vi "TLB Native Dynamic Events ver 0.23.vi"() -> ()   [LabVIEW 2018]
uses:
  Labview Training Phase 2/Enum Controls/States for Action Engine.ctl
  TLB Type Definitions/State Type Definitions, for 0.26g versions and later 2.ctl
  TLB Type Definitions/Intruction Type Definitions.ctl
  TLB Type Definitions/Encoder cluster.ctl
  TLB Type Definitions/PING CLUSTER.ctl
  <vilib>/Studica/Studica Toolkit/NavX/NavX.lvlib
  <vilib>/Studica/Studica Toolkit/Background/DIO Channel.ctl
  Underlying VI's/NavX VI/navX type def.ctl
  <vilib>/Studica/Studica Toolkit/Background/I2C Channel.ctl
  TLB Type Definitions/Vision cluster.ctl
  <vilib>/NI_Real-Time Target Support.lvlib
  TLB Type Definitions/Stepper cluster.ctl
  Experimental VI's/Archived VI's/MOTOR CONTROL NO PID Type Def.ctl
  Underlying VI's/I2C Master VI/I2C MASTER Type Def.ctl
  Underlying VI's/I2C Master VI/I2C_MASTER_WRITE_NEW Type Def.ctl
  <vilib>/userdefined/High Color/IMAQdx.ctl
  Underlying VI's/I2C Master VI/Arduino_Interfacing.ctl
  TLB Type Definitions/Yaw Cluster.ctl
  TLB Type Definitions/Time cluster.ctl
  TLB Type Definitions/Y Stepper cluster.ctl
  Underlying VI's/Modified webcam FGV/Webcam AE.ctl
  Underlying VI's/Elasped Timer/Elapsed timer control.ctl
  Underlying VI's/Motor Control VI with PID/MOTOR CONTROL WITH PID AE DATA MODE TYPE DEF.ctl
  Underlying VI's/Motor Control VI with PID/MOTOR CONTROL WITH PID AE DIRECTION TYPE DEF.ctl
  TLB Type Definitions/IR Sensor Type Def.ctl
  <vilib>/myRIO/Common/Instrument Driver Framework/myRIO v1.0/AI/typedefs/AI Channels Enum.ctl
  <vilib>/myRIO/Common/Instrument Driver Framework/myRIO v1.0/AI/typedefs/AI Channels List.ctl
  TLB Type Definitions/Motor Speed Cluster.ctl
  Underlying VI's/IMAQ Create Reference AE/IMAQ Reference AE.ctl
  TLB Type Definitions/Line Sensor Cluster.ctl
  Underlying VI's/Line Sensor AE/Line Sensor AE Type Def.ctl
  <vilib>/Studica/Studica Toolkit/NavX/TypeDefs/Flags/Z900_navX_Flags_CalibrationStatusTypeDef.ctl
  <vilib>/Studica/Studica Toolkit/NavX/TypeDefs/Flags/Z900_navX_Flags_OpStatusTypeDef.ctl
panel:
  out "Front Wall detected":bool
  out "CPU 1 Usage":dbl
  out "CPU 0 Usage":dbl
  out "Line sensors":T1
  out "IR Sensors":T2
  out "Time up":T3
  out "NAVX Values":T4
  out "Stepper position values":T5
  out "Encoder values":T6
  out "Ultrasonic sensors":T7
  out "Stop?":bool
  out "Selected Task":T8=enum."Start Task 9"
  out "Object recognition mode":enum16{"Ball", "Soap", "Gel", "Pipe", "None"}(ring)
  out "Correcte stepper":u8
  out "Image Processing Error":errorcluster
  out "Object Detection":T9
  out "Status":T12 {"OP Status" items=["INITIALIZING", "SELFTEST_IN_PROGRESS", "ERROR", "IMU_AUTOCAL_IN_PROGRESS", "NORMAL"]; "Calibration Status" items=["IMU_CAL_STATE_MASK"=3, "IMU_CAL_STATE_INPROGRESS"=0, "IMU_CAL_STATE_ACCUMULATE"=1, "IMU_CAL_STATE_COMPLETE"=2]}
  out "General Errors":errorcluster
  in  "Red LED":bool
  out "Table obstruct":bool
  out "x-y":dbl
  out "Obstacle detected":bool
  out "Speed & distance":T13
  out "Task selection":u8
  out "NavX Readings":T14
  out "Arduino Data":T15
  out "TASK ENABLE":bool
  out "Rising Edge":bool
  in  "Green LED":bool
  out "State Logic":T16=enum."Startup"
  out "elements":T8[](array[typedef])
  in  "STOP TASK":bool
  in  "OK Button":bool
  in  "STOP":bool
  out "Queue Errors":errorcluster
  out "Action Queue Items":i32
  out "State Logic Queue Items":i32
  out "Action Queues items":string[](array[string])=["Hardware reset", "Software reset", ""]
  out "Action State":string
  # "VISION"
  # "TLB FRAMEWORK STATUS"
  # "System Health Status Update"
  # "Test Programme written by Calvin Loke    Dated: 28 Aug 2019\nTest Programme revised by Dr Alex See   Dated 30 Aug 2019\n\nRevision date: 20/03/2020\nProgramme version:   TLB Native Dynamic Events ver 0.19a"
  # "0: Task 1\n1: Task 2\n2: Task 3\n3: Task 4\n4: Task 5\n5: Task 6\n6: Task 7\n7: Task 8 Ball\n8: Task 8 Soap\n9: Task 8 Gel\n10: Task 8 Pipe\n11: Task 9 Blue\n12: Task 9 Black\n13: Task 9 Green\n14: Task 9 Red\n15: Task 9 Yellow"
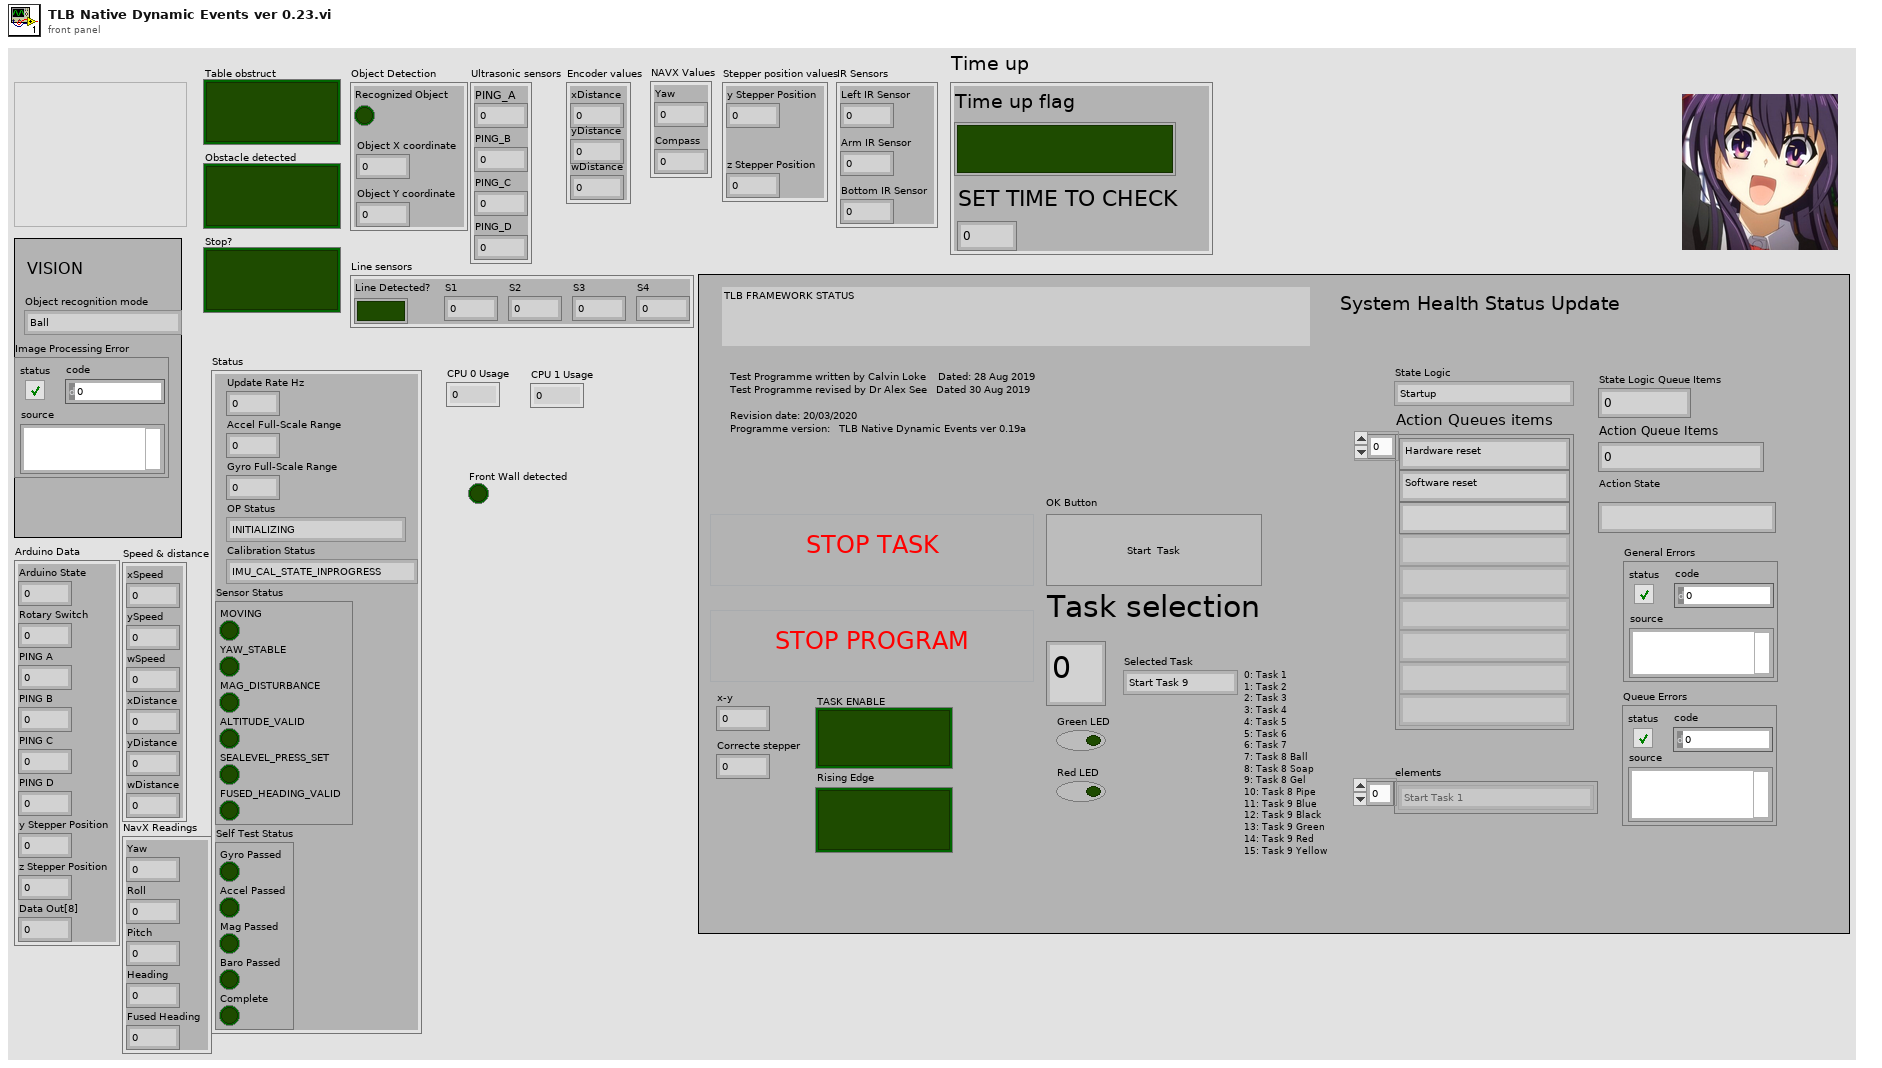
[diagram p1: front panel]
types:
  T1 = typedef "Line Sensor Cluster.ctl" = cluster{"Line Detected?":bool, "S1":dbl, "S2":dbl, "S3":dbl, "S4":dbl}
  T2 = typedef "IR Sensor Type Def.ctl" = cluster{"Left IR Sensor":dbl, "Arm IR Sensor":dbl, "Bottom IR Sensor":dbl}
  T3 = typedef "Time cluster.ctl" = cluster{"Time up flag":bool, "SET TIME TO CHECK":dbl}
  T4 = typedef "Yaw Cluster.ctl" = cluster{"Yaw":dbl, "Compass":dbl}
  T5 = typedef "Stepper cluster.ctl" = cluster{"y Stepper Position":u8, "z Stepper Position":u8}
  T6 = typedef "Encoder cluster.ctl" = cluster{"xDistance":dbl, "yDistance":dbl, "wDistance":dbl}
  T7 = typedef "PING CLUSTER.ctl" = cluster{"PING_A":u8, "PING_B":u8, "PING_C":u8, "PING_D":u8}
  T8 = typedef "Intruction Type Definitions.ctl" = enum16{"None", "Start Task 1", "Start Task 2", "Start Task 3", "Start Task 4", "Start Task 5", "Start Task 6", "Start Task 7", "Start Task 8 - BALL", "Start Task 8 - Gel", "Start Task 8 - Pipe", "Start Task 8 - Soap", "Start Task 9", "Start Task A", "Start Task B", "Exit"}
  T9 = typedef "Vision cluster.ctl" = cluster{"Recognized Object":bool, "Object X coordinate":dbl, "Object Y coordinate":dbl}
  T10 = typedef "NavX.lvlib/Z900_navX_Flags_OpStatusTypeDef.ctl" = u8
  T11 = typedef "NavX.lvlib/Z900_navX_Flags_CalibrationStatusTypeDef.ctl" = u8
  T12 = cluster{"Update Rate Hz":u8, "Accel Full-Scale Range":u8, "Gyro Full-Scale Range":u16, "OP Status":T10, "Calibration Status":T11, "Sensor Status":cluster{"MOVING":bool, "YAW_STABLE":bool, "MAG_DISTURBANCE":bool, "ALTITUDE_VALID":bool, "SEALEVEL_PRESS_SET":bool, "FUSED_HEADING_VALID":bool}, "Self Test Status":cluster{"Gyro Passed":bool, "Accel Passed":bool, "Mag Passed":bool, "Baro Passed":bool, "Complete":bool}}
  T13 = cluster{"xSpeed":dbl, "ySpeed":dbl, "wSpeed":dbl, "xDistance":dbl, "yDistance":dbl, "wDistance":dbl}
  T14 = cluster{"Yaw":dbl, "Roll":dbl, "Pitch":dbl, "Heading":dbl, "Fused Heading":dbl}
  T15 = cluster{"Arduino State":u8, "Rotary Switch":u8, "PING A":u8, "PING B":u8, "PING C":u8, "PING D":u8, "y Stepper Position":u8, "z Stepper Position":u8, "Data Out[8]":u8}
  T16 = typedef "State Type Definitions, for 0.26g versions and later 2.ctl" = enum16{"None", "Startup", "Move to Angle", "True Stop", "Idle", "Shutdown", "Task 1A", "Task 1B", "Task 2:Raise Arm", "Task 2:Sensor Mode", "Task 2:Reverse Mode", "Task 3", "Task 4_A", "Task 4_B", "Task 4_C", "Task 4_D", "Task 5A", "Task 5B", "Task 5C", "Task 5D", "Task 5E: POSITION ARM", "Task 5F: ARM GRAB HEIGHT", "Task 5G: CLOSE CLAW", "Task 5H: RAISE ARM", "Task 6_A", "Task 6_B", "Task 7", "Task 8A: RAISE ARM", "Task 8B: MOVE TO BOX", "Task 8C: CAM BURST", "Task 8D: PROCESS IMAGE", "Task 8E: ROBOT ADJUST", "Task 8F: CAM BURST 2", "Task 8G: PROCESS IMAGE 2", "Task 8H: ARM ADJUST", "Task 8I: ARM GRAB HEIGHT", "Task 8J: CLOSE CLAW", "Task 8K: RAISE MY SWORD", "Task 9A: Raise Arm", "Task 9B: Rotate to Angle", "Task 9C: Detect Box", "Task 9D: MOVE FORWARD", "Task 9E: MOVE LEFT", "Task 9F: SCAN BOX", "Task 9G: MOVE RIGHT", "Task 9H: SCAN BOX 2", "Task 9I: ROTATE 90 CW", "Task 9J: FORWARD", "Task 9K: MOVE RIGHT", "Task 9L: SCAN BOX 3", "Task 9M: MOVE RIGHT", "Task 9N: SCAN BOX 4", "PENIS", "PENIS 2", "PENIS 3", "Task 9R: PROCESS COLOUR", "Task A1: Task 9 Open cam", "Task A2: Task 9 Move Arm", "Task A3: Task 9 Set Timer", "Task A4: Tasl 9 Capture images", "Task A5: Task 9 Close camera", "Task A6: Process Colour", "Task A7: Dispose Camera Buffer"}
  T17 = typedef "Motor Speed Cluster.ctl" = cluster{"ySpeed":dbl, "xSpeed":dbl, "wSpeed":dbl}
  T18 = typedef "Y Stepper cluster.ctl" = cluster{"yStepper desired":u8}
  T19 = typedef "DIO Channel.ctl" = enum16{"Not Connected", "A/DIO1", "A/DIO2", "A/DIO3", "A/DIO4", "A/DIO5", "A/DIO6", "A/DIO7", "A/DIO13", "B/DIO1", "B/DIO2", "B/DIO3", "B/DIO4", "B/DIO5", "B/DIO6", "B/DIO7", "B/DIO13", "C/DIO0", "C/DIO1", "C/DIO2", "C/DIO3", "C/DIO4", "C/DIO5", "C/DIO6", "C/DIO7"}
  T20 = cluster{"DIO Channel":T19, "FPGA VI Reference Out":refnum<k20>}
  T21 = typedef "States for Action Engine.ctl" = enum16{"Initialize", "Write", "Read"}
  T22 = typedef "NI_Real-Time Target Support.lvlib/RT CPU Load.ctl" = cluster{"Total (%)":dbl, "Time Critical (%)":dbl, "Timed Structures (%)":dbl, "High (%)":dbl, "Above Normal (%)":dbl, "Normal (%)":dbl, "Background (%)":dbl, "Idle (%)":dbl, "ISR (%)":dbl}
  T23 = cluster{"CPU loads[0]":T22, "CPU loads[1]":T22, "CPU loads[2]":T22, "CPU loads[3]":T22, "CPU loads[4]":T22, "CPU loads[5]":T22, "CPU loads[6]":T22, "CPU loads[7]":T22, "CPU loads[8]":T22}
  T24 = typedef "navX type def.ctl" = enum16{"Get i2C reference", "Read Values", "Zero Yaw"}
  T25 = typedef "Arduino_Interfacing.ctl" = enum16{"Initialize", "Write to Arduino", "Read From Arduino"}
  T26 = typedef "I2C Channel.ctl" = enum16{"Not Connected", "A", "B"}
  T27 = cluster{"I2C Ref Out":cluster{"I2C Channel":T26, "FPGA VI Reference Out":refnum<k20>}, "Connected":bool, "Slave Address (7-bit)":u8, "Registry":u8[]}
  T28 = typedef "State Type Definitions.ctl" = enum16{"None", "Startup", "Move to Angle", "True Stop", "Idle", "Shutdown", "Task 1A", "Task 1B", "Task 2:Raise Arm", "Task 2:Sensor Mode", "Task 2:Reverse Mode", "Task 3", "Task 4_A", "Task 4_B", "Task 4_C", "Task 4_D", "Task 5A: ARM CAM HEIGHT", "Task 5B: MOVE TO BOX", "Task 5C: CAM BURST", "Task 5D: PROCESS IMAGE", "Task 5E: POSITION ARM", "Task 5F: ARM GRAB HEIGHT", "Task 5G: CLOSE CLAW", "Task 5H: RAISE ARM", "Task 6_A", "Task 6_B", "Task 7", "Task 8A: RAISE ARM", "Task 8B: MOVE TO BOX", "Task 8C: CAM BURST", "Task 8D: PROCESS IMAGE", "Task 8E: ROBOT ADJUST", "Task 8F: CAM BURST 2", "Task 8G: PROCESS IMAGE 2", "Task 8H: ARM ADJUST", "Task 8I: ARM GRAB HEIGHT", "Task 8J: CLOSE CLAW", "Task 8K: RAISE MY SWORD", "Task 9A: Raise Arm", "Task 9B: Rotate to Angle", "Task 9C: Detect Box", "Task 9D: MOVE FORWARD", "Task 9E: MOVE LEFT", "Task 9F: SCAN IMAGE", "Task 9G: PROCESS COLOUR", "Task 9H: MOVE RIGHT", "Task 9I: SCAN IMAGE", "Task 9J: PROCESS COLOUR", "Task 9K: ROTATE 90 CW", "Task 9L: MOVE FORWARD", "Task 9M: MOVE RIGHT", "Task 9N: SCAN IMAGE", "Task 9O: PROCESS COLOUR", "Task 9P: MOVE RIGHT", "Task 9Q: SCAN IMAGE", "Task 9R: PROCESS COLOUR"}
  T29 = typedef "State Type Definitions.ctl" = enum16{"None", "Startup", "Move to Angle", "True Stop", "Idle", "Shutdown", "Task 1A", "Task 1B", "Task 2:Raise Arm", "Task 2:Sensor Mode", "Task 2:Reverse Mode", "Task 3", "Task 4_A", "Task 4_B", "Task 4_C", "Task 4_D", "Task 5A", "Task 5B", "Task 5C", "Task 5D", "Task 5E: POSITION ARM", "Task 5F: ARM GRAB HEIGHT", "Task 5G: CLOSE CLAW", "Task 5H: RAISE ARM", "Task 6_A", "Task 6_B", "Task 7", "Task 8A: RAISE ARM", "Task 8B: MOVE TO BOX", "Task 8C: CAM BURST", "Task 8D: PROCESS IMAGE", "Task 8E: ROBOT ADJUST", "Task 8F: CAM BURST 2", "Task 8G: PROCESS IMAGE 2", "Task 8H: ARM ADJUST", "Task 8I: ARM GRAB HEIGHT", "Task 8J: CLOSE CLAW", "Task 8K: RAISE MY SWORD", "Task 9A: Raise Arm", "Task 9B: Rotate to Angle", "Task 9C: Detect Box", "Task 9D: MOVE FORWARD", "Task 9E: MOVE LEFT", "Task 9F: SCAN IMAGE", "Task 9G: PROCESS COLOUR", "Task 9H: MOVE RIGHT", "Task 9I: SCAN IMAGE", "Task 9J: PROCESS COLOUR", "Task 9K: ROTATE 90 CW", "Task 9L: MOVE FORWARD", "Task 9M: MOVE RIGHT", "Task 9N: SCAN IMAGE", "Task 9O: PROCESS COLOUR", "Task 9P: MOVE RIGHT", "Task 9Q: SCAN IMAGE", "Task 9R: PROCESS COLOUR", "Task A1: Raise Arm", "Task A2: Rotate to Angle", "Task A3: Move Forward", "Task A4: Rotate CW 90"}
  T30 = typedef "MOTOR CONTROL WITH PID AE DIRECTION TYPE DEF.ctl" = enum16{"y-axis movement", "x-axis movement", "rotation", "stop", "reset encoders"}
  T31 = typedef "MOTOR CONTROL WITH PID AE DATA MODE TYPE DEF.ctl" = enum16{"Init AE", "Write to AE", "Read from AE"}
  T32 = typedef "Line Sensor AE Type Def.ctl" = enum16{"INIT AE", "READ FROM LINE SENSORS"}
  T33 = typedef "IMAQ Reference AE.ctl" = enum16{"Initialize AE", "Get IMAQ Reference", "Dispose Processing Buffer"}
  T34 = typedef "Elapsed timer control.ctl" = enum16{"Start", "Pause", "Initialize"}
  T35 = typedef "I2C_MASTER_WRITE_NEW Type Def.ctl" = enum16{"Ultrasonic sensors", "Stepper origin", "zStepper 13.3k", "zStepper 13k", "zStepper 12k", "zStepper 11k", "zStepper 10k", "zStepper 9k", "zStepper 8k", "zStepper 7k", "zStepper 6k", "zStepper 5k", "zStepper 4k", "zStepper 3k", "zStepper 2k", "zStepper 1k", "zStepper 900", "zStepper 800", "zStepper 700", "zStepper 600", "zStepper 500", "zStepper 400", "zStepper 300", "zStepper 200", "zStepper 100", "zStepper 0", "yStepper control", "Open Claw", "Close Claw", "Soft Reset"}
  T36 = typedef "Webcam AE.ctl" = enum16{"Initialize Camera", "Open Camera", "Continuous Acquisition", "Close Camera", "Retrieve Image", "Dispose Camera Image Buffer"}
  T37 = typedef "IMAQdx.ctl" = refnum<k21>
  T38 = typedef "MOTOR CONTROL NO PID Type Def.ctl" = enum16{"Init", "Front Back", "Left Right", "Rotate", "Stop", "Latch"}
  T39 = typedef "AI Channels List.ctl" = T40[]
  T40 = typedef "AI Channels Enum.ctl" = enum16{"Not Connected", "AudioIn/Left", "AudioIn/Right", "C/AI0", "C/AI1", "A/AI0", "A/AI1", "A/AI2", "A/AI3", "A/AI4", "A/AI5", "A/AI6", "A/AI7", "B/AI0", "B/AI1", "B/AI2", "B/AI3", "B/AI4", "B/AI5", "B/AI6", "B/AI7", "AI/AI0", "AI/AI1", "AI/AI2", "AI/AI3", "A/AI0 (DIFF)", "A/AI1 (DIFF)", "A/AI2 (DIFF)", "A/AI3 (DIFF)", "B/AI0 (DIFF)", "B/AI1 (DIFF)", "B/AI2 (DIFF)", "B/AI3 (DIFF)"}
  T41 = cluster{"S1":dbl, "S2":dbl, "S3":dbl, "S4":dbl, "Array[4]":dbl, "Array[5]":dbl, "Array[6]":dbl, "Array[7]":dbl, "Array[8]":dbl}
  T42 = typedef "I2C MASTER Type Def.ctl" = enum16{"Last State", "Mode 0", "Mode 1", "Mode 2", "Mode 3", "Mode 4", "Mode 5", "Mode 6", "Mode 7", "Mode 8", "Mode 9", "Mode 10"}
  T43 = typedef "IMAQ Image.ctl" = refnum<image>
  T44 = cluster{"Number of Matches":i32, "Object detected?":bool}
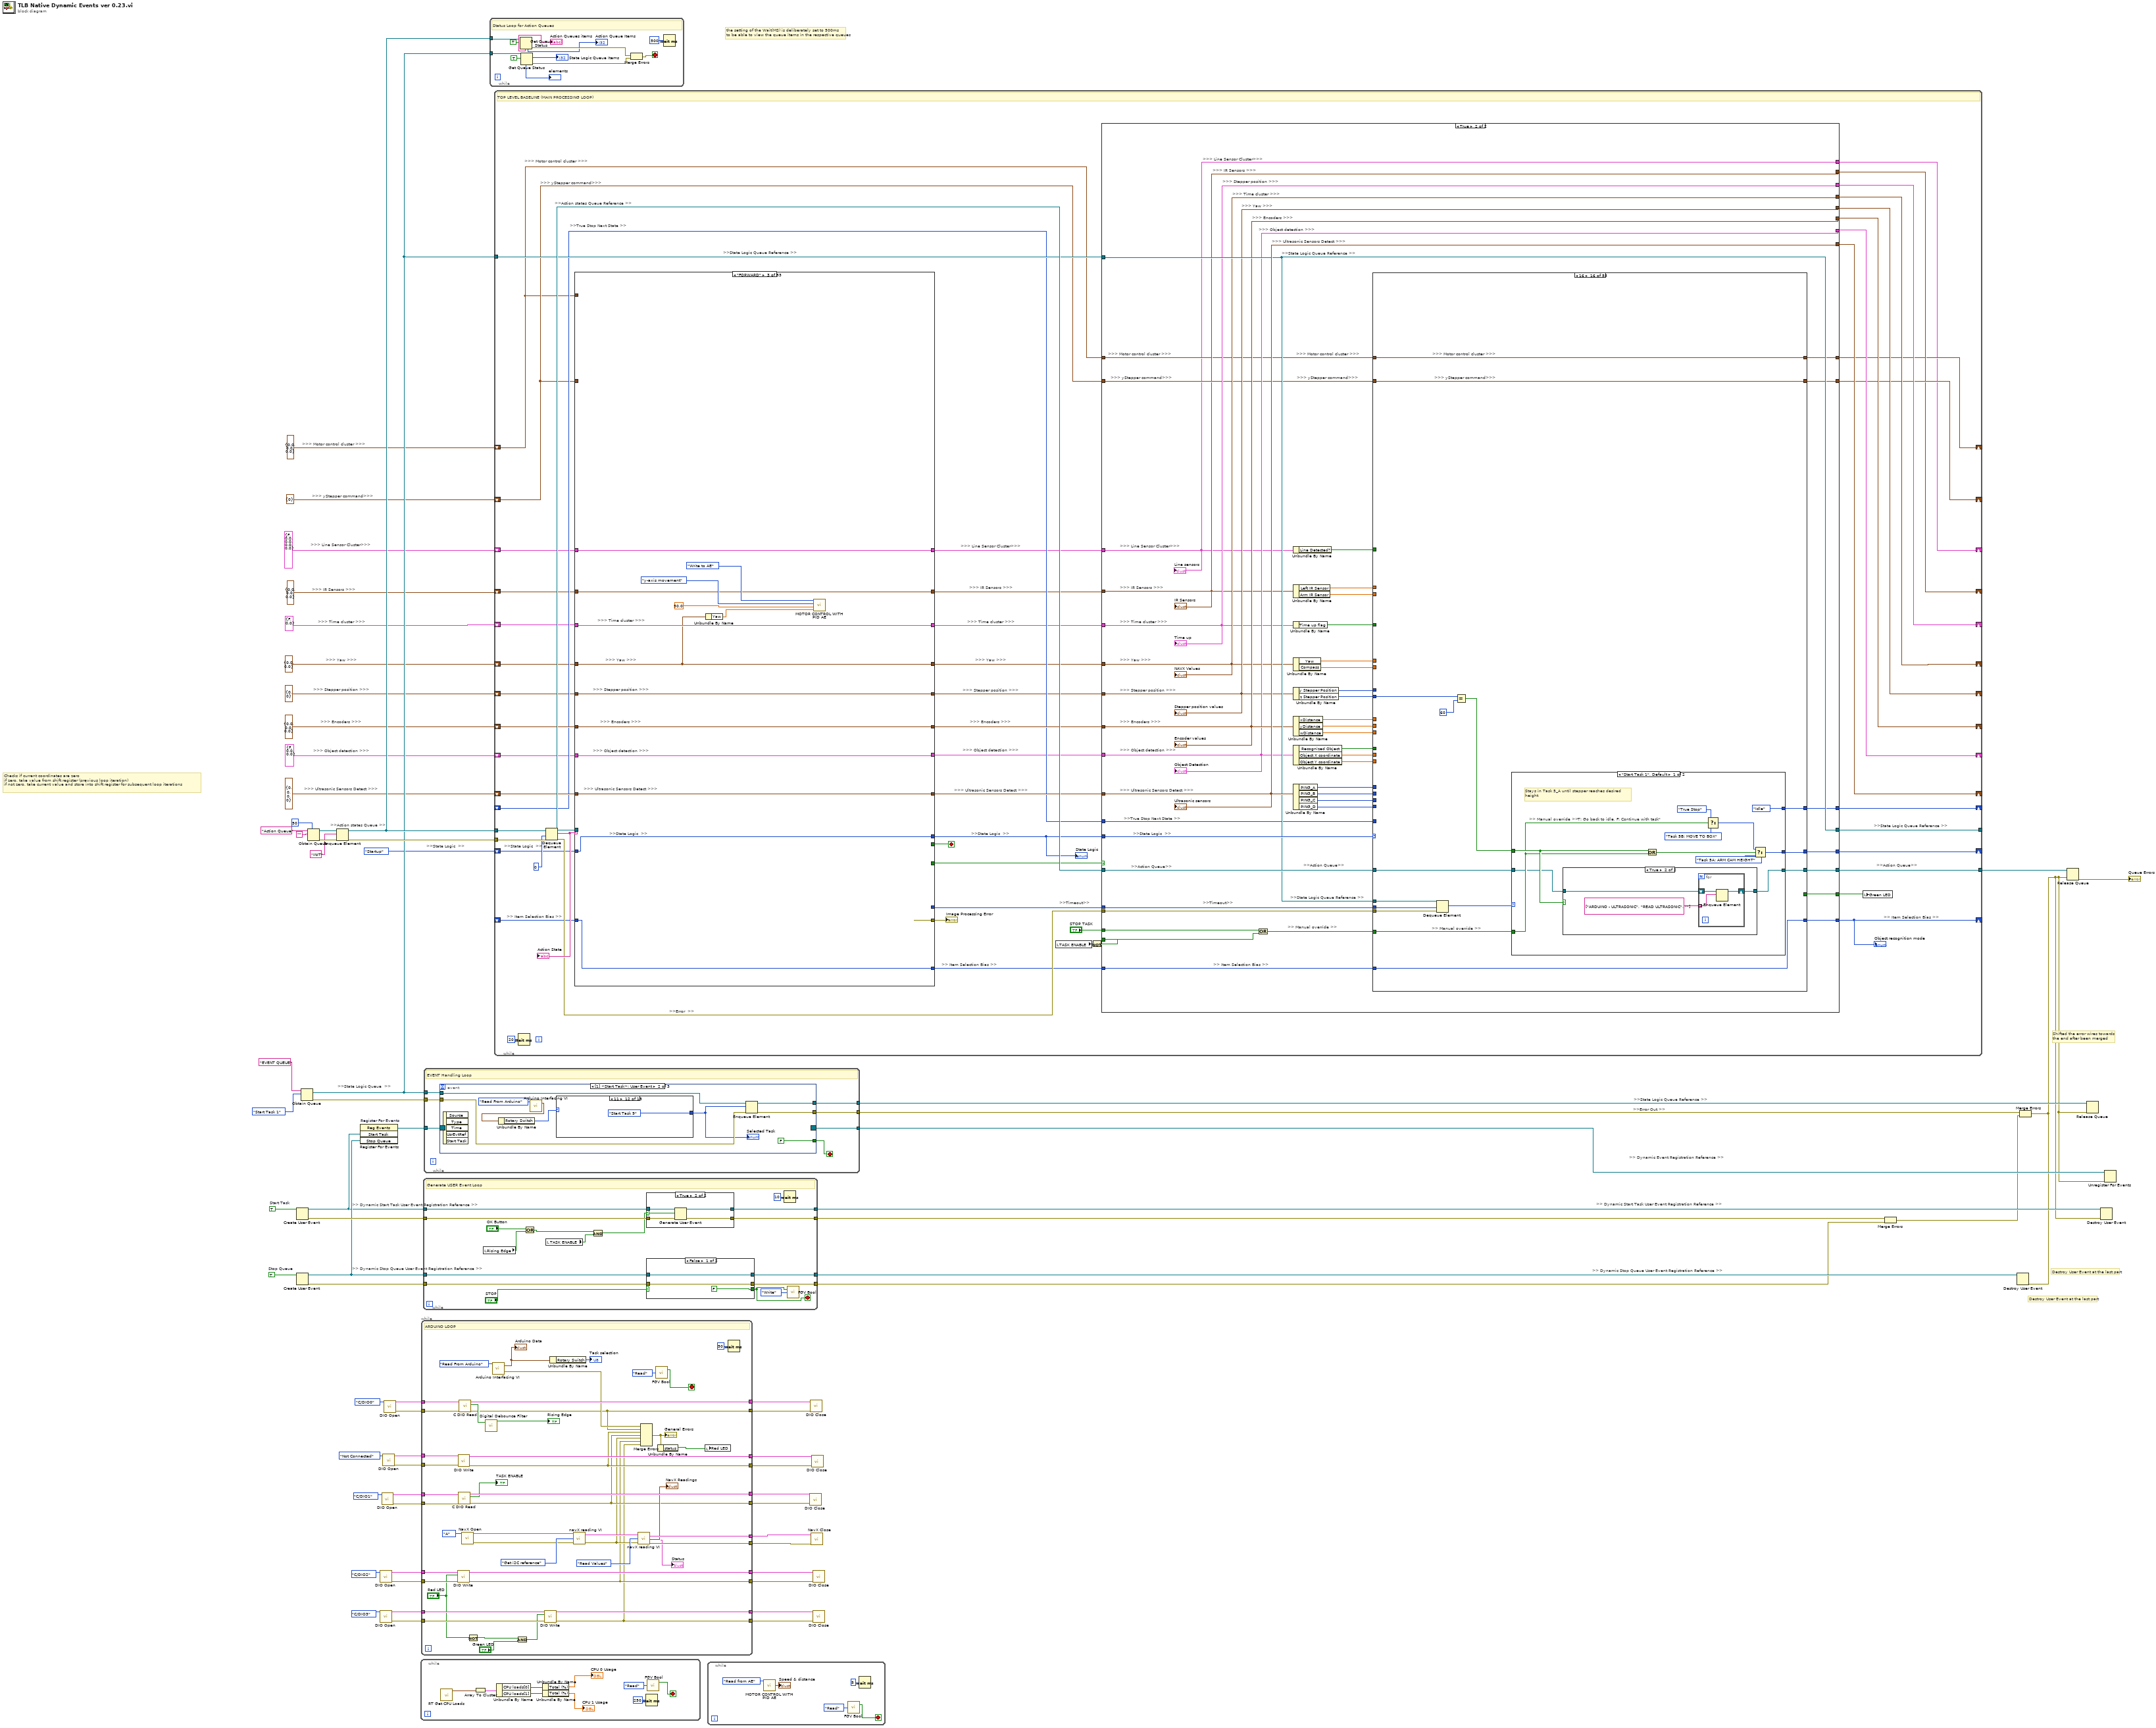
[diagram p0: block diagram]
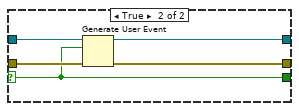
[diagram p2: hidden frame]
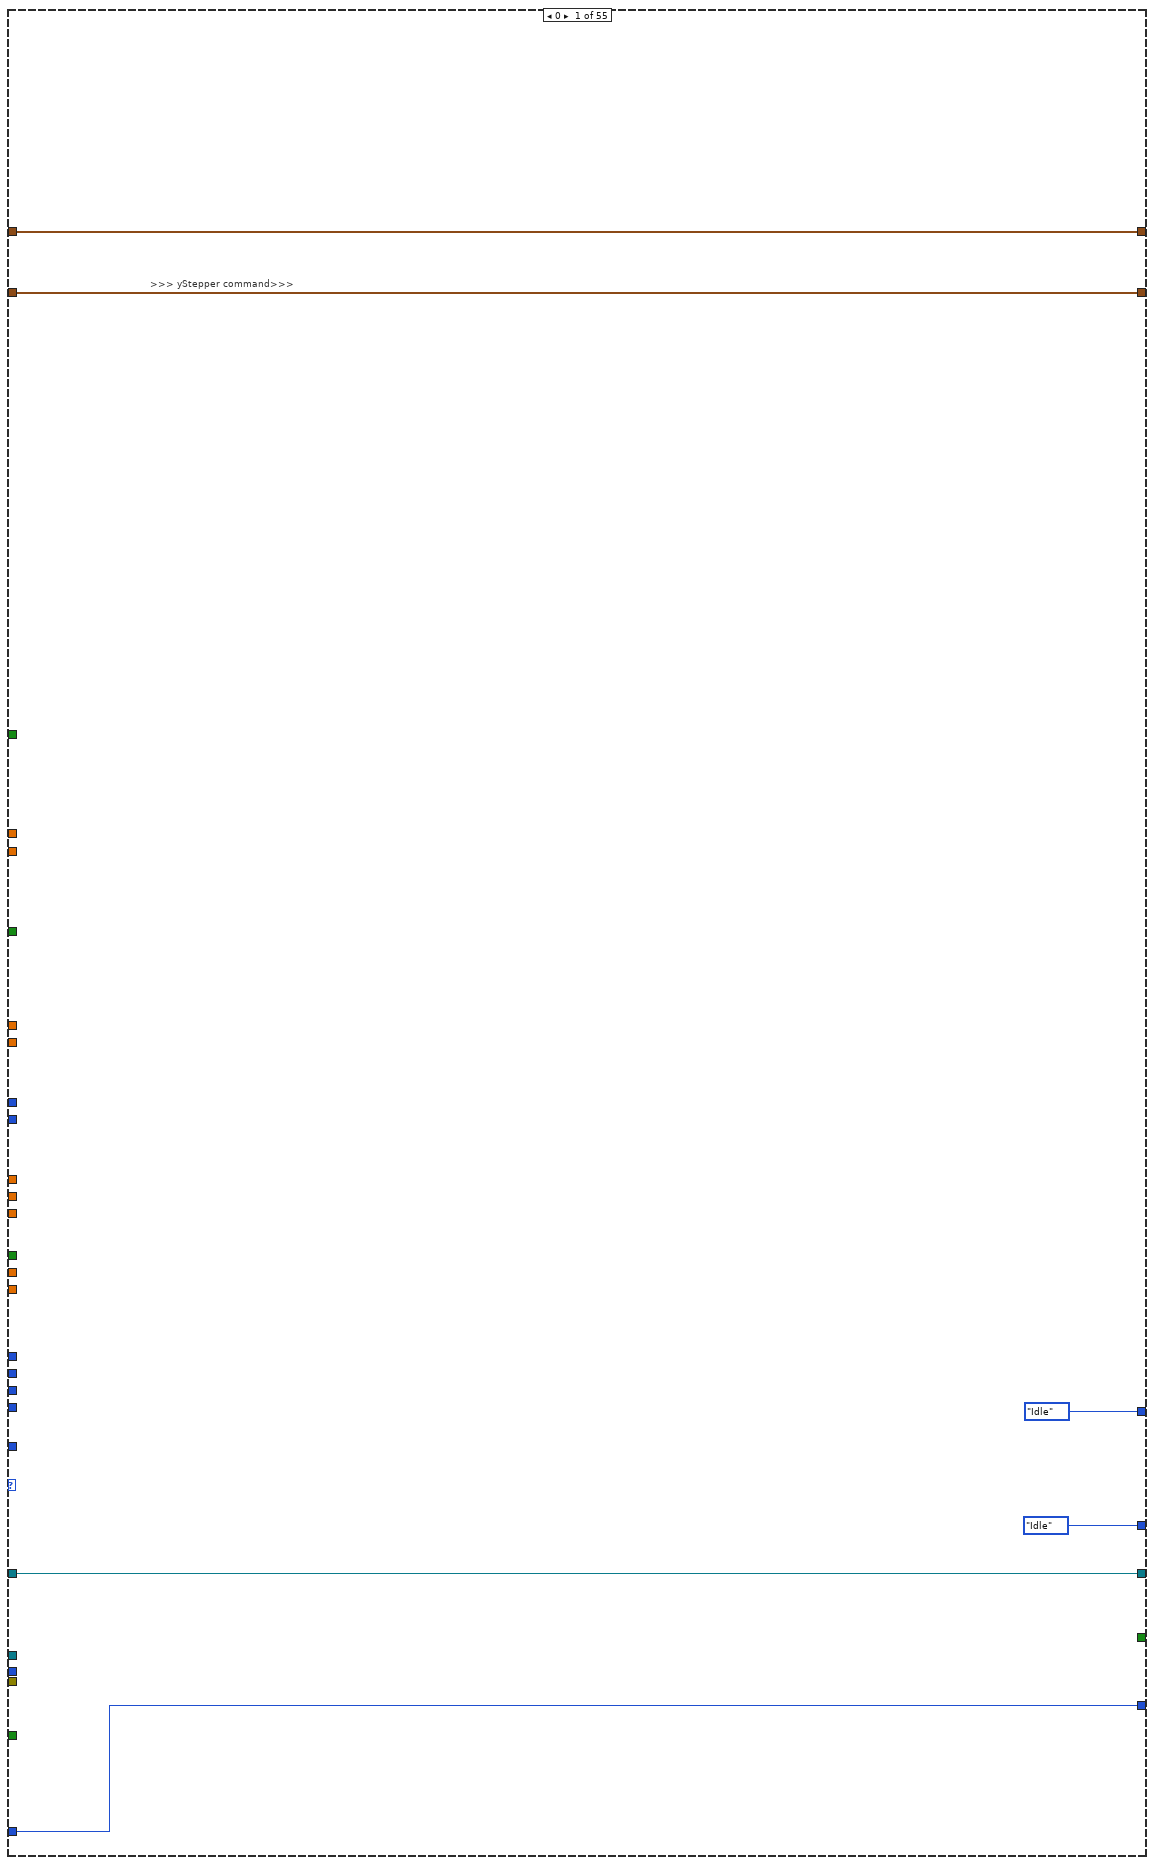
[diagram p5: hidden frame]
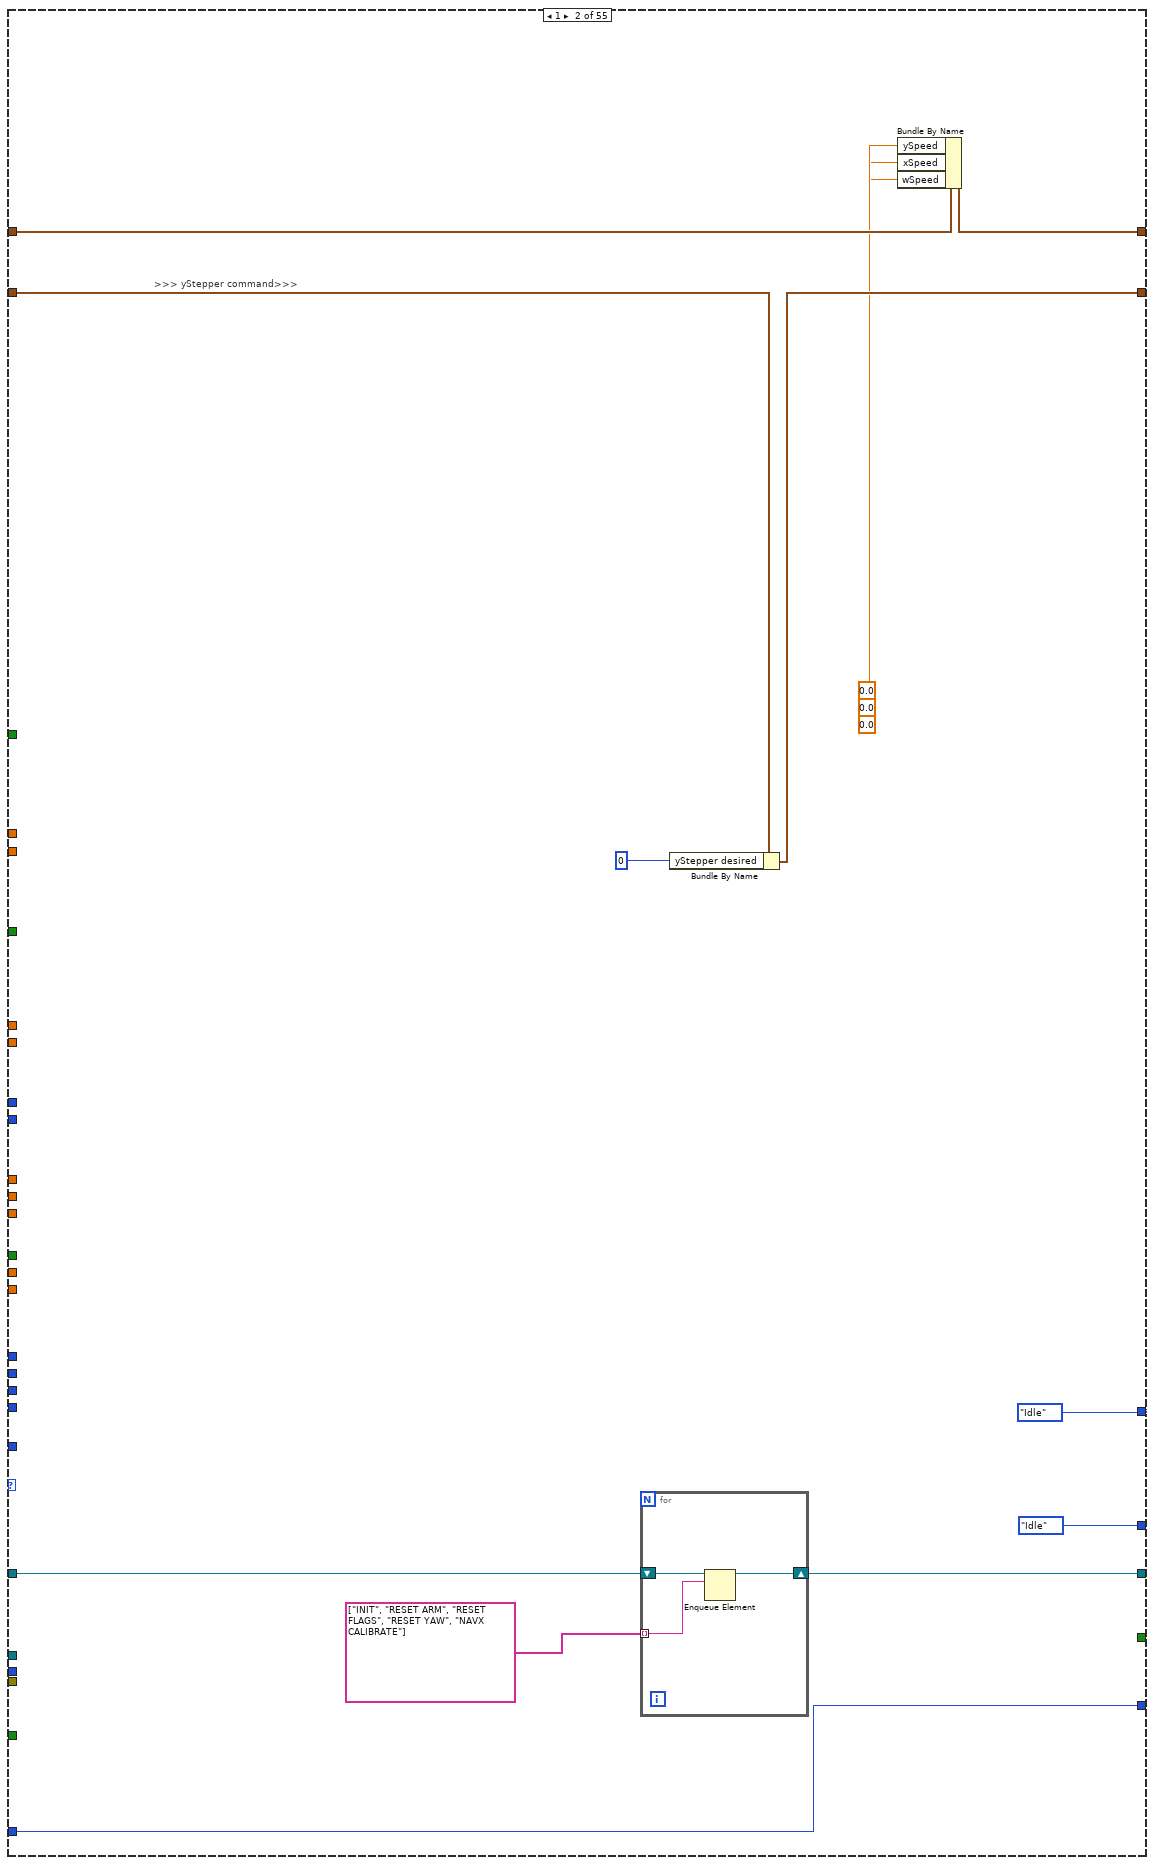
[diagram p6: hidden frame]
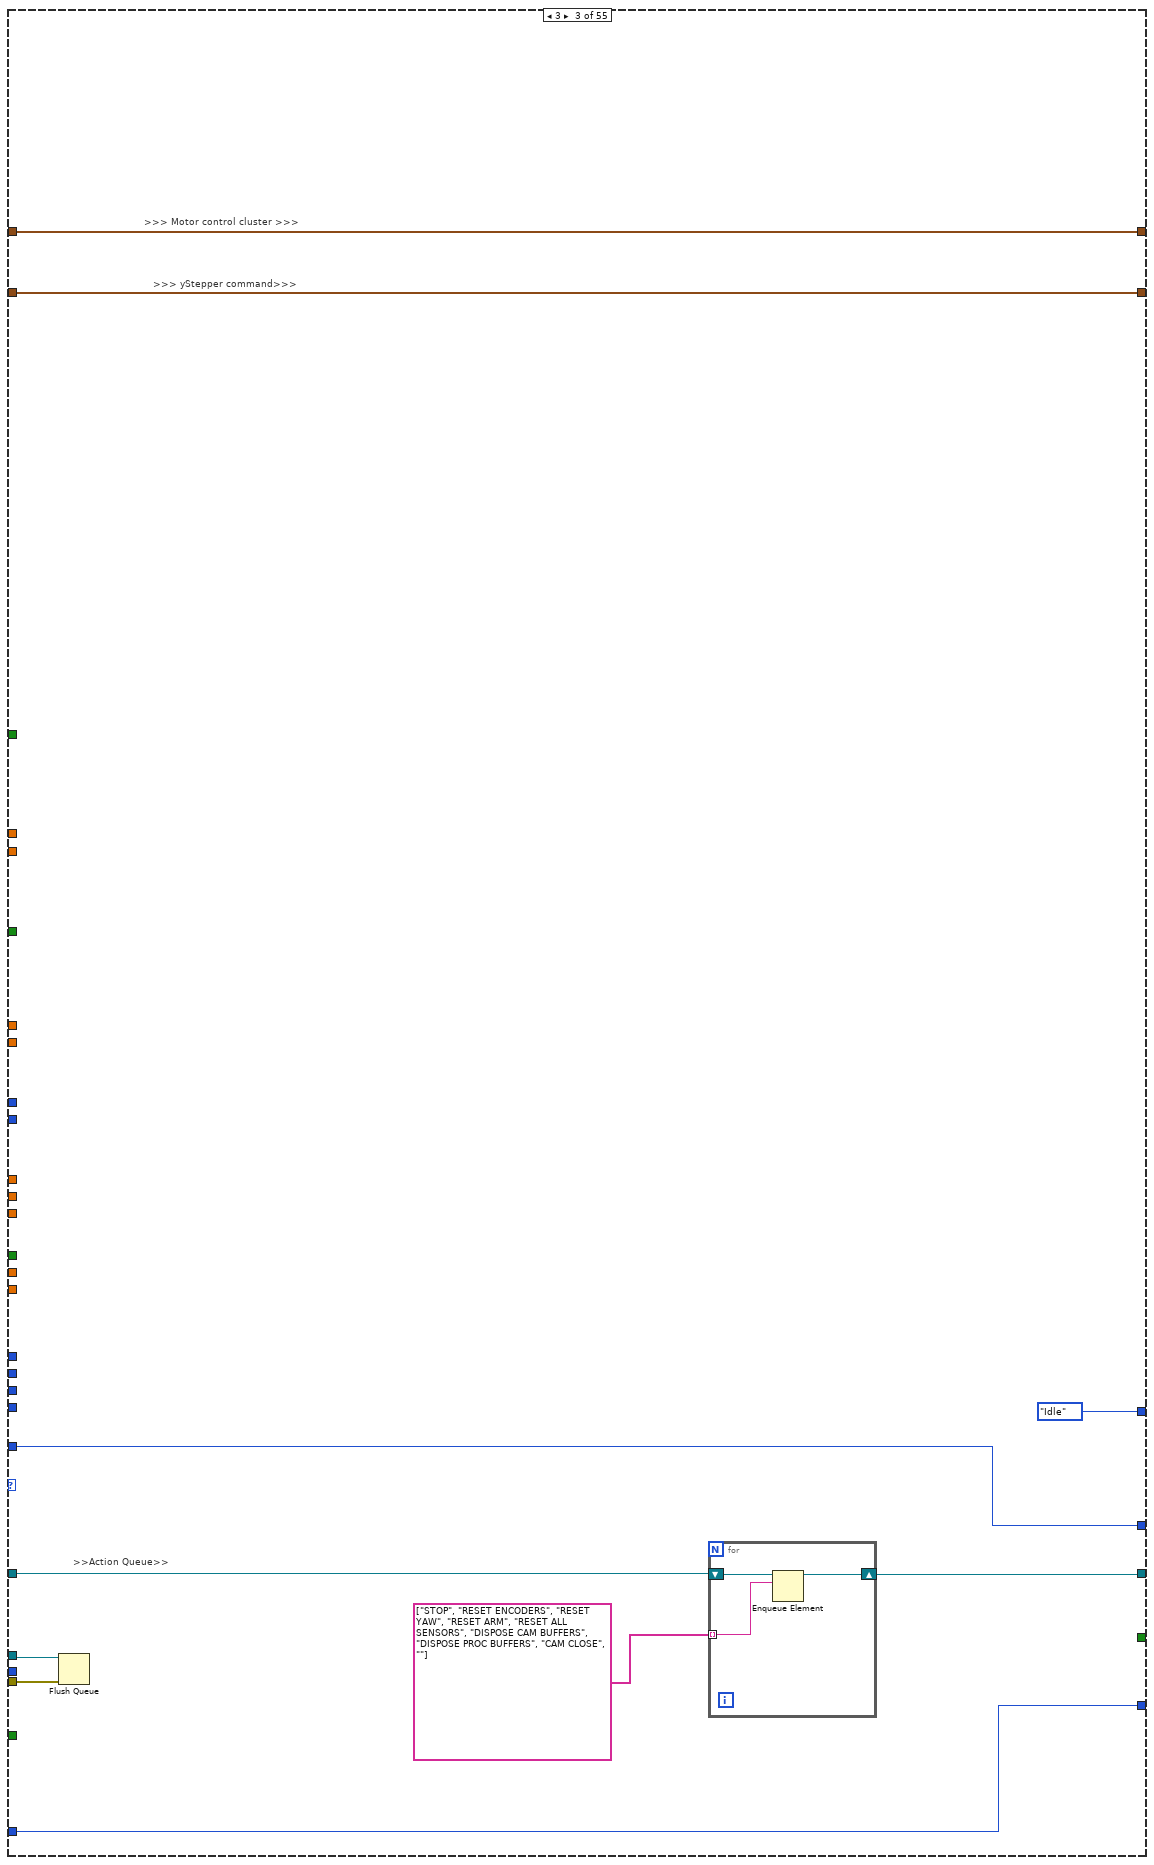
[diagram p7: hidden frame]
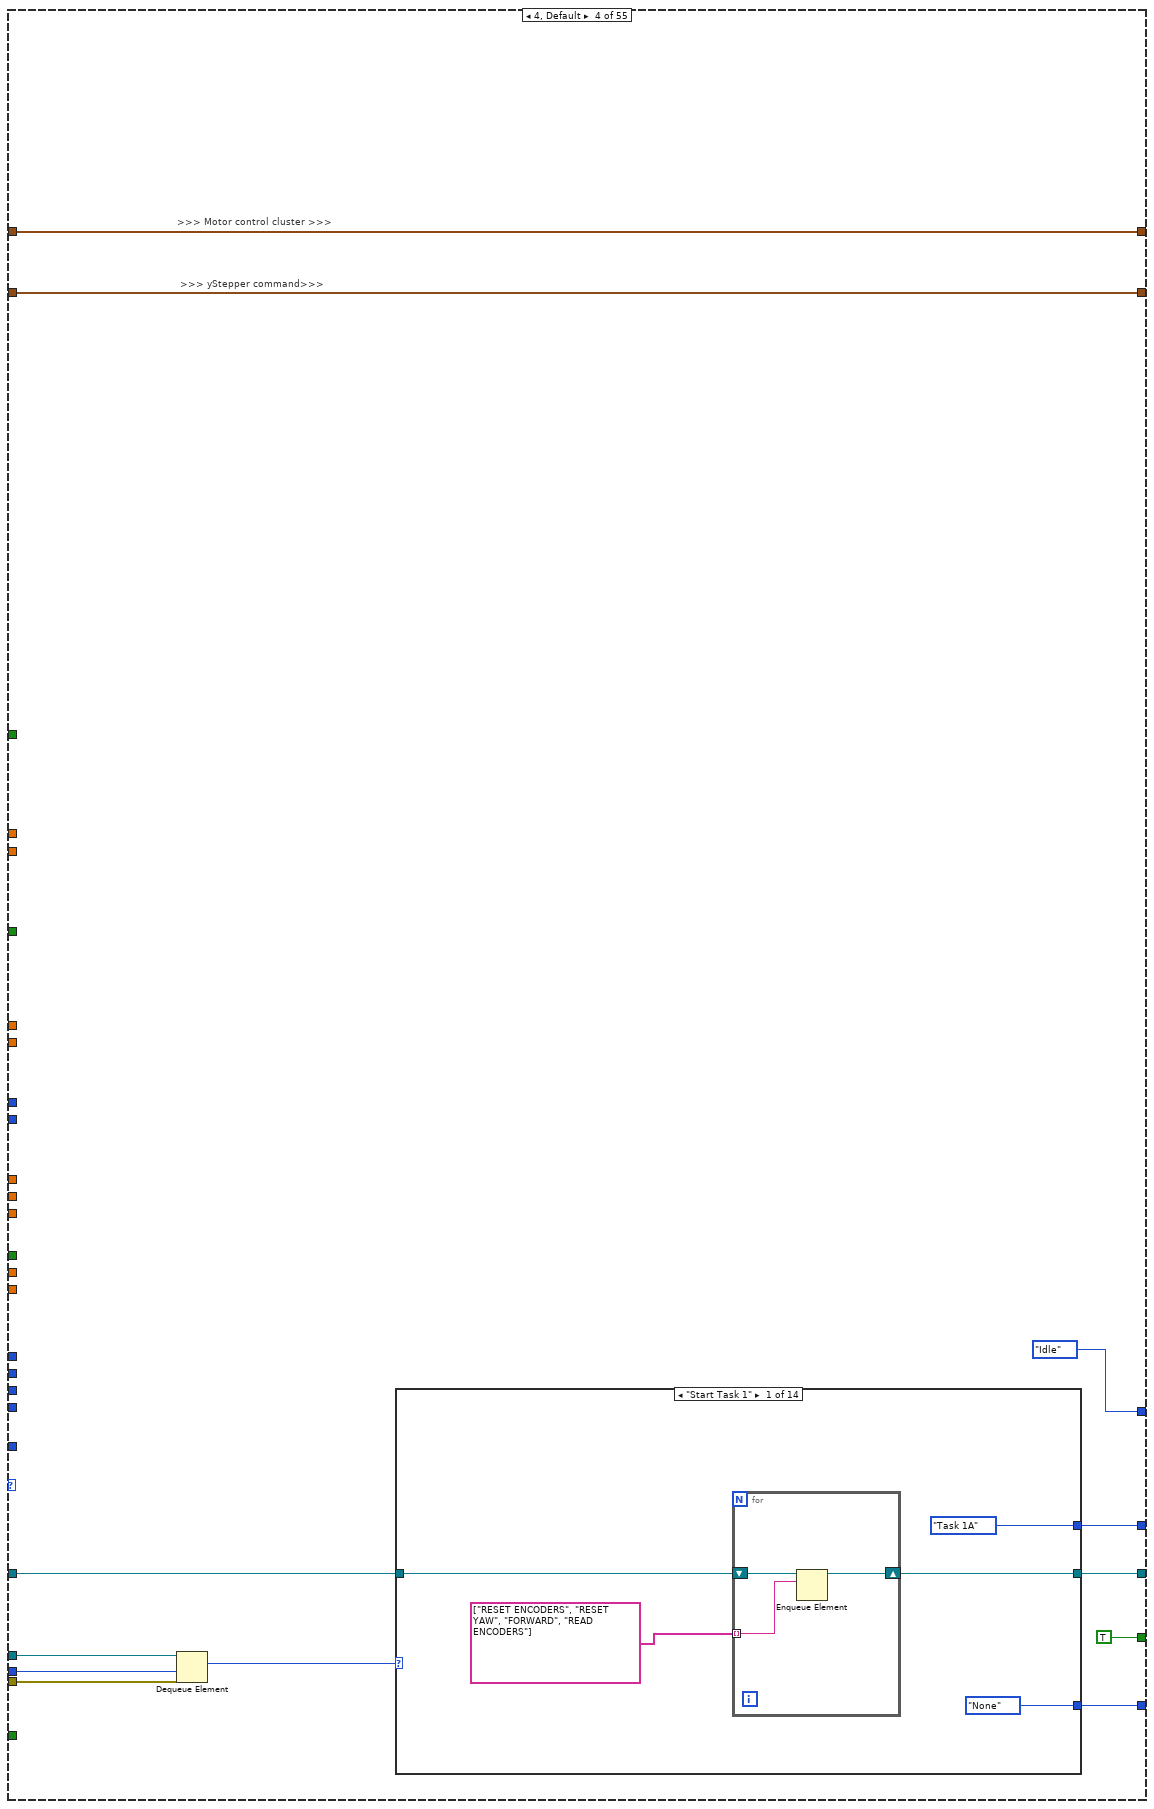
[diagram p8: hidden frame]
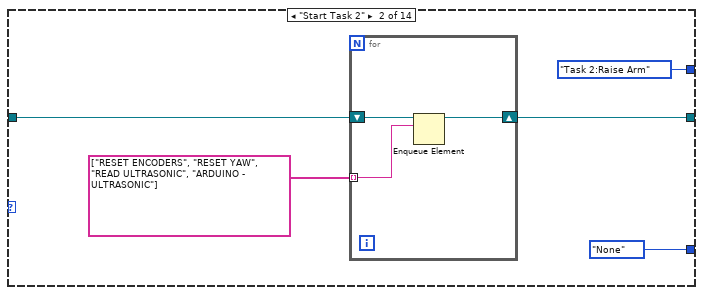
[diagram p9: hidden frame]
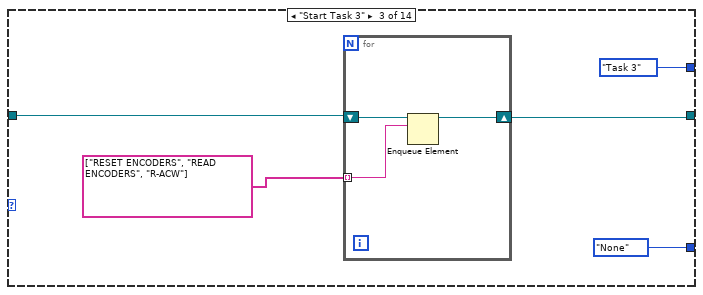
[diagram p10: hidden frame]
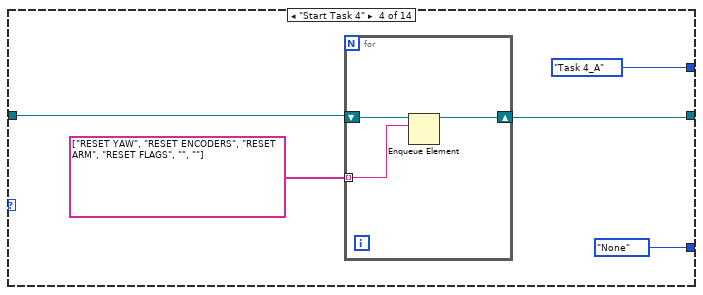
[diagram p11: hidden frame]
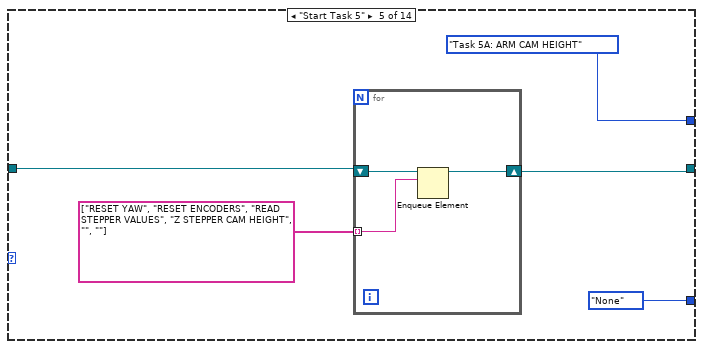
[diagram p12: hidden frame]
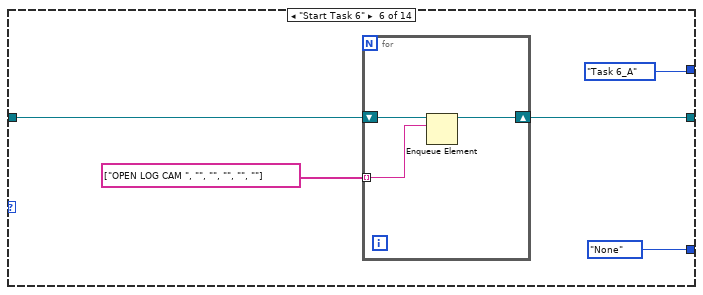
[diagram p13: hidden frame]
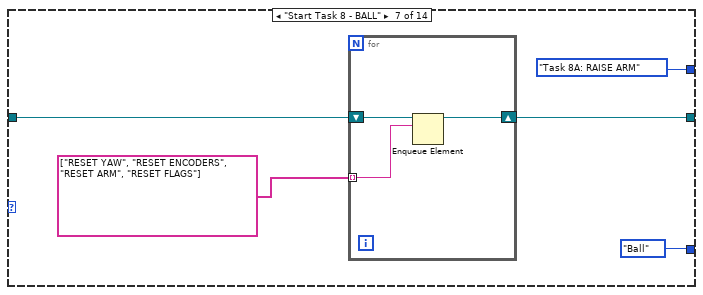
[diagram p14: hidden frame]
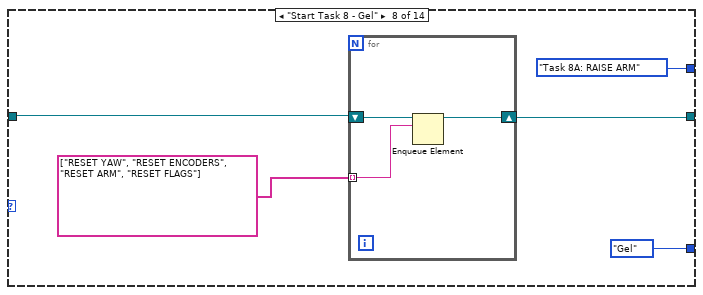
[diagram p15: hidden frame]
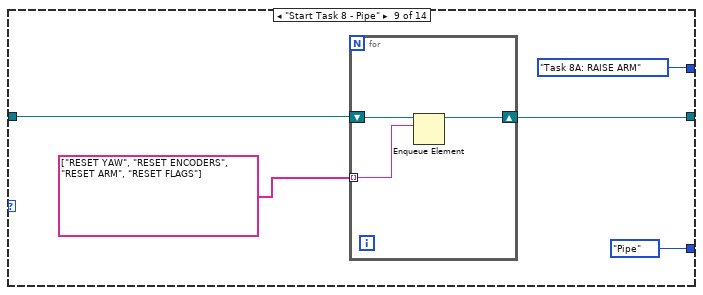
[diagram p16: hidden frame]
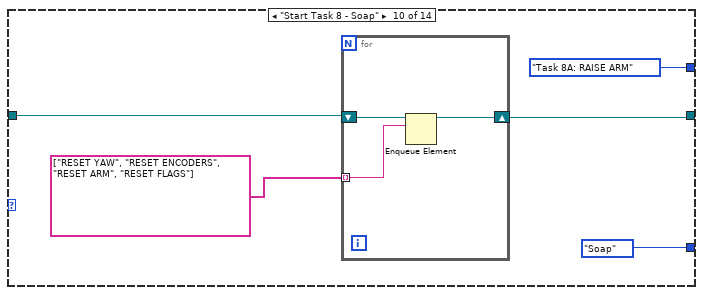
[diagram p17: hidden frame]
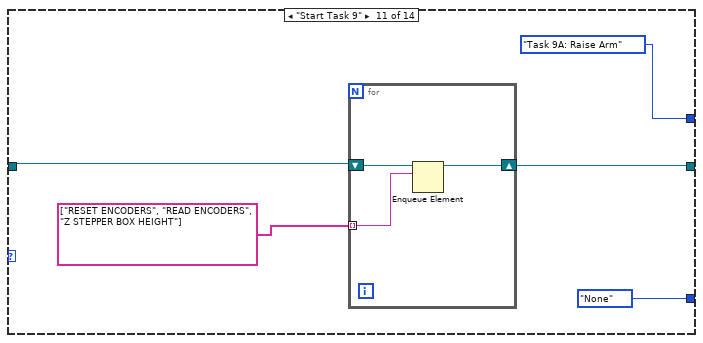
[diagram p18: hidden frame]
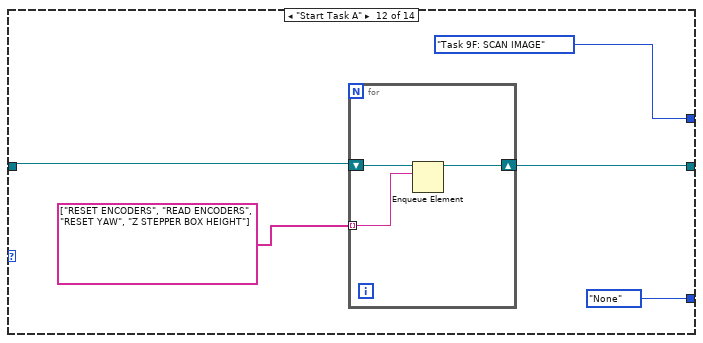
[diagram p19: hidden frame]
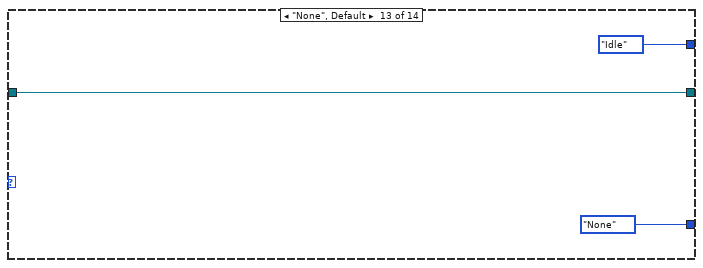
[diagram p20: hidden frame]
diagram:
  w68 = TRUE  # Stop Queue
  w67 = TRUE  # Start Task
  # ">>State Logic  >>"
  # ">>> Line Sensor Cluster>>>"
  # ">>> Motor control cluster >>>"
  # ">>> IR Sensors >>>"
  # "Checks if current coordinates are zero\nif zero, take value from shift register (previous loop iteration)\nif not zero, take current value and store into shift register for subsequent loop iterations"
  # ">>> yStepper command>>>"
  # ">>> Time cluster >>>"
  # ">>> Yaw >>>"
  # ">>> Stepper position >>>"
  # ">>> Encoders >>>"
  # ">>> Object detection >>>"
  # ">>> Ultrasonic Sensors Detect >>>"
  # "the setting of the Wait(MS) is deliberately set to 500ms\nto be able to view the queue items in the respective queues"
  # ">>Error Out >>"
  # ">> Dynamic Stop Queue User Event Registration Reference >>"
  # ">> Dynamic Start Task User Event Registration Reference >>"
  # ">> Dynamic Stop Queue User Event Registration Reference >>"
  # ">> Dynamic Start Task User Event Registration Reference >>"
  # ">> Dynamic Event Registration Reference >>"
  # ">>Action states Queue >>"
  # ">>State Logic Queue  >>"
  # ">>State Logic Queue Reference >>"
  # "Destroy User Event at the last part"
  # "Destroy User Event at the last part"
  # "Shifted the error wires towards\nthe end after been merged"
  n1 = Create User Event(user event datatype=w67) -> (user event=w59:refnum<user-event>, error out=w64:errorcluster)  [unwired: 1 in]
  n2 = Create User Event(user event datatype=w68) -> (user event=w60:refnum<user-event>, error out=w63:errorcluster)  [unwired: 1 in]
  n3 = Obtain Queue(name (unnamed)="EVENT QUEUE", element data type=Intruction_Type_Definitions."Start Task 1" ("Enum")) -> (queue out=w45:refnum<queue>, error out=w51:errorcluster)  [unwired: 3 in, 1 out]
  n4 = Obtain Queue(max queue size (-1, unlimited)=50, name (unnamed)="Action Queue", element data type="") -> (queue out=w54:refnum<queue>, error out=w50:errorcluster)  [unwired: 2 in, 1 out]
  n5 = Enqueue Element(queue=w54, element="INIT", error in (no error)=w50) -> (queue out=w46:refnum<queue>, error out=w49:errorcluster)  [unwired: 1 in, 1 out]
  n6 = register-events "Register For Events"(w59, w60) -> (reference out=w58:refnum<event-registration>)  [unwired: 2 in, 1 out]
  n7 = call <vilib>:"DIO Open.vi"("DIO Channel"=DIO_Channel."C/DIO2") -> ("error out"=w18:errorcluster, "DIO Info Out"=w19:T20)  [unwired: 9 in]
  n8 = call <vilib>:"DIO Open.vi"("DIO Channel"=DIO_Channel."C/DIO3") -> ("error out"=w13:errorcluster, "DIO Info Out"=w14:T20)  [unwired: 9 in]
  n9 = call <vilib>:"DIO Open.vi"("DIO Channel"=DIO_Channel."C/DIO1") -> ("error out"=w23:errorcluster, "DIO Info Out"=w24:T20)  [unwired: 9 in]
  n10 = call <vilib>:"DIO Open.vi"("DIO Channel"=DIO_Channel."Not Connected") -> ("error out"=w28:errorcluster, "DIO Info Out"=w30:T20)  [unwired: 9 in]
  n11 = call <vilib>:"DIO Open.vi"("DIO Channel"=DIO_Channel."C/DIO0") -> ("error out"=w33:errorcluster, "DIO Info Out"=w36:T20)  [unwired: 9 in]
  n12 = while {
    stop <- w75 stop-if-true
    n13 = call <vilib>:"RT Get CPU Loads.vi"() -> ("CPU loads"=w74:T22[])  [unwired: 10 in, 1 out]
    n14 = Array To Cluster(array=w74) -> (cluster=w73:T23)
    n15 = Unbundle By Name(w73) -> ("CPU loads[0]"=w72:T22, "CPU loads[1]"=w71:T22)
    n16 = Unbundle By Name(w72) -> ("Total (%)"=→"CPU 0 Usage":dbl)
    n17 = Unbundle By Name(w71) -> ("Total (%)"=→"CPU 1 Usage":dbl)
    n18 = Wait (ms)(milliseconds to wait=u32 250) -> ()  [unwired: 1 out]
    n19 = call "FGV Bool.vi"("Init/Read/Write State"=States_for_Action_Engine."Read") -> ("Output node"=w75:bool)  [unwired: 2 in, 1 out]
  }
  n20 = while {
    tunnel: w36 -> [w121]
    tunnel: [w120] -> w34
    tunnel: w33 -> [w119]
    tunnel: [w90] -> w32
    tunnel: w30 -> [w116]
    tunnel: [w115] -> w29
    tunnel: w28 -> [w114]
    tunnel: [w89] -> w27
    tunnel: [w113] -> w25
    tunnel: w24 -> [w112]
    tunnel: w23 -> [w111]
    tunnel: [w88] -> w22
    tunnel: w19 -> [w105]
    tunnel: w18 -> [w104]
    tunnel: [w103] -> w17
    tunnel: [w86] -> w16
    tunnel: w14 -> [w102]
    tunnel: w13 -> [w101]
    tunnel: [w100] -> w12
    tunnel: [w85] -> w11
    tunnel: [w97] -> w8
    tunnel: [w96] -> w9
    stop <- w123 stop-if-true
    # "ARDUINO LOOP"
    n21 = call <vilib>:"DIO Write.vi"("error in (no error)"=w104, "Input"="Red LED", "DIO Info In"=w105) -> ("error out"=w86:errorcluster, "DIO Info Out"=w103:T20)  [unwired: 7 in]
    n22 = call <vilib>:"DIO Write.vi"("error in (no error)"=w114, "DIO Info In"=w116) -> ("error out"=w89:errorcluster, "DIO Info Out"=w115:T20)  [unwired: 8 in]
    n23 = call <vilib>:"C DIO Read.vi"("error in (no error)"=w111, "DIO Info In in"=w112) -> ("error out"=w88:errorcluster, "IN"=→"TASK ENABLE":bool, "DIO Info In out"=w113:T20)  [unwired: 7 in]
    n24 = call <vilib>:"C DIO Read.vi"("error in (no error)"=w119, "DIO Info In in"=w121) -> ("error out"=w90:errorcluster, "IN"=w118:bool, "DIO Info In out"=w120:T20)  [unwired: 7 in]
    n25 = call <vilib>:"NavX Open.vi"("I2C Channel"=I2C_Channel."A") -> ("error out"=w107:errorcluster, "NavX Info"=w109:T27)  [unwired: 9 in]
    n26 = Not(x="Red LED") -> (.not. x?=w79:bool)
    n27 = call "Digital Debounce Filter.vi"("Boolean input"=w118) -> ("Rising Edge"=→"Rising Edge":bool)  [unwired: 1 in, 2 out]
    n28 = call "Arduino Interfacing VI.vi"("AE Mode"=Arduino_Interfacing."Read From Arduino") -> ("error out"=w91:errorcluster, "Arduino Data"=w93:T15)  [unwired: 3 in]
    "Arduino Data" <- w93
    n29 = And(x=w79, y="Green LED") -> (x .and. y?=w82:bool)
    n30 = call <vilib>:"DIO Write.vi"("error in (no error)"=w101, "Input"=w82, "DIO Info In"=w102) -> ("error out"=w85:errorcluster, "DIO Info Out"=w100:T20)  [unwired: 7 in]
    n31 = Unbundle By Name(w93) -> ("Rotary Switch"=→"Task selection":u8)
    n32 = call "navX reading VI.vi"("NavX Info In"=w109, "Mode"=navX_type_def."Get i2C reference", "error in (no error)"=w107) -> ("NavX Info Out"=w98:T27, "Error Out"=w87:errorcluster)  [unwired: 2 out]
    n33 = call "navX reading VI.vi"("NavX Info In"=w98, "Mode"=navX_type_def."Read Values", "error in (no error)"=w87) -> ("NavX Info Out"=w97:T27, "NavX Readings"=→"NavX Readings":T14, "Status"=→"Status":T12, "Error Out"=w96:errorcluster)
    n34 = Merge Errors(w91, w90, w89, w88, w87, w86, w85) -> (w83:errorcluster)
    "General Errors" <- w83
    n35 = call "FGV Bool.vi"("Init/Read/Write State"=States_for_Action_Engine."Read") -> ("Output node"=w123:bool)  [unwired: 2 in, 1 out]
    n36 = Unbundle By Name(w83) -> ("status"=w80:bool)
    n37 = local write "Red LED"(w80) -> ()
    n38 = Wait (ms)(milliseconds to wait=u32 50) -> ()  [unwired: 1 out]
  }
  n39 = while {
    tunnel: w59 -> [w141]
    tunnel: w60 -> [w140]
    tunnel: [w139] -> w66
    tunnel: [w138] -> w65
    tunnel: w64 -> [w137]
    tunnel: [w136] -> w62
    tunnel: w63 -> [w135]
    tunnel: [w134] -> w61
    stop <- w132 stop-if-true
    # "Generate USER Event Loop"
    n40 = local read "Rising Edge"() -> (w129:bool)
    n41 = Or(x="OK Button", y=w129) -> (x .or. y?=w128:bool)
    n42 = local read "TASK ENABLE"() -> (w127:bool)
    n43 = And(x=w128, y=w127) -> (x .and. y?=w126:bool)
    n44 = case shown="True" w126 {
      selector: w126 -> [_ w152]
      tunnel: w141 -> [w151 w156]
      tunnel: [w151 w155] -> w138
      tunnel: w137 -> [w150 w154]
      tunnel: [w150 w153] -> w136
      frame False {
      }
      frame True {
        n45 = Generate User Event(user event=w156, event data cluster=w152, error in=w154) -> (user event out=w155:refnum<user-event>, error out=w153:errorcluster)  [unwired: 1 in]
      }
    }
    n46 = case shown="False" "STOP" {
      selector: "STOP" -> [_ w145]
      tunnel: w140 -> [w144 w149]
      tunnel: [w144 w148] -> w139
      tunnel: w135 -> [w143 w147]
      tunnel: [w143 w146] -> w134
      tunnel: [FALSE w145] -> w132
      frame False {
      }
      frame True {
        n47 = Generate User Event(user event=w149, event data cluster=w145, error in=w147) -> (user event out=w148:refnum<user-event>, error out=w146:errorcluster)  [unwired: 1 in]
      }
    }
    n48 = Wait (ms)(milliseconds to wait=u32 10) -> ()  [unwired: 1 out]
    n49 = call "FGV Bool.vi"("Init/Read/Write State"=States_for_Action_Engine."Write", "Input Node"=w132) -> ()  [unwired: 1 in, 2 out]
  }
  n50 = while {
    tunnel: w58 -> [w163]
    tunnel: [w162] -> w57
    tunnel: w45 -> [w160]
    tunnel: [w159] -> w56
    tunnel: w51 -> [w158]
    tunnel: [w157] -> w48
    stop <- w161 stop-if-true
    # "EVENT Handling Loop"
    n51 = event shown="[1] <Start Task>: User Event" {
      selector: w163 -> [_ _ _]
      dyn-events: [_ _ _] -> w162
      timeout: _ -> [_ _ _]
      tunnel: [FALSE FALSE w197] -> w161
      tunnel: w160 -> [w168 w177 w195]
      tunnel: [w167 w176 w196] -> w159
      tunnel: w158 -> [w166 w175 w194]
      tunnel: [w165 w174 w193] -> w157
      event Timeout {
        n52 = event-data() -> ()  [unwired: 1 in, 3 out]
        n53 = Enqueue Element(queue=w168, element=Intruction_Type_Definitions."Start Task 1" ("Enum"), error in (no error)=w166) -> (queue out=w167:refnum<queue>, error out=w165:errorcluster)  [unwired: 1 in, 1 out]
      }
      event User Event {
        n54 = event-data() -> ()  [unwired: 1 in, 5 out]
        n55 = call "Arduino Interfacing VI.vi"("AE Mode"=Arduino_Interfacing."Read From Arduino") -> ("Arduino Data"=w171:T15)  [unwired: 3 in, 1 out]
        n56 = Unbundle By Name(w171) -> ("Rotary Switch"=w170:u8)
        n57 = case shown="11" w170 {
          tunnel: [Intruction_Type_Definitions."Start Task 1" ("Enum") Intruction_Type_Definitions."Start Task 2" ("Enum") Intruction_Type_Definitions."Start Task 3" ("Enum") Intruction_Type_Definitions."Start Task 4" ("Enum") Intruction_Type_Definitions."Start Task 5" ("Enum") Intruction_Type_Definitions."Start Task 6" ("Enum") Intruction_Type_Definitions."Start Task 7" ("Enum") Intruction_Type_Definitions."Start Task 8 - BALL" ("Enum") Intruction_Type_Definitions."Start Task 8 - Soap" ("Enum") Intruction_Type_Definitions."Start Task 8 - Gel" ("Enum") Intruction_Type_Definitions."Start Task 8 - Pipe" ("Enum") Intruction_Type_Definitions."Start Task 9" ("Enum") Intruction_Type_Definitions."None" ("Enum")] -> w173
          frame 0, Default {
          }
          frame 1 {
          }
          frame 2 {
          }
          frame 3 {
          }
          frame 4 {
          }
          frame 5 {
          }
          frame 6 {
          }
          frame 7 {
          }
          frame 8 {
          }
          frame 9 {
          }
          frame 10 {
          }
          frame 11 {
          }
          frame 12 {
          }
        }
        "Selected Task" <- w173
        n58 = Enqueue Element(queue=w177, element=w173, error in (no error)=w175) -> (queue out=w176:refnum<queue>, error out=w174:errorcluster)  [unwired: 1 in, 1 out]
      }
      event User Event {
        n59 = event-data() -> ("Stop Queue"=w197:bool)  [unwired: 1 in, 4 out]
        n60 = Enqueue Element At Opposite End(queue=w195, element=Intruction_Type_Definitions."Exit" ("Enum"), error in (no error)=w194) -> (queue out=w196:refnum<queue>, error out=w193:errorcluster)  [unwired: 1 in, 1 out]
      }
    }
  }
  n61 = while {
    tunnel: w46 -> [w207]
    tunnel: w45 -> [w204]
    stop <- w201 stop-if-true
    # "Status Loop for Action Queues"
    n62 = Get Queue Status(queue=w207, return elements? (F)=TRUE) -> (error out=w203:errorcluster, # elements in queue=→"Action Queue Items":i32, elements=→"Action Queues items":string[])  [unwired: 1 in, 5 out]
    n63 = Get Queue Status(queue=w204, return elements? (F)=TRUE) -> (# pending remove=→"State Logic Queue Items":i32, error out=w202:errorcluster, elements=→"elements":T8[])  [unwired: 1 in, 5 out]
    n64 = Merge Errors(w203, w202) -> (w201:errorcluster)
    n65 = Wait (ms)(milliseconds to wait=u32 500) -> ()  [unwired: 1 out]
  }
  n66 = while {
    tunnel: w45 -> [w251]
    tunnel: w46 -> [w263]
    tunnel: w49 -> [w261]
    tunnel: [w260] -> _
    tunnel: [w259] -> w39
    shift-right: [w252] -> _
    shift-left: T7 {"PING_A"=0, "PING_B"=0, "PING_C"=0, "PING_D"=0} -> [w254]
    shift-right: [w245] -> _
    shift-left: State_Type_Definitions,_for_0.26g_versions_and_later_2."Startup" ("Enum") -> [w248]
    shift-right: [w241] -> _
    shift-left: T6 {"xDistance"=0.0, "yDistance"=0.0, "wDistance"=0.0} -> [w243]
    shift-right: [w238] -> _
    shift-left: _ -> [w237]
    shift-right: [w234] -> _
    shift-left: T9 {"Recognized Object"=FALSE, "Object X coordinate"=0.0, "Object Y coordinate"=0.0} -> [w236]
    shift-right: [w231] -> _
    shift-left: T5 {"y Stepper Position"=0, "z Stepper Position"=0} -> [w233]
    shift-right: [w228] -> _
    shift-left: T4 {"Yaw"=0.0, "Compass"=0.0} -> [w230]
    shift-right: [w225] -> _
    shift-left: T3 {"Time up flag"=FALSE, "SET TIME TO CHECK"=0.0} -> [w227]
    shift-right: [w223] -> _
    shift-left: T18 {"yStepper desired"=0} -> [w224]
    shift-right: [w219] -> _
    shift-left: T2 {"Left IR Sensor"=0.0, "Arm IR Sensor"=0.0, "Bottom IR Sensor"=0.0} -> [w221]
    shift-right: [w217] -> _
    shift-left: T17 {"ySpeed"=0.0, "xSpeed"=0.0, "wSpeed"=0.0} -> [w218]
    shift-right: [w214] -> _
    shift-left: T1 {"Line Detected?"=FALSE, "S1"=0.0, "S2"=0.0, "S3"=0.0, "S4"=0.0} -> [w216]
    shift-right: [w212] -> _
    shift-left: _ -> [w211]
    stop <- w250 stop-if-true
    # ">>Action Queue>>"
    # ">>State Logic Queue Reference >>"
    # ">>> Line Sensor Cluster>>>"
    # ">>> IR Sensors >>>"
    # ">>> Time cluster >>>"
    # ">>> Object detection >>>"
    # ">>> Yaw >>>"
    # ">>> Ultrasonic Sensors Detect >>>"
    # ">>> Encoders >>>"
    # ">>> Stepper position >>>"
    # ">>State Logic  >>"
    # ">> Item Selection Bias >>"
    # ">> Item Selection Bias >>"
    # ">> Item Selection Bias >>"
    # ">>State Logic  >>"
    # ">>> Motor control cluster >>>"
    # ">>> yStepper command>>>"
    # ">>True Stop Next State >>"
    # ">>Error  >>"
    # ">>Timeout>>"
    # ">>Action states Queue Reference >>"
    # ">>State Logic Queue Reference >>"
    # "TOP LEVEL BASELINE (MAIN PROCESSING LOOP)"
    n67 = Wait (ms)(milliseconds to wait=u32 20) -> ()  [unwired: 1 out]
    n68 = Dequeue Element(queue=w263, timeout in ms (-1)=0, error in (no error)=w261) -> (queue out=w255:refnum<queue>, element=w262:string, error out=w256:errorcluster)  [unwired: 1 out]
    "Action State" <- w262
    n69 = case shown="\"FORWARD\"" w262 {
      tunnel: [_ _ _ _ _ _ _ _ _ _ _ _ _ _ _ _ _ _ _ _ 0 w3078 _ _ _ _ _ _ _ _ _ _ _ _ _ _ _ _ _ _ _ _ _ _ _ _ _ _ _ _ _ _ _] -> w258
      tunnel: w255 -> [_ _ _ _ _ _ _ _ _ _ _ _ _ _ _ _ _ _ _ _ _ _ _ _ _ _ _ _ _ _ _ _ _ _ _ _ _ _ _ _ _ _ _ _ _ _ _ _ _ _ _ _ _]
      tunnel: w254 -> [w2774 w2785 w2799 w2812 w2831 w2845 w2858 w2871 w2886 w2900 w2913 w2922 w2939 w2955 w2969 w2981 w3004 w3013 w3042 w3054 w3067 w3079 w3090 w3102 w3119 w3153 w3189 w3202 w3212 w3223 w3235 w3249 w3264 w3275 w3286 w3305 w3315 w3330 w3339 w3351 w3363 w3375 w3384 w3401 w3410 w3428 w3436 w3450 w3464 w3478 w3492 w3506 w3519]
      tunnel: [w2774 w2785 w2799 w2812 w2831 w2845 w2858 w2871 w2886 w2900 w2913 w2922 w2939 w2956 w2969 w2981 w3004 w3013 w3043 w3054 w3067 w3079 w3090 w3102 w3119 w3152 w3188 w3202 w3212 w3223 w3235 w3249 w3264 w3275 w3286 w3305 w3315 w3330 w3339 w3351 w3363 w3375 w3384 w3401 w3410 w3428 w3436 w3450 w3464 w3478 w3492 w3506 w3519] -> w253
      tunnel: [TRUE TRUE _ _ _ _ _ _ _ _ _ _ _ _ _ _ _ _ _ _ _ _ _ _ _ _ _ _ _ _ _ _ _ _ _ _ _ _ _ _ _ _ _ _ _ _ _ _ _ _ _ _ _] -> w250
      tunnel: w248 -> [w2772 w2783 w2798 w2811 w2830 w2844 w2857 w2870 w2885 w2899 w2912 w2921 w2938 w2954 w2968 w2979 w2997 w3012 w3041 w3053 w3064 w3076 w3089 w3101 w3118 w3151 w3187 w3201 w3211 w3222 w3227 w3248 w3263 w3274 w3285 w3304 w3314 w3324 w3338 w3350 w3362 w3374 w3383 w3392 w3409 w3427 w3435 w3449 w3463 w3477 w3491 w3505 w3518]
      tunnel: [_ _ _ _ _ _ _ _ _ _ _ _ _ _ _ _ _ _ _ _ _ TRUE _ _ _ _ _ _ _ _ _ _ _ _ _ _ _ _ _ _ _ _ _ _ _ _ _ _ _ _ _ _ _] -> w247
      tunnel: [w2772 w2783 w2798 w2811 w2830 w2844 w2857 w2870 w2885 w2899 w2912 w2921 w2938 w2954 w2968 w2979 w2997 w3012 w3041 w3053 w3064 w3076 w3089 w3101 w3118 w3151 w3187 w3201 w3211 w3222 w3227 w3248 w3263 w3274 w3285 w3304 w3314 w3324 w3338 w3350 w3362 w3374 w3383 w3392 w3409 w3427 w3435 w3449 w3463 w3477 w3491 w3505 w3518] -> w246
      tunnel: w243 -> [w2771 w2782 w2797 w2814 w2829 w2843 w2856 w2869 w2884 w2898 w2911 w2923 w2937 w2953 w2970 w2983 w2999 w3014 w3040 w3055 w3063 w3075 w3091 w3103 w3114 w3142 w3177 w3200 w3214 w3224 w3232 w3250 w3265 w3276 w3287 w3306 w3317 w3328 w3341 w3353 w3365 w3377 w3386 w3396 w3412 w3430 w3438 w3452 w3466 w3480 w3494 w3508 w3521]
      tunnel: [w2771 w2782 w2797 w2814 w2829 w2843 w2856 w2869 w2884 w2898 w2911 w2923 w2936 w2953 w2970 w2983 w2999 w3014 w3039 w3055 w3063 w3075 w3091 w3103 w3114 w3141 w3176 w3200 w3214 w3224 w3232 w3250 w3265 w3276 w3287 w3306 w3317 w3328 w3341 w3353 w3365 w3377 w3386 w3396 w3412 w3430 w3438 w3452 w3466 w3480 w3494 w3508 w3521] -> w242
      tunnel: w236 -> [w2770 w2781 w2796 w2813 w2828 w2842 w2855 w2868 w2883 w2897 w2909 w2920 w2935 w2952 w2963 w2982 w2998 w3011 w3031 w3052 w3062 w3074 w3088 w3100 w3117 w3146 w3182 w3198 w3213 w3221 w3233 w3247 w3262 w3270 w3284 w3300 w3316 w3329 w3340 w3352 w3364 w3376 w3385 w3395 w3411 w3429 w3437 w3451 w3465 w3479 w3493 w3507 w3520]
      tunnel: [w2770 w2781 w2796 w2813 w2828 w2842 w2855 w2868 w2883 w2897 w2909 w2920 w2935 w2952 w2963 w2982 w2998 w3011 w3030 w3052 w3062 w3074 w3088 w3100 w3116 w3145 w3181 w3198 w3213 w3221 w3233 w3247 w3262 w3270 w3284 w3299 w3316 w3329 w3340 w3352 w3364 w3376 w3385 w3395 w3411 w3429 w3437 w3451 w3465 w3479 w3493 w3507 w3520] -> w235
      tunnel: w233 -> [w2769 w2780 w2795 w2815 w2827 w2841 w2854 w2867 w2882 w2896 w2908 w2919 w2934 w2951 w2971 w2984 w3000 w3010 w3036 w3051 w3061 w3073 w3087 w3099 w3113 w3137 w3172 w3197 w3210 w3220 w3231 w3246 w3261 w3273 w3283 w3307 w3318 w3327 w3337 w3349 w3361 w3373 w3387 w3397 w3413 w3426 w3439 w3453 w3467 w3481 w3495 w3509 w3522]
      tunnel: [w2769 w2780 w2795 w2815 w2827 w2841 w2854 w2867 w2882 w2896 w2908 w2919 w2934 w2951 w2971 w2984 w3000 w3010 w3035 w3051 w3061 w3073 w3087 w3099 w3113 w3136 w3171 w3197 w3210 w3220 w3231 w3246 w3261 w3273 w3283 w3307 w3318 w3327 w3337 w3349 w3361 w3373 w3387 w3397 w3413 w3425 w3439 w3453 w3467 w3481 w3495 w3509 w3522] -> w232
      tunnel: w230 -> [w2768 w2779 w2793 w2816 w2825 w2839 w2852 w2866 w2880 w2894 w2907 w2918 w2933 w2944 w2966 w2985 w3001 w3009 w3026 w3050 w3060 w3072 w3086 w3098 w3112 w3133 w3168 w3196 w3207 w3219 w3230 w3245 w3260 w3272 w3282 w3308 w3319 w3326 w3336 w3346 w3358 w3370 w3388 w3398 w3414 w3420 w3440 w3454 w3468 w3482 w3496 w3510 w3523]
      tunnel: [w2768 w2779 w2793 w2816 w2825 w2839 w2852 w2866 w2880 w2894 w2907 w2918 w2933 w2944 w2965 w2985 w3001 w3009 w3025 w3050 w3060 w3072 w3086 w3098 w3112 w3132 w3167 w3196 w3207 w3219 w3230 w3245 w3260 w3272 w3282 w3308 w3319 w3326 w3336 w3346 w3358 w3370 w3388 w3398 w3414 w3420 w3440 w3454 w3468 w3482 w3496 w3510 w3523] -> w229
      tunnel: w227 -> [w2766 w2778 w2794 w2817 w2826 w2840 w2853 w2865 w2881 w2895 w2906 w2917 w2932 w2943 w2962 w2986 w3002 w3008 w3022 w3047 w3059 w3071 w3085 w3097 w3111 w3130 w3165 w3194 w3206 w3218 w3229 w3244 w3259 w3271 w3281 w3309 w3320 w3325 w3335 w3345 w3357 w3369 w3389 w3399 w3415 w3419 w3434 w3448 w3462 w3476 w3490 w3504 w3517]
      tunnel: [w2766 w2778 w2794 w2817 w2826 w2840 w2853 w2865 w2881 w2895 w2906 w2917 w2932 w2943 w2962 w2986 w3002 w3008 w3022 w3047 w3059 w3071 w3085 w3097 w3110 w3129 w3164 w3194 w3206 w3218 w3229 w3244 w3259 w3271 w3281 w3309 w3320 w3325 w3335 w3345 w3357 w3369 w3389 w3399 w3415 w3419 w3434 w3446 w3460 w3474 w3488 w3502 w3516] -> w226
      tunnel: w224 -> [_ _ _ _ _ _ _ _ _ _ _ _ _ _ _ _ _ _ _ _ _ _ _ _ _ _ _ _ _ _ _ _ _ _ _ _ _ _ _ _ _ _ _ _ w3406 _ _ _ _ _ _ _ _]
      tunnel: [w2765 w2777 w2788 w2807 w2820 w2834 w2848 w2861 w2876 w2889 w2903 w2916 w2926 w2942 w2959 w2977 w3003 w3007 w3019 w3046 w3058 w3070 w3084 w3094 w3104 w3123 w3156 w3193 w3205 w3217 w3234 w3238 w3253 w3268 w3279 w3293 w3312 w3331 w3334 w3344 w3356 w3368 w3380 w3400 w3404 w3418 w3433 w3443 w3457 w3471 w3485 w3499 w3513] -> w220
      tunnel: w221 -> [w2765 w2777 w2788 w2807 w2820 w2834 w2848 w2861 w2876 w2889 w2903 w2916 w2926 w2942 w2959 w2978 w3003 w3007 w3019 w3046 w3058 w3070 w3084 w3094 w3104 w3124 w3157 w3193 w3205 w3217 w3234 w3238 w3253 w3268 w3279 w3293 w3312 w3331 w3334 w3344 w3356 w3368 w3380 w3400 w3404 w3418 w3433 w3443 w3457 w3471 w3485 w3499 w3513]
      tunnel: w218 -> [_ _ _ _ _ _ _ _ w2875 _ _ _ _ _ _ _ _ _ _ _ _ _ _ _ _ _ _ _ _ _ _ _ _ _ _ _ _ _ _ _ _ _ _ _ _ _ _ _ _ _ _ _ _]
      tunnel: w216 -> [w2764 w2776 w2787 w2801 w2819 w2833 w2847 w2860 w2873 w2888 w2902 w2915 w2925 w2941 w2958 w2973 w2996 w3006 w3017 w3045 w3057 w3069 w3083 w3093 w3107 w3126 w3160 w3192 w3204 w3216 w3226 w3237 w3252 w3267 w3278 w3290 w3311 w3322 w3333 w3343 w3355 w3367 w3379 w3391 w3403 w3417 w3432 w3442 w3456 w3470 w3484 w3498 w3512]
      tunnel: [w2764 w2776 w2787 w2801 w2819 w2833 w2847 w2860 w2873 w2888 w2902 w2915 w2925 w2941 w2958 w2973 w2995 w3006 w3017 w3045 w3057 w3069 w3083 w3093 w3106 w3125 w3159 w3192 w3204 w3216 w3226 w3237 w3252 w3267 w3278 w3290 w3311 w3322 w3333 w3343 w3355 w3367 w3379 w3391 w3403 w3417 w3432 w3442 w3456 w3470 w3484 w3498 w3512] -> w215
      tunnel: [_ _ _ _ _ _ _ _ _ _ _ _ _ _ _ _ _ _ _ _ _ _ _ _ _ _ _ _ _ _ _ _ _ _ _ w3289 _ _ _ _ _ _ _ _ _ _ _ _ _ _ _ _ _] -> w213
      tunnel: w211 -> [w2763 w2775 w2786 w2800 w2818 w2832 w2846 w2859 w2872 w2887 w2901 w2914 w2924 w2940 w2957 w2972 w2987 w3005 w3015 w3044 w3056 w3068 w3082 w3092 w3108 w3127 w3161 w3191 w3203 w3215 w3225 w3236 w3251 w3266 w3277 w3288 w3310 w3321 w3332 w3342 w3354 w3366 w3378 w3390 w3402 w3416 w3431 w3441 w3455 w3469 w3483 w3497 w3511]
      tunnel: [w2763 w2775 w2786 w2800 w2818 w2832 w2846 w2859 w2872 w2887 w2901 w2914 w2924 w2940 w2957 w2972 w2987 w3005 w3015 w3044 w3056 w3068 w3082 w3092 w3108 w3127 w3161 w3191 w3203 w3215 w3225 w3236 w3251 w3266 w3277 w3288 w3310 w3321 w3332 w3342 w3354 w3366 w3378 w3390 w3402 w3416 w3431 w3441 w3455 w3469 w3483 w3497 w3511] -> w210
      frame "Exit" {
        # ">>State Logic  >>"
        # ">>> Time cluster >>>"
        # ">>> Yaw >>>"
        # ">>> Stepper position >>>"
        # ">>> Encoders >>>"
        # ">>> Object detection >>>"
        # ">>> Ultrasonic Sensors Detect >>>"
        n70 = call "Imaq Dispose"("All Images? (No)"=TRUE) -> ()  [unwired: 5 in, 1 out]
      }
      frame "----Movement States----" {
        # ">>State Logic  >>"
        # ">>> Time cluster >>>"
        # ">>> Yaw >>>"
        # ">>> Stepper position >>>"
        # ">>> Encoders >>>"
        # ">>> Object detection >>>"
        # ">>> Ultrasonic Sensors Detect >>>"
      }
      frame "FORWARD" {
        # ">>State Logic  >>"
        # ">>> Time cluster >>>"
        # ">>> Yaw >>>"
        # ">>> Stepper position >>>"
        # ">>> Encoders >>>"
        # ">>> Object detection >>>"
        # ">>> Ultrasonic Sensors Detect >>>"
        n71 = Unbundle By Name(w2793) -> ("Yaw"=w2789:dbl)
        n72 = call "MOTOR CONTROL WITH PID AE.vi"("Yaw"=w2789, "Speed"=50.0, "Direction"=MOTOR_CONTROL_WITH_PID_AE_DIRECTION_TYPE_DEF."y-axis movement", "AE Mode"=MOTOR_CONTROL_WITH_PID_AE_DATA_MODE_TYPE_DEF."Write to AE") -> ()  [unwired: 1 out]
      }
      frame "FORWARD - IR ASSIST" {
        # ">>State Logic  >>"
        # ">>> Time cluster >>>"
        # ">>> Yaw >>>"
        # ">>> Stepper position >>>"
        # ">>> Encoders >>>"
        # ">>> Object detection >>>"
        # ">>> Ultrasonic Sensors Detect >>>"
        n73 = Unbundle By Name(w2807) -> ("Left IR Sensor"=w2806:dbl)
        n74 = Subtract(x=w2806, y=20.0) -> (x-y=w2804:dbl)
        n75 = Multiply(x=w2804, y=0.25) -> (x*y=w2802:dbl)
        n76 = call "MOTOR CONTROL WITH PID AE.vi"("Yaw"=w2802, "Speed"=30.0, "Direction"=MOTOR_CONTROL_WITH_PID_AE_DIRECTION_TYPE_DEF."y-axis movement", "AE Mode"=MOTOR_CONTROL_WITH_PID_AE_DATA_MODE_TYPE_DEF."Write to AE") -> ()  [unwired: 1 out]
      }
      frame "LEFT" {
        # ">>State Logic  >>"
        # ">>> Time cluster >>>"
        # ">>> Yaw >>>"
        # ">>> Stepper position >>>"
        # ">>> Encoders >>>"
        # ">>> Object detection >>>"
        # ">>> Ultrasonic Sensors Detect >>>"
        n77 = Unbundle By Name(w2825) -> ("Yaw"=w2822:dbl)
        n78 = call "MOTOR CONTROL WITH PID AE.vi"("Yaw"=w2822, "Speed"=-20.0, "Direction"=MOTOR_CONTROL_WITH_PID_AE_DIRECTION_TYPE_DEF."x-axis movement", "AE Mode"=MOTOR_CONTROL_WITH_PID_AE_DATA_MODE_TYPE_DEF."Write to AE") -> ()  [unwired: 1 out]
      }
      frame "RIGHT" {
        # ">>> Time cluster >>>"
        # ">>> Yaw >>>"
        # ">>> Stepper position >>>"
        # ">>> Encoders >>>"
        # ">>> Object detection >>>"
        # ">>> Ultrasonic Sensors Detect >>>"
        n79 = Unbundle By Name(w2839) -> ("Yaw"=w2835:dbl)
        n80 = call "MOTOR CONTROL WITH PID AE.vi"("Yaw"=w2835, "Speed"=20.0, "Direction"=MOTOR_CONTROL_WITH_PID_AE_DIRECTION_TYPE_DEF."x-axis movement", "AE Mode"=MOTOR_CONTROL_WITH_PID_AE_DATA_MODE_TYPE_DEF."Write to AE") -> ()  [unwired: 1 out]
      }
      frame "R-ACW" {
        # ">>> IR Sensors >>>"
        # ">>> Time cluster >>>"
        # ">>> Yaw >>>"
        # ">>> Stepper position >>>"
        # ">>> Encoders >>>"
        # ">>> Object detection >>>"
        # ">>> Ultrasonic Sensors Detect >>>"
        n81 = call "MOTOR CONTROL WITH PID AE.vi"("Speed"=10.0, "Direction"=MOTOR_CONTROL_WITH_PID_AE_DIRECTION_TYPE_DEF."rotation", "AE Mode"=MOTOR_CONTROL_WITH_PID_AE_DATA_MODE_TYPE_DEF."Write to AE") -> ()  [unwired: 1 in, 1 out]
      }
      frame "R-CW" {
        (unwired) -0.2 ("Speed")
        # ">>> Time cluster >>>"
        # ">>> Yaw >>>"
        # ">>> Stepper position >>>"
        # ">>> Encoders >>>"
        # ">>> Object detection >>>"
        # ">>> Ultrasonic Sensors Detect >>>"
        n82 = call "MOTOR CONTROL WITH PID AE.vi"("Speed"=-10.0, "Direction"=MOTOR_CONTROL_WITH_PID_AE_DIRECTION_TYPE_DEF."rotation", "AE Mode"=MOTOR_CONTROL_WITH_PID_AE_DATA_MODE_TYPE_DEF."Write to AE") -> ()  [unwired: 1 in, 1 out]
      }
      frame "X AXIS - SLOW" {
        # ">>> Line Sensor Cluster>>>"
        # ">>> IR Sensors >>>"
        # ">>> Time cluster >>>"
        # ">>> Yaw >>>"
        # ">>> Stepper position >>>"
        # ">>> Encoders >>>"
        # ">>> Object detection >>>"
        # ">>> Ultrasonic Sensors Detect >>>"
        n83 = Unbundle By Name(w2875) -> ("xSpeed"=w2874:dbl)
        n84 = Unbundle By Name(w2880) -> ("Yaw"=w2877:dbl)
        n85 = call "MOTOR CONTROL WITH PID AE.vi"("Yaw"=w2877, "Speed"=w2874, "Direction"=MOTOR_CONTROL_WITH_PID_AE_DIRECTION_TYPE_DEF."x-axis movement", "AE Mode"=MOTOR_CONTROL_WITH_PID_AE_DATA_MODE_TYPE_DEF."Write to AE") -> ()  [unwired: 1 out]
      }
      frame "REVERSE" {
        # ">>> Time cluster >>>"
        # ">>> Yaw >>>"
        # ">>> Stepper position >>>"
        # ">>> Encoders >>>"
        # ">>> Object detection >>>"
        # ">>> Ultrasonic Sensors Detect >>>"
        n86 = Unbundle By Name(w2894) -> ("Yaw"=w2890:dbl)
        n87 = call "MOTOR CONTROL WITH PID AE.vi"("Yaw"=w2890, "Speed"=-50.0, "Direction"=MOTOR_CONTROL_WITH_PID_AE_DIRECTION_TYPE_DEF."y-axis movement", "AE Mode"=MOTOR_CONTROL_WITH_PID_AE_DATA_MODE_TYPE_DEF."Write to AE") -> ()  [unwired: 1 out]
      }
      frame "STOP" {
        n88 = Wait (ms)(milliseconds to wait=u32 100) -> ()  [unwired: 1 out]
        n89 = call "MOTOR CONTROL WITH PID AE.vi"("Direction"=MOTOR_CONTROL_WITH_PID_AE_DIRECTION_TYPE_DEF."stop", "AE Mode"=MOTOR_CONTROL_WITH_PID_AE_DATA_MODE_TYPE_DEF."Write to AE") -> ()  [unwired: 2 in, 1 out]
      }
      frame "----SENSOR READING---- " {
      }
      frame "READ ENCODERS" {
        # ">>> Time cluster >>>"
        # ">>> Yaw >>>"
        # ">>> Stepper position >>>"
        # ">>> Object detection >>>"
        # ">>> Current encoder distance >>>"
        # ">>> Ultrasonic Sensors Detect >>>"
        n90 = call "MOTOR CONTROL WITH PID AE.vi"("AE Mode"=MOTOR_CONTROL_WITH_PID_AE_DATA_MODE_TYPE_DEF."Read from AE") -> ("Speed & distance"=w2930:T13)  [unwired: 3 in]
        n91 = Unbundle By Name(w2930) -> ("xDistance"=w2929:dbl, "yDistance"=w2928:dbl, "wDistance"=w2927:dbl)
        n92 = Bundle By Name(cluster=w2937, "xDistance"=w2929, "yDistance"=w2928, "wDistance"=w2927) -> (w2936:T6)
      }
      frame "READ ULTRASONIC" {
        (unwired) navX_type_def."Read Values" ("Mode")
        (unwired) MOTOR_CONTROL_NO_PID_Type_Def."Latch" ("Direction")
        # ">>> Line Sensor Cluster>>>"
        # ">>> IR Sensors >>>"
        # ">>State Logic  >>"
        # ">>> Time cluster >>>"
        # ">>> Ultrasonic Sensors Detect >>>"
        # ">>> Object detection >>>"
        # ">>> Encoders >>>"
        # ">>> Stepper position >>>"
        # ">>> Yaw >>>"
        n93 = call "Arduino Interfacing VI.vi"("AE Mode"=Arduino_Interfacing."Read From Arduino") -> ("Arduino Data"=w2949:T15)  [unwired: 3 in, 1 out]
        n94 = Unbundle By Name(w2949) -> ("PING A"=w2948:u8, "PING B"=w2947:u8, "PING C"=w2946:u8, "PING D"=w2945:u8)
        n95 = Bundle By Name(cluster=w2955, "PING_A"=w2948, "PING_B"=w2947, "PING_C"=w2946, "PING_D"=w2945) -> (w2956:T7)
      }
      frame "READ NAVX" {
        # ">> Item Selection Bias >>"
        # ">>State Logic  >>"
        # ">>> Line Sensor Cluster>>>"
        # ">>> IR Sensors >>>"
        # ">>> Time cluster >>>"
        # ">>> Yaw >>>"
        # ">>> Ultrasonic Sensors Detect >>>"
        # ">>> Object detection >>>"
        # ">>> Encoders >>>"
        # ">>> Stepper position >>>"
        n96 = call "navX reading VI.vi"("Mode"=navX_type_def."Read Values") -> ("NavX Readings"=w2961:T14)  [unwired: 2 in, 3 out]
        n97 = Unbundle By Name(w2961) -> ("Heading"=w2960:dbl)
        n98 = Unbundle By Name(w2961) -> ("Yaw"=w2964:dbl)
        n99 = Bundle By Name(cluster=w2966, "Yaw"=w2964, "Compass"=w2960) -> (w2965:T4)
      }
      frame "READ IR" {
        w2975 = T39 [enum."B/AI1"] items=["Not Connected", "AudioIn/Left", "AudioIn/Right", "C/AI0", "C/AI1", "A/AI0", "A/AI1", "A/AI2", "A/AI3", "A/AI4", "A/AI5", "A/AI6", "A/AI7", "B/AI0", "B/AI1", "B/AI2", "B/AI3", "B/AI4", "B/AI5", "B/AI6", "B/AI7", "AI/AI0", "AI/AI1", "AI/AI2", "AI/AI3", "A/AI0 (DIFF)", "A/AI1 (DIFF)", "A/AI2 (DIFF)", "A/AI3 (DIFF)", "B/AI0 (DIFF)", "B/AI1 (DIFF)", "B/AI2 (DIFF)", "B/AI3 (DIFF)"] ("AI Channel")
        w2980 = T39 [enum."B/AI0"] items=["Not Connected", "AudioIn/Left", "AudioIn/Right", "C/AI0", "C/AI1", "A/AI0", "A/AI1", "A/AI2", "A/AI3", "A/AI4", "A/AI5", "A/AI6", "A/AI7", "B/AI0", "B/AI1", "B/AI2", "B/AI3", "B/AI4", "B/AI5", "B/AI6", "B/AI7", "AI/AI0", "AI/AI1", "AI/AI2", "AI/AI3", "A/AI0 (DIFF)", "A/AI1 (DIFF)", "A/AI2 (DIFF)", "A/AI3 (DIFF)", "B/AI0 (DIFF)", "B/AI1 (DIFF)", "B/AI2 (DIFF)", "B/AI3 (DIFF)"] ("AI Channel")
        # ">>State Logic  >>"
        # ">>> Time cluster >>>"
        # ">>> Ultrasonic Sensors Detect >>>"
        # ">>> Object detection >>>"
        # ">>> Encoders >>>"
        # ">>> Stepper position >>>"
        # ">>> Yaw >>>"
        n100 = call <vilib>:"Sharp IR.vi"("AI Channel"=w2975) -> ("Sharp IR Distance"=w2974:dbl)  [unwired: 8 in, 2 out]
        n101 = call <vilib>:"Sharp IR.vi"("AI Channel"=w2980) -> ("Sharp IR Distance"=w2976:dbl)  [unwired: 8 in, 2 out]
        n102 = Bundle By Name(cluster=w2978, "Left IR Sensor"=w2976, "Arm IR Sensor"=w2974) -> (w2977:T2)
      }
      frame "READ LINE SENSOR" {
        # ">>> IR Sensors >>>"
        # ">>> Line Sensor Cluster>>>"
        # ">>State Logic  >>"
        # ">>> Time cluster >>>"
        # ">>> Object detection >>>"
        # ">>> Yaw >>>"
        # ">>> Ultrasonic Sensors Detect >>>"
        # ">>> Encoders >>>"
        # ">>> Stepper position >>>"
        n103 = call "Line Sensor AE.vi"("AE State"=Line_Sensor_AE_Type_Def."READ FROM LINE SENSORS") -> ("Line Detected?"=w2993:bool, "Line Sensor Raw Values"=w2992:T41)
        n104 = Unbundle By Name(w2992) -> ("S1"=w2991:dbl, "S2"=w2990:dbl, "S3"=w2989:dbl, "S4"=w2988:dbl)
        n105 = Bundle By Name(cluster=w2996, "Line Detected?"=w2993, "S1"=w2991, "S2"=w2990, "S3"=w2989, "S4"=w2988) -> (w2995:T1)
      }
      frame "----SYSTEM MODES----" {
        (unwired) I2C_MASTER_Type_Def."Last State" ("Arduino Mode")
        # ">>> Object detection >>>"
        # ">>> Yaw >>>"
        # ">>> Ultrasonic Sensors Detect >>>"
        # ">>> Encoders >>>"
        # ">>> Stepper position >>>"
      }
      frame "INIT" {
        w3037 = u8 0
        w3038 = 0.0
        # ">>> IR Sensors >>>"
        # ">>> IR Sensors >>>"
        # ">>> Line Sensor Cluster>>>"
        # ">>> Time cluster >>>"
        # ">>> Object detection >>>"
        # ">>> Yaw >>>"
        # ">>> Ultrasonic Sensors Detect >>>"
        # ">>> Encoders >>>"
        # ">>> Stepper position >>>"
        # ">>State Logic  >>"
        n106 = call "Arduino Interfacing VI.vi"("AE Mode"=Arduino_Interfacing."Initialize") -> ()  [unwired: 3 in, 2 out]
        n107 = call "FGV Bool.vi"("Init/Read/Write State"=States_for_Action_Engine."Initialize") -> ()  [unwired: 2 in, 2 out]
        n108 = call "Elasped Timer.vi"("Action"=Elapsed_timer_control."Initialize") -> ()  [unwired: 7 in, 4 out]
        n109 = call "MOTOR CONTROL WITH PID AE.vi"("AE Mode"=MOTOR_CONTROL_WITH_PID_AE_DATA_MODE_TYPE_DEF."Init AE") -> ()  [unwired: 3 in, 1 out]
        n110 = call "IMAQ Reference AE.vi"("IMAQ AE States"=IMAQ_Reference_AE."Initialize AE") -> ()  [unwired: 1 in, 2 out]
        n111 = call "Line Sensor AE.vi"("AE State"=Line_Sensor_AE_Type_Def."INIT AE") -> ()  [unwired: 2 out]
        n112 = Bundle By Name(cluster=w3031, "Recognized Object"=FALSE, "Object X coordinate"=0.0, "Object Y coordinate"=0.0) -> (w3030:T9)
        n113 = Bundle By Name(cluster=w3036, "y Stepper Position"=u8 0, "z Stepper Position"=u8 0) -> (w3035:T5)
        n114 = Bundle By Name(cluster=w3040, "xDistance"=w3038, "yDistance"=w3038, "wDistance"=w3038) -> (w3039:T6)
        n115 = Bundle By Name(cluster=w3042, "PING_A"=w3037, "PING_B"=w3037, "PING_C"=w3037, "PING_D"=w3037) -> (w3043:T7)
        n116 = Bundle By Name(cluster=w3026, "Yaw"=0.0) -> (w3025:T4)
      }
      frame "ARDUINO - ULTRASONIC" {
        # ">>> Time cluster >>>"
        # ">>> Line Sensor Cluster>>>"
        # ">>> Object detection >>>"
        # ">>> Yaw >>>"
        # ">>> Ultrasonic Sensors Detect >>>"
        # ">>> Encoders >>>"
        # ">>> Stepper position >>>"
        # ">>State Logic  >>"
        n117 = call "Arduino Interfacing VI.vi"("Data to Write"=I2C_MASTER_WRITE_NEW_Type_Def."Ultrasonic sensors", "AE Mode"=Arduino_Interfacing."Write to Arduino") -> ()  [unwired: 2 in, 2 out]
      }
      frame "NAVX CALIBRATE" {
        # ">>> Object detection >>>"
        # ">>> Yaw >>>"
        # ">>> Ultrasonic Sensors Detect >>>"
        # ">>> Encoders >>>"
        # ">>> Stepper position >>>"
        # ">>State Logic  >>"
        # "Adds a 15 second delay to the startup process \nfor the NavX to calibrate"
        n118 = Wait (ms)(milliseconds to wait=u32 1000) -> ()  [unwired: 1 out]
      }
      frame "NO ACTION", Default {
        (unwired) u8 0 ("y Stepper value")
        (unwired) TRUE ("Latch")
        (unwired) navX_type_def."Read Values" ("Mode")
        (unwired) MOTOR_CONTROL_NO_PID_Type_Def."Latch" ("Direction")
        # ">>> Object detection >>>"
        # ">>> Yaw >>>"
        # ">>> Ultrasonic Sensors Detect >>>"
        # ">>> Encoders >>>"
        # ">>> Stepper position >>>"
        # ">>State Logic  >>"
        n119 = case shown="4" w3076 {
          tunnel: [0 100] -> w3078
          frame 1, Default {
          }
          frame 4 {
          }
        }
      }
      frame "----RESET CASES----" {
        (unwired) I2C_MASTER_Type_Def."Last State" ("Arduino Mode")
        # ">>> Object detection >>>"
        # ">>> Yaw >>>"
        # ">>> Ultrasonic Sensors Detect >>>"
        # ">>> Encoders >>>"
        # ">>> Stepper position >>>"
        # ">>State Logic  >>"
      }
      frame "RESET ENCODERS" {
        # ">>> Object detection >>>"
        # ">>> Yaw >>>"
        # ">>> Ultrasonic Sensors Detect >>>"
        # ">>> Encoders >>>"
        # ">>> Stepper position >>>"
        # ">>State Logic  >>"
        n120 = call "MOTOR CONTROL WITH PID AE.vi"("Direction"=MOTOR_CONTROL_WITH_PID_AE_DIRECTION_TYPE_DEF."reset encoders", "AE Mode"=MOTOR_CONTROL_WITH_PID_AE_DATA_MODE_TYPE_DEF."Write to AE") -> ()  [unwired: 2 in, 1 out]
      }
      frame "RESET FLAGS" {
        # ">>> Line Sensor Cluster>>>"
        # ">>> IR Sensors >>>"
        # ">>> Time cluster >>>"
        # ">>> Object detection >>>"
        # ">>> Yaw >>>"
        # ">>> Ultrasonic Sensors Detect >>>"
        # ">>> Encoders >>>"
        # ">>> Stepper position >>>"
        # ">>> Line Sensor Cluster>>>"
        # ">>> IR Sensors >>>"
        # ">>> Time cluster >>>"
        # ">>> Object detection >>>"
        # ">>> Yaw >>>"
        # ">>> Ultrasonic Sensors Detect >>>"
        # ">>> Encoders >>>"
        # ">>> Stepper position >>>"
        # "Resets BOOLEAN FLAGS only"
        n121 = Wait (ms)(milliseconds to wait=u32 20) -> ()  [unwired: 1 out]
        n122 = Bundle By Name(cluster=w3117, "Recognized Object"=FALSE) -> (w3116:T9)
        n123 = Bundle By Name(cluster=w3107, "Line Detected?"=FALSE) -> (w3106:T1)
        n124 = Bundle By Name(cluster=w3111, "Time up flag"=FALSE) -> (w3110:T3)
      }
      frame "RESET SENSOR VALUES" {
        w3121 = 0.0 ("S4")
        w3122 = 0.0 ("S4")
        # "Resets SENSOR VALUES only"
        # ">>> Line Sensor Cluster>>>"
        # ">>> IR Sensors >>>"
        # ">>> Time cluster >>>"
        # ">>> Object detection >>>"
        # ">>> Yaw >>>"
        # ">>> Ultrasonic Sensors Detect >>>"
        # ">>> Encoders >>>"
        # ">>> Stepper position >>>"
        # ">>> Line Sensor Cluster>>>"
        # ">>> IR Sensors >>>"
        # ">>> Time cluster >>>"
        # ">>> Object detection >>>"
        # ">>> Yaw >>>"
        # ">>> Ultrasonic Sensors Detect >>>"
        # ">>> Encoders >>>"
        # ">>> Stepper position >>>"
        # "Resets any software variables\nand/or non-critical states"
        n125 = Wait (ms)(milliseconds to wait=u32 20) -> ()  [unwired: 1 out]
        n126 = Bundle By Name(cluster=w3130, "SET TIME TO CHECK"=0.0) -> (w3129:T3)
        n127 = Bundle By Name(cluster=w3146, "Object X coordinate"=0.0, "Object Y coordinate"=0.0) -> (w3145:T9)
        n128 = Bundle By Name(cluster=w3137, "y Stepper Position"=u8 0, "z Stepper Position"=u8 0) -> (w3136:T5)
        n129 = Bundle By Name(cluster=w3124, "Left IR Sensor"=w3121, "Arm IR Sensor"=w3121) -> (w3123:T2)
        n130 = Bundle By Name(cluster=w3142, "xDistance"=0.0, "yDistance"=0.0, "wDistance"=0.0) -> (w3141:T6)
        n131 = Bundle By Name(cluster=w3153, "PING_A"=u8 0, "PING_B"=u8 0, "PING_C"=u8 0, "PING_D"=u8 0) -> (w3152:T7)
        n132 = Bundle By Name(cluster=w3133, "Yaw"=0.0) -> (w3132:T4)
        n133 = Bundle By Name(cluster=w3126, "S1"=w3122, "S2"=w3122, "S3"=w3122, "S4"=w3122) -> (w3125:T1)
      }
      frame "RESET ALL SENSORS" {
        w3155 = 0.0 ("SET TIME TO CHECK")
        # ">>> Line Sensor Cluster>>>"
        # ">>> IR Sensors >>>"
        # ">>> Time cluster >>>"
        # ">>> Object detection >>>"
        # ">>> Yaw >>>"
        # ">>> Ultrasonic Sensors Detect >>>"
        # ">>> Encoders >>>"
        # ">>> Stepper position >>>"
        # ">>> Line Sensor Cluster>>>"
        # ">>> IR Sensors >>>"
        # ">>> Time cluster >>>"
        # ">>> Object detection >>>"
        # ">>> Yaw >>>"
        # ">>> Ultrasonic Sensors Detect >>>"
        # ">>> Encoders >>>"
        # ">>> Stepper position >>>"
        # "Resets ALL SENSOR PARAMTERS"
        n134 = Wait (ms)(milliseconds to wait=u32 20) -> ()  [unwired: 1 out]
        n135 = Bundle By Name(cluster=w3165, "Time up flag"=FALSE, "SET TIME TO CHECK"=0.0) -> (w3164:T3)
        n136 = Bundle By Name(cluster=w3182, "Recognized Object"=FALSE, "Object X coordinate"=0.0, "Object Y coordinate"=0.0) -> (w3181:T9)
        n137 = Bundle By Name(cluster=w3172, "y Stepper Position"=u8 0, "z Stepper Position"=u8 0) -> (w3171:T5)
        n138 = Bundle By Name(cluster=w3160, "Line Detected?"=FALSE) -> (w3159:T1)
        n139 = Bundle By Name(cluster=w3157, "Left IR Sensor"=w3155, "Arm IR Sensor"=w3155) -> (w3156:T2)
        n140 = Bundle By Name(cluster=w3177, "xDistance"=0.0, "yDistance"=0.0, "wDistance"=0.0) -> (w3176:T6)
        n141 = Bundle By Name(cluster=w3189, "PING_A"=u8 0, "PING_B"=u8 0, "PING_C"=u8 0, "PING_D"=u8 0) -> (w3188:T7)
        n142 = Bundle By Name(cluster=w3168, "Yaw"=0.0) -> (w3167:T4)
      }
      frame "RESET YAW" {
        n143 = Wait (ms)(milliseconds to wait=u32 100) -> ()  [unwired: 1 out]
        n144 = call "navX reading VI.vi"("Mode"=navX_type_def."Zero Yaw") -> ()  [unwired: 2 in, 4 out]
      }
      frame "RESET ARM" {
        n145 = call "Arduino Interfacing VI.vi"("Data to Write"=I2C_MASTER_WRITE_NEW_Type_Def."Soft Reset", "AE Mode"=Arduino_Interfacing."Write to Arduino") -> ()  [unwired: 2 in, 2 out]
      }
      frame "--------CAM STATES-------" {
      }
      frame "OPEN IMAQ REF" {
        # ">>> Line Sensor Cluster>>>"
        # ">>State Logic  >>"
        # ">>> Time cluster >>>"
        # ">>> Object detection >>>"
        # ">>> Yaw >>>"
        # ">>> Ultrasonic Sensors Detect >>>"
        # ">>> Encoders >>>"
        # ">>> Stepper position >>>"
        # ">>> IR Sensors >>>"
        n146 = call "IMAQ Reference AE.vi"("IMAQ AE States"=IMAQ_Reference_AE."Initialize AE") -> ()  [unwired: 1 in, 2 out]
      }
      frame "OPEN LOG CAM" {
        n147 = call "Webcam AE.vi"("Session In"=T37 "cam0", "Camera states"=Webcam_AE."Initialize Camera") -> ("error out"=w3241:errorcluster, "Session Out"=w3240:T37)  [unwired: 1 in, 1 out]
        n148 = call "Webcam AE.vi"("error in (no error)"=w3241, "Session In"=w3240, "Camera states"=Webcam_AE."Open Camera") -> ()  [unwired: 3 out]
      }
      frame "OPEN LIFE CAM" {
        n149 = call "Webcam AE.vi"("Session In"=T37 "cam1", "Camera states"=Webcam_AE."Initialize Camera") -> ("error out"=w3256:errorcluster, "Session Out"=w3255:T37)  [unwired: 1 in, 1 out]
        n150 = call "Webcam AE.vi"("error in (no error)"=w3256, "Session In"=w3255, "Camera states"=Webcam_AE."Open Camera") -> ()  [unwired: 3 out]
      }
      frame "CAM ACQ" {
        # ">>State Logic  >>"
        # ">>> Time cluster >>>"
        # ">>> Yaw >>>"
        # ">>> Stepper position >>>"
        # ">>> Encoders >>>"
        # ">>> Object detection >>>"
        # ">>> Ultrasonic Sensors Detect >>>"
        n151 = call "Webcam AE.vi"("Camera states"=Webcam_AE."Continuous Acquisition") -> ()  [unwired: 2 in, 3 out]
      }
      frame "CAM CLOSE" {
        # ">>State Logic  >>"
        # ">>> Time cluster >>>"
        # ">>> Yaw >>>"
        # ">>> Stepper position >>>"
        # ">>> Encoders >>>"
        # ">>> Object detection >>>"
        # ">>> Ultrasonic Sensors Detect >>>"
        n152 = call "Webcam AE.vi"("Camera states"=Webcam_AE."Close Camera") -> ()  [unwired: 2 in, 3 out]
      }
      frame "PROCESS IMAGE" {
        # ">>> Line Sensor Cluster>>>"
        # ">>> IR Sensors >>>"
        # ">> Item Selection Bias >>"
        # ">> Item Selection Bias >>"
        # ">>State Logic  >>"
        # ">>> Time cluster >>>"
        # ">>> Yaw >>>"
        # ">>> Stepper position >>>"
        # ">>> Encoders >>>"
        # ">>> Object detection >>>"
        # ">>> Ultrasonic Sensors Detect >>>"
        n153 = call "Webcam AE.vi"("Camera states"=Webcam_AE."Retrieve Image") -> ("error out"=w3301:errorcluster, "Image Out"=w3302:T43)  [unwired: 2 in, 1 out]
        n154 = call "IMAQ Reference AE.vi"("IMAQ AE States"=IMAQ_Reference_AE."Get IMAQ Reference") -> ("Image Out"=w3291:T43)  [unwired: 1 in, 1 out]
        n155 = call "Object Detection SubVI.vi"("Error In"=w3301, "Mode"=w3288, "Image Dest"=w3291, "Image in"=w3302) -> ("Error out"=w3289:errorcluster, "Object Center Coordinates"=w3298:cluster{"x":sgl, "y":sgl}, "Object detection cluster"=w3294:T44)  [unwired: 1 out]
        n156 = Unbundle By Name(w3294) -> ("Object detected?"=w3295:bool)
        n157 = Unbundle By Name(w3298) -> ("x"=w3297:sgl, "y"=w3296:sgl)
        n158 = Bundle By Name(cluster=w3300, "Recognized Object"=w3295, "Object X coordinate"=w3297, "Object Y coordinate"=w3296) -> (w3299:T9)
      }
      frame "DISPOSE CAM BUFFERS" {
        # ">> Item Selection Bias >>"
        # ">>> Line Sensor Cluster>>>"
        # ">>> IR Sensors >>>"
        # ">>State Logic  >>"
        # ">>> Time cluster >>>"
        # ">>> Yaw >>>"
        # ">>> Stepper position >>>"
        # ">>> Encoders >>>"
        # ">>> Object detection >>>"
        # ">>> Ultrasonic Sensors Detect >>>"
        n159 = call "Webcam AE.vi"("Camera states"=Webcam_AE."Dispose Camera Image Buffer") -> ()  [unwired: 2 in, 3 out]
      }
      frame "DISPOSE PROC BUFFERS" {
        # ">>> Line Sensor Cluster>>>"
        # ">>State Logic  >>"
        # ">>> IR Sensors >>>"
        # ">>> Time cluster >>>"
        # ">>> Object detection >>>"
        # ">>> Yaw >>>"
        # ">>> Ultrasonic Sensors Detect >>>"
        # ">>> Encoders >>>"
        # ">>> Stepper position >>>"
        n160 = call "IMAQ Reference AE.vi"("IMAQ AE States"=IMAQ_Reference_AE."Dispose Processing Buffer") -> ()  [unwired: 1 in, 2 out]
      }
      frame "-----ARM ACTIONS-----" {
      }
      frame "CLOSE CLAW" {
        n161 = call "Arduino Interfacing VI.vi"("Data to Write"=I2C_MASTER_WRITE_NEW_Type_Def."Close Claw", "AE Mode"=Arduino_Interfacing."Write to Arduino") -> ()  [unwired: 2 in, 2 out]
      }
      frame "OPEN CLAW" {
        n162 = call "Arduino Interfacing VI.vi"("Data to Write"=I2C_MASTER_WRITE_NEW_Type_Def."Open Claw", "AE Mode"=Arduino_Interfacing."Write to Arduino") -> ()  [unwired: 2 in, 2 out]
      }
      frame "Z STEPPER CAM HEIGHT" {
        n163 = call "Arduino Interfacing VI.vi"("Data to Write"=I2C_MASTER_WRITE_NEW_Type_Def."zStepper 6k", "AE Mode"=Arduino_Interfacing."Write to Arduino") -> ()  [unwired: 2 in, 2 out]
      }
      frame "Z STEPPER GRAB HEIGHT" {
        # ">>State Logic  >>"
        # ">>> Time cluster >>>"
        # ">>> Yaw >>>"
        # ">>> Stepper position >>>"
        # ">>> Encoders >>>"
        # ">>> Object detection >>>"
        # ">>> Ultrasonic Sensors Detect >>>"
        n164 = call "Arduino Interfacing VI.vi"("Data to Write"=I2C_MASTER_WRITE_NEW_Type_Def."zStepper 100", "AE Mode"=Arduino_Interfacing."Write to Arduino") -> ()  [unwired: 2 in, 2 out]
      }
      frame "Z STEPPER BOX HEIGHT" {
        # ">>> IR Sensors >>>"
        # ">>> Time cluster >>>"
        # ">>> Yaw >>>"
        # ">>> Stepper position >>>"
        # ">>> Encoders >>>"
        # ">>> Object detection >>>"
        # ">>> Ultrasonic Sensors Detect >>>"
        n165 = call "Arduino Interfacing VI.vi"("Data to Write"=I2C_MASTER_WRITE_NEW_Type_Def."zStepper 4k", "AE Mode"=Arduino_Interfacing."Write to Arduino") -> ()  [unwired: 2 in, 2 out]
      }
      frame "Y STEPPER CONTROL" {
        # ">>State Logic  >>"
        # ">>> yStepper command>>>"
        # ">>> Time cluster >>>"
        # ">>> Yaw >>>"
        # ">>> Stepper position >>>"
        # ">>> Encoders >>>"
        # ">>> Object detection >>>"
        # ">>> Ultrasonic Sensors Detect >>>"
        n166 = Unbundle By Name(w3406) -> ("yStepper desired"=w3405:u8)
        n167 = call "Arduino Interfacing VI.vi"("y Stepper value"=w3405, "Data to Write"=I2C_MASTER_WRITE_NEW_Type_Def."yStepper control", "AE Mode"=Arduino_Interfacing."Write to Arduino") -> ()  [unwired: 1 in, 2 out]
      }
      frame "READ STEPPER VALUES" {
        # ">>State Logic  >>"
        # ">>> Time cluster >>>"
        # ">>> Yaw >>>"
        # ">>> Stepper position >>>"
        # ">>> Encoders >>>"
        # ">>> Object detection >>>"
        # ">>> Ultrasonic Sensors Detect >>>"
        n168 = call "Arduino Interfacing VI.vi"("AE Mode"=Arduino_Interfacing."Read From Arduino") -> ("Arduino Data"=w3423:T15)  [unwired: 3 in, 1 out]
        n169 = Unbundle By Name(w3423) -> ("y Stepper Position"=w3422:u8, "z Stepper Position"=w3421:u8)
        n170 = Bundle By Name(cluster=w3426, "y Stepper Position"=w3422, "z Stepper Position"=w3421) -> (w3425:T5)
      }
      frame " -----TIMING-----" {
        # ">>State Logic  >>"
        # ">>> Time cluster >>>"
        # ">>> Yaw >>>"
        # ">>> Stepper position >>>"
        # ">>> Encoders >>>"
        # ">>> Object detection >>>"
        # ">>> Ultrasonic Sensors Detect >>>"
      }
      frame "SET TIMER 1" {
        # ">>State Logic  >>"
        # ">>> Time cluster >>>"
        # ">>> Yaw >>>"
        # ">>> Stepper position >>>"
        # ">>> Encoders >>>"
        # ">>> Object detection >>>"
        # ">>> Ultrasonic Sensors Detect >>>"
        n171 = call "Elasped Timer.vi"("Time Setting"=1.0, "Action"=Elapsed_timer_control."Initialize") -> ()  [unwired: 6 in, 4 out]
        n172 = Bundle By Name(cluster=w3448, "Time up flag"=FALSE) -> (w3446:T3)
      }
      frame "SET TIMER 2" {
        # ">>State Logic  >>"
        # ">>> Time cluster >>>"
        # ">>> Yaw >>>"
        # ">>> Stepper position >>>"
        # ">>> Encoders >>>"
        # ">>> Object detection >>>"
        # ">>> Ultrasonic Sensors Detect >>>"
        n173 = call "Elasped Timer.vi"("Time Setting"=2.0, "Action"=Elapsed_timer_control."Initialize") -> ()  [unwired: 6 in, 4 out]
        n174 = Bundle By Name(cluster=w3462, "Time up flag"=FALSE) -> (w3460:T3)
      }
      frame "SET TIMER 3" {
        # ">>State Logic  >>"
        # ">>> Time cluster >>>"
        # ">>> Yaw >>>"
        # ">>> Stepper position >>>"
        # ">>> Encoders >>>"
        # ">>> Object detection >>>"
        # ">>> Ultrasonic Sensors Detect >>>"
        n175 = call "Elasped Timer.vi"("Time Setting"=3.0, "Action"=Elapsed_timer_control."Initialize") -> ()  [unwired: 6 in, 4 out]
        n176 = Bundle By Name(cluster=w3476, "Time up flag"=FALSE) -> (w3474:T3)
      }
      frame "SET TIMER 4" {
        # ">>State Logic  >>"
        # ">>> Time cluster >>>"
        # ">>> Yaw >>>"
        # ">>> Stepper position >>>"
        # ">>> Encoders >>>"
        # ">>> Object detection >>>"
        # ">>> Ultrasonic Sensors Detect >>>"
        n177 = call "Elasped Timer.vi"("Time Setting"=4.0, "Action"=Elapsed_timer_control."Initialize") -> ()  [unwired: 6 in, 4 out]
        n178 = Bundle By Name(cluster=w3490, "Time up flag"=FALSE) -> (w3488:T3)
      }
      frame "SET TIMER 5" {
        # ">>State Logic  >>"
        # ">>> Time cluster >>>"
        # ">>> Yaw >>>"
        # ">>> Stepper position >>>"
        # ">>> Encoders >>>"
        # ">>> Object detection >>>"
        # ">>> Ultrasonic Sensors Detect >>>"
        n179 = call "Elasped Timer.vi"("Time Setting"=5.0, "Action"=Elapsed_timer_control."Initialize") -> ()  [unwired: 6 in, 4 out]
        n180 = Bundle By Name(cluster=w3504, "Time up flag"=FALSE) -> (w3502:T3)
      }
      frame "START TIMER" {
        # ">>State Logic  >>"
        # ">>> Time cluster >>>"
        # ">>> Yaw >>>"
        # ">>> Stepper position >>>"
        # ">>> Encoders >>>"
        # ">>> Object detection >>>"
        # ">>> Ultrasonic Sensors Detect >>>"
        n181 = call "Elasped Timer.vi"("Action"=Elapsed_timer_control."Start") -> ("Time Out?!"=w3514:bool)  [unwired: 7 in, 3 out]
        n182 = Bundle By Name(cluster=w3517, "Time up flag"=w3514) -> (w3516:T3)
      }
    }
    "State Logic" <- w246
    "Image Processing Error" <- w213
    n183 = local read "TASK ENABLE"() -> (w240:bool)
    n184 = Not(x=w240) -> (.not. x?=w239:bool)
    n185 = case shown="True" w247 {
      tunnel: w251 -> [w278 w318]
      tunnel: w255 -> [w274 w320]
      tunnel: [w278 w318] -> w260
      tunnel: [w274 w321] -> w259
      tunnel: w256 -> [_ w316]
      tunnel: w258 -> [_ w317]
      tunnel: w253 -> [w277 w323]
      tunnel: [w277 w323] -> w252
      tunnel: "STOP TASK" -> [_ w306]
      tunnel: w246 -> [w276 w322]
      tunnel: [w276 w319] -> w245
      tunnel: w242 -> [w275 w312]
      tunnel: [w275 w312] -> w241
      tunnel: w239 -> [_ w307]
      tunnel: [w273 w304] -> w238
      tunnel: w237 -> [w273 w303]
      tunnel: w235 -> [w272 w300]
      tunnel: [w272 w300] -> w234
      tunnel: w232 -> [w271 w296]
      tunnel: [w271 w296] -> w231
      tunnel: w229 -> [w270 w294]
      tunnel: [w270 w294] -> w228
      tunnel: w226 -> [w269 w292]
      tunnel: [w269 w292] -> w225
      tunnel: w224 -> [w268 w291]
      tunnel: [w268 w290] -> w223
      tunnel: [_ w288] -> w222
      tunnel: w220 -> [w267 w286]
      tunnel: [w267 w286] -> w219
      tunnel: w218 -> [w266 w285]
      tunnel: [w266 w284] -> w217
      tunnel: w215 -> [w265 w281]
      tunnel: [w265 w281] -> w214
      tunnel: [w264 w280] -> w212
      tunnel: w210 -> [w264 w279]
      frame False {
        # ">> Item Selection Bias >>"
        # ">>State Logic Queue Reference >>"
        # ">>Action states Queue Reference >>"
        # ">>True Stop Next State >>"
        # ">>State Logic  >>"
        # ">>> IR Sensors >>>"
        # ">>> Line Sensor Cluster>>>"
        # ">>> Line Sensor Cluster>>>"
        # ">>> Motor control cluster >>>"
        # ">>> yStepper command>>>"
        # ">>> Motor control cluster >>>"
        # ">>> yStepper command>>>"
        # ">>> Motor control cluster >>>"
        # ">>> IR Sensors >>>"
        # ">>> IR Sensors >>>"
        # ">>> yStepper command>>>"
        # ">>> Time cluster >>>"
        # ">>> Yaw >>>"
        # ">>> Stepper position >>>"
        # ">>> Encoders >>>"
        # ">>> Object detection >>>"
        # ">>> Ultrasonic Sensors Detect >>>"
        # ">>> Time cluster >>>"
        # ">>> Yaw >>>"
        # ">>> Stepper position >>>"
        # ">>> Encoders >>>"
        # ">>> Object detection >>>"
        # ">>> Ultrasonic Sensors Detect >>>"
      }
      frame True {
        # ">> Item Selection Bias >>"
        # ">>> IR Sensors >>>"
        # ">>> Line Sensor Cluster>>>"
        # ">>> Line Sensor Cluster>>>"
        # ">>> Motor control cluster >>>"
        # ">>> yStepper command>>>"
        # ">>> IR Sensors >>>"
        # ">>> Motor control cluster >>>"
        # ">>State Logic Queue Reference >>"
        # ">>Timeout>>"
        # ">>> yStepper command>>>"
        # ">>> Time cluster >>>"
        # ">>> Object detection >>>"
        # ">>> Yaw >>>"
        # ">>> Ultrasonic Sensors Detect >>>"
        # ">>> Encoders >>>"
        # ">>> Stepper position >>>"
        # ">>State Logic  >>"
        # ">>True Stop Next State >>"
        # ">>Action Queue>>"
        # ">> Manual override >>"
        # ">>> Time cluster >>>"
        # ">>> Yaw >>>"
        # ">>> Stepper position >>>"
        # ">>> Encoders >>>"
        # ">>> Object detection >>>"
        # ">>> Ultrasonic Sensors Detect >>>"
        # ">>Action Queue>>"
        # ">>State Logic Queue Reference >>"
        n186 = Or(x=w306, y=w307) -> (x .or. y?=w305:bool)
        n187 = Unbundle By Name(w281) -> ("Line Detected?"=w282:bool)
        n188 = Unbundle By Name(w286) -> ("Left IR Sensor"=w287:dbl, "Arm IR Sensor"=w283:dbl)
        n189 = Unbundle By Name(w292) -> ("Time up flag"=w293:bool)
        n190 = Unbundle By Name(w294) -> ("Yaw"=w295:dbl, "Compass"=w289:dbl)
        n191 = Unbundle By Name(w296) -> ("y Stepper Position"=w298:u8, "z Stepper Position"=w297:u8)
        n192 = Unbundle By Name(w312) -> ("xDistance"=w309:dbl, "yDistance"=w310:dbl, "wDistance"=w311:dbl)
        n193 = Unbundle By Name(w300) -> ("Recognized Object"=w299:bool, "Object X coordinate"=w302:dbl, "Object Y coordinate"=w301:dbl)
        n194 = Unbundle By Name(w323) -> ("PING_A"=w315:u8, "PING_B"=w314:u8, "PING_C"=w313:u8, "PING_D"=w308:u8)
        n195 = case shown="16" w322 {
          tunnel: [w328 w340 w354 w365 w483 w500 w546 w583 w637 w680 w728 w772 w827 w875 w919 w979 w1025 w1066 w1115 w1158 w1211 w1249 w1301 w1345 w1389 w1419 w1437 w1483 w1524 w1573 w1626 w1665 w1714 w1757 w1810 w1848 w1900 w1936 w1985 w2028 w2081 w2125 w2170 w2222 w2263 w2311 w2350 w2392 w2447 w2501 w2539 w2585 w2634 w2675 w2719] -> w321
          tunnel: w320 -> [w328 w343 w355 w368 w485 w501 w547 w592 w635 w684 w729 w778 w820 w878 w926 w969 w1028 w1072 w1114 w1161 w1201 w1255 w1291 w1340 w1380 w1419 w1427 w1486 w1530 w1572 w1625 w1671 w1713 w1760 w1800 w1854 w1890 w1940 w1992 w2033 w2086 w2130 w2174 w2220 w2264 w2312 w2352 w2402 w2457 w2500 w2543 w2591 w2633 w2679 w2723]
          tunnel: [State_Type_Definitions,_for_0.26g_versions_and_later_2."Idle" ("Enum") State_Type_Definitions,_for_0.26g_versions_and_later_2."Idle" ("Enum") w350 w367 State_Type_Definitions,_for_0.26g_versions_and_later_2."Shutdown" ("Enum") w502 w548 w590 w638 w681 w727 w773 w826 w876 w921 w978 w1026 w1073 w1116 w1160 w1210 w1256 w1300 w1346 w1381 State_Type_Definitions,_for_0.26g_versions_and_later_2."Idle" ("Enum") w1436 w1484 w1531 w1574 w1627 w1672 w1715 w1759 w1809 w1855 w1899 w1937 w1986 w2029 w2082 w2126 w2171 w2223 w2262 w2310 w2351 w2397 w2458 w2502 w2540 w2586 w2635 w2676 w2720] -> w319
          tunnel: w318 -> [_ _ w353 w371 _ w506 w553 w586 w634 w685 w736 w777 w824 w879 w925 w976 w1023 w1071 w1112 w1162 w1208 w1254 w1298 w1343 w1388 _ w1434 w1481 w1529 w1570 w1623 w1670 w1711 w1761 w1807 w1853 w1897 w1944 w1991 w2036 w2089 w2133 w2177 w2219 w2265 w2305 w2353 w2401 w2456 w2499 w2547 w2590 w2632 w2683 w2724]
          tunnel: w317 -> [_ _ _ w370 _ w505 w552 w585 w633 w686 w735 w776 w823 w872 w924 w975 w1022 w1070 w1111 w1163 w1207 w1253 w1297 w1342 w1386 _ w1433 w1480 w1528 w1569 w1622 w1669 w1710 w1762 w1806 w1852 w1896 w1939 w1990 w2035 w2088 w2132 w2173 w2218 w2266 w2306 w2354 w2400 w2455 w2498 w2546 w2589 w2631 w2682 w2725]
          tunnel: w316 -> [_ _ w352 w366 _ w504 w551 w584 w632 w687 w734 w775 w822 w871 w923 w977 w1024 w1069 w1110 w1164 w1209 w1252 w1299 w1341 w1387 _ w1435 w1482 w1527 w1568 w1621 w1668 w1709 w1763 w1808 w1851 w1898 w1943 w1989 w2034 w2087 w2131 w2176 w2217 w2267 w2307 w2355 w2399 w2454 w2497 w2545 w2588 w2630 w2681 w2726]
          tunnel: w305 -> [_ _ _ _ _ w491 w545 w591 w631 w688 w731 w771 w825 w877 w927 w970 w1029 w1067 w1113 w1165 w1202 w1250 w1292 w1344 w1384 _ w1428 w1487 w1525 w1571 w1624 w1666 w1712 w1764 w1801 w1849 w1891 w1942 w1984 w2032 w2085 w2129 w2175 w2216 w2268 w2308 w2356 w2398 w2453 w2496 w2544 w2587 w2629 w2680 w2727]
          tunnel: w315 -> [_ _ _ _ _ _ _ _ _ _ _ _ _ _ _ _ _ _ _ _ _ _ _ _ _ _ _ _ _ _ _ _ _ _ _ _ _ _ _ _ _ _ _ _ _ _ _ _ _ _ _ _ _ _ _]
          tunnel: w314 -> [_ _ _ _ _ _ _ _ w630 _ _ _ w816 w860 w917 _ w1015 _ _ _ _ _ _ _ _ _ _ w1473 _ _ _ _ _ _ _ _ _ _ _ _ w2076 _ _ _ _ _ _ _ w2451 _ _ _ _ _ _]
          tunnel: w313 -> [_ _ _ _ _ _ _ _ w629 _ _ _ w817 w861 w918 _ w1016 _ _ _ _ _ _ _ _ _ _ w1474 _ _ _ _ _ _ _ _ _ _ _ _ w2075 _ _ _ _ _ _ _ w2452 _ _ _ _ _ _]
          tunnel: w311 -> [_ _ _ _ _ _ _ _ _ _ w733 _ _ _ _ _ _ _ _ _ _ _ _ _ _ _ _ _ _ _ _ _ _ _ _ _ _ _ _ _ _ _ _ _ _ _ _ w2395 _ _ _ _ _ _ _]
          tunnel: w310 -> [_ _ _ _ _ w499 w544 _ _ w679 _ _ _ _ w922 _ _ _ _ _ _ _ _ _ _ _ _ _ _ _ _ _ _ _ _ _ _ _ _ _ _ _ _ _ _ _ _ _ w2443 _ _ _ _ _ _]
          tunnel: w309 -> [_ _ _ _ _ _ _ _ _ _ _ _ _ w866 _ _ _ _ _ _ _ _ _ _ _ _ _ _ _ _ w1612 _ _ _ _ _ _ _ _ _ _ _ _ _ w2257 _ _ _ _ _ _ _ w2628 _ _]
          tunnel: w308 -> [_ _ _ _ _ _ _ _ _ _ _ _ _ _ _ _ _ _ _ _ _ _ _ _ _ _ _ _ _ _ _ _ _ _ _ _ _ _ _ _ _ _ _ _ _ _ _ _ _ _ _ _ _ _ _]
          tunnel: [State_Type_Definitions,_for_0.26g_versions_and_later_2."Idle" ("Enum") State_Type_Definitions,_for_0.26g_versions_and_later_2."Idle" ("Enum") State_Type_Definitions,_for_0.26g_versions_and_later_2."Idle" ("Enum") State_Type_Definitions,_for_0.26g_versions_and_later_2."Idle" ("Enum") State_Type_Definitions,_for_0.26g_versions_and_later_2."Shutdown" ("Enum") w497 w542 w589 w636 w682 w724 w770 w819 w874 w920 w980 w1027 w1065 w1117 w1159 w1212 w1248 w1302 w1347 w1382 w1421 w1438 w1485 w1523 w1575 w1628 w1664 w1716 w1758 w1811 w1847 w1901 w1938 w1987 w2031 w2084 w2128 w2172 w2221 w2261 w2309 w2349 w2396 w2459 w2503 w2541 w2584 w2636 w2677 w2721] -> w304
          tunnel: w303 -> [_ _ w350 _ _ _ _ _ _ _ _ _ _ _ _ _ _ _ _ _ _ _ _ _ _ w1421 _ _ _ _ _ _ _ _ _ _ _ _ _ _ _ _ _ _ _ _ _ _ _ _ _ _ _ _ _]
          tunnel: w299 -> [_ _ _ _ _ _ _ _ _ _ _ _ _ _ _ _ _ _ _ _ _ _ _ _ w1383 _ _ _ _ _ _ _ _ _ _ _ _ _ _ _ _ _ _ _ _ _ _ _ _ _ _ _ _ _ _]
          tunnel: w302 -> [_ _ _ _ _ _ _ _ _ _ _ _ _ _ _ _ _ _ _ _ _ _ _ _ _ _ _ _ _ _ w1618 _ _ _ _ _ _ _ _ _ _ _ _ _ _ _ _ _ _ _ _ _ _ _ _]
          tunnel: w301 -> [_ _ _ _ _ _ _ _ _ _ _ _ _ _ _ _ _ _ _ w1154 _ _ _ _ _ _ _ _ _ _ _ _ _ w1753 _ _ _ _ _ _ _ _ _ _ _ _ _ _ _ _ _ _ _ _ _]
          tunnel: w298 -> [_ _ _ _ _ _ _ _ _ _ _ _ _ _ _ _ _ _ _ w1153 _ _ _ _ _ _ _ _ _ _ _ _ _ w1752 _ _ _ _ _ _ _ _ _ _ _ _ _ _ _ _ _ _ _ _ _]
          tunnel: w297 -> [_ _ _ _ _ _ _ w588 _ _ _ w768 _ _ _ w973 _ _ _ _ w1205 _ w1295 w1339 _ _ w1431 _ _ _ _ _ _ _ w1804 _ w1894 w1941 _ _ _ _ _ _ _ _ _ _ _ _ _ _ _ _ _]
          tunnel: w295 -> [_ _ _ _ _ _ _ _ _ _ _ _ _ _ _ _ _ _ _ _ _ _ _ _ _ _ _ _ _ _ _ _ _ _ _ _ _ _ _ _ _ _ _ _ _ _ _ _ _ _ _ _ _ _ _]
          tunnel: w293 -> [_ _ _ _ _ _ _ _ _ _ _ _ _ _ _ _ _ w1063 w1107 _ _ w1246 _ _ _ _ _ _ w1521 w1565 _ w1662 w1706 _ _ w1845 _ _ _ _ _ _ w2166 _ _ w2304 w2348 _ _ _ w2542 w2583 _ w2678 w2722]
          tunnel: w291 -> [w326 w338 w349 w363 w481 w496 w541 w587 w628 w683 w723 w769 w818 w870 w916 w968 w1020 w1064 w1108 w1156 w1200 w1247 w1290 w1336 w1379 w1422 w1426 w1478 w1522 w1566 w1619 w1663 w1707 w1755 w1799 w1846 w1889 w1935 w1988 w2030 w2083 w2127 w2169 w2215 w2270 w2314 w2358 w2404 w2461 w2505 w2549 w2593 w2641 w2685 w2729]
          tunnel: [w326 w337 w349 w363 w481 w496 w541 w587 w628 w683 w723 w769 w818 w870 w916 w968 w1020 w1064 w1108 w1155 w1200 w1247 w1290 w1336 w1379 w1422 w1426 w1478 w1522 w1566 w1619 w1663 w1707 w1754 w1799 w1846 w1889 w1935 w1988 w2030 w2083 w2127 w2169 w2215 w2270 w2314 w2358 w2404 w2461 w2505 w2549 w2593 w2641 w2685 w2729] -> w290
          tunnel: w289 -> [_ _ _ _ _ _ _ _ _ _ _ _ _ _ _ _ _ _ _ _ _ _ _ _ _ _ _ _ _ _ _ _ _ _ _ _ _ _ w1983 _ _ _ _ _ _ _ _ _ _ _ _ _ _ _ _]
          tunnel: [_ _ _ TRUE _ _ _ _ _ _ _ _ _ _ _ _ _ _ _ _ _ _ _ _ _ _ _ _ _ _ _ _ _ _ _ _ _ _ _ _ _ _ _ _ _ _ _ _ _ _ _ _ _ _ _] -> w288
          tunnel: w287 -> [_ _ _ _ _ _ _ _ _ _ _ _ _ _ _ _ _ _ _ _ _ _ _ _ _ _ _ _ _ _ _ _ _ _ _ _ _ _ _ _ _ _ _ _ _ _ _ _ _ _ _ _ _ _ _]
          tunnel: w285 -> [w325 w335 w348 w361 w480 w495 w540 w582 w627 w676 w722 w765 w811 w859 w915 w967 w1013 w1062 w1106 w1150 w1199 w1245 w1289 w1335 w1378 w1423 w1425 w1471 w1520 w1564 w1615 w1661 w1705 w1749 w1798 w1844 w1888 w1934 w1979 w2027 w2080 w2124 w2168 w2214 w2272 w2316 w2360 w2406 w2463 w2507 w2551 w2595 w2643 w2687 w2731]
          tunnel: [w325 w334 w348 w361 w480 w495 w540 w582 w627 w676 w722 w765 w811 w859 w915 w967 w1013 w1062 w1106 w1150 w1199 w1245 w1289 w1335 w1378 w1423 w1425 w1471 w1520 w1564 w1614 w1661 w1705 w1749 w1798 w1844 w1888 w1934 w1979 w2027 w2080 w2124 w2168 w2214 w2272 w2316 w2360 w2406 w2463 w2507 w2551 w2595 w2643 w2687 w2731] -> w284
          tunnel: w283 -> [_ _ _ _ _ _ _ _ _ _ _ _ _ _ _ _ _ _ _ _ _ _ _ _ _ _ _ _ _ _ _ _ _ _ _ _ _ _ _ _ w2078 _ _ w2213 _ _ _ _ w2449 _ _ _ _ _ _]
          tunnel: w282 -> [_ _ _ _ _ w492 _ _ _ _ _ _ _ _ w913 _ _ _ _ _ _ _ _ _ _ _ _ _ _ _ _ _ _ _ _ _ _ _ _ w2026 _ w2122 _ _ w2259 _ _ _ _ w2495 _ _ w2627 _ _]
          tunnel: [w324 w330 w347 w360 w479 w494 w539 w581 w626 w675 w721 w764 w810 w858 w914 w966 w1012 w1061 w1105 w1149 w1198 w1244 w1288 w1334 w1377 w1418 w1424 w1470 w1519 w1563 w1607 w1660 w1704 w1748 w1797 w1843 w1887 w1933 w1978 w2025 w2077 w2123 w2167 w2210 w2271 w2315 w2359 w2405 w2462 w2506 w2550 w2594 w2642 w2686 w2730] -> w280
          tunnel: w279 -> [w324 w330 w347 _ w479 w494 w539 w581 w626 w675 w721 w764 w810 w858 w914 w966 w1012 w1061 w1105 w1149 w1198 w1244 w1288 w1334 w1377 w1418 w1424 w1470 w1519 w1563 w1607 w1660 w1704 w1748 w1797 w1843 w1887 w1933 w1978 w2025 w2077 w2123 w2167 w2210 w2271 w2315 w2359 w2405 w2462 w2506 w2550 w2594 w2642 w2686 w2730]
          frame 0 {
            # ">>> yStepper command>>>"
          }
          frame 1 {
            # ">>> yStepper command>>>"
            n196 = for {
              shift-right: [w346] -> w340
              shift-left: w343 -> [w345]
              tunnel: string[] ["INIT", "RESET ARM", "RESET FLAGS", "RESET YAW", "NAVX CALIBRATE"] -> [w344] mode=indexing
              n197 = Enqueue Element(queue=w345, element=w344) -> (queue out=w346:refnum<queue>)  [unwired: 2 in, 2 out]
            }
            n198 = Bundle By Name(cluster=w338, "yStepper desired"=u8 0) -> (w337:T18)
            n199 = Bundle By Name(cluster=w335, "ySpeed"=0.0, "xSpeed"=0.0, "wSpeed"=0.0) -> (w334:T17)
          }
          frame 3 {
            # ">>Action Queue>>"
            # ">>> Motor control cluster >>>"
            # ">>> yStepper command>>>"
            n200 = Flush Queue(queue=w353, error in (no error)=w352) -> ()  [unwired: 3 out]
            n201 = for {
              shift-right: [w359] -> w354
              shift-left: w355 -> [w358]
              tunnel: string[] ["STOP", "RESET ENCODERS", "RESET YAW", "RESET ARM", "RESET ALL SENSORS", "DISPOSE CAM BUFFERS", "DISPOSE PROC BUFFERS", "CAM CLOSE", ""] -> [w357] mode=indexing
              n202 = Enqueue Element(queue=w358, element=w357) -> (queue out=w359:refnum<queue>)  [unwired: 2 in, 2 out]
            }
          }
          frame 4, Default {
            # ">>> Motor control cluster >>>"
            # ">>> yStepper command>>>"
            n203 = Dequeue Element(queue=w371, timeout in ms (-1)=w370, error in (no error)=w366) -> (element=w369:T8)  [unwired: 3 out]
            n204 = case shown="\"Start Task 1\"" w369 {
              tunnel: [w374 w382 w390 w398 w406 w414 w422 w430 w438 w445 w455 w463 w470 w473] -> w365
              tunnel: w368 -> [w375 w383 w391 w399 w407 w415 w423 w431 w439 w446 w454 w462 w470 w474]
              tunnel: [State_Type_Definitions,_for_0.26g_versions_and_later_2."Task 1A" ("Enum") State_Type_Definitions,_for_0.26g_versions_and_later_2."Task 2:Raise Arm" ("Enum") State_Type_Definitions,_for_0.26g_versions_and_later_2."Task 3" ("Enum") State_Type_Definitions,_for_0.26g_versions_and_later_2."Task 4_A" ("Enum") State_Type_Definitions."Task 5A: ARM CAM HEIGHT" ("Enum") State_Type_Definitions,_for_0.26g_versions_and_later_2."Task 6_A" ("Enum") State_Type_Definitions,_for_0.26g_versions_and_later_2."Task 8A: RAISE ARM" ("Enum") State_Type_Definitions,_for_0.26g_versions_and_later_2."Task 8A: RAISE ARM" ("Enum") State_Type_Definitions,_for_0.26g_versions_and_later_2."Task 8A: RAISE ARM" ("Enum") State_Type_Definitions,_for_0.26g_versions_and_later_2."Task 8A: RAISE ARM" ("Enum") State_Type_Definitions,_for_0.26g_versions_and_later_2."Task 9A: Raise Arm" ("Enum") State_Type_Definitions."Task 9F: SCAN IMAGE" ("Enum") State_Type_Definitions,_for_0.26g_versions_and_later_2."Idle" ("Enum") State_Type_Definitions,_for_0.26g_versions_and_later_2."Shutdown" ("Enum")] -> w367
              tunnel: [enum16{"Ball", "Soap", "Gel", "Pipe", "None"}."None" ("Object recognition mode") enum16{"Ball", "Soap", "Gel", "Pipe", "None"}."None" ("Object recognition mode") enum16{"Ball", "Soap", "Gel", "Pipe", "None"}."None" ("Object recognition mode") enum16{"Ball", "Soap", "Gel", "Pipe", "None"}."None" ("Object recognition mode") enum16{"Ball", "Soap", "Gel", "Pipe", "None"}."None" ("Object recognition mode") enum16{"Ball", "Soap", "Gel", "Pipe", "None"}."None" ("Object recognition mode") enum16{"Ball", "Soap", "Gel", "Pipe", "None"}."Ball" ("Object recognition mode") enum16{"Ball", "Soap", "Gel", "Pipe", "None"}."Gel" ("Object recognition mode") enum16{"Ball", "Soap", "Gel", "Pipe", "None"}."Pipe" ("Object recognition mode") enum16{"Ball", "Soap", "Gel", "Pipe", "None"}."Soap" ("Object recognition mode") enum16{"Ball", "Soap", "Gel", "Pipe", "None"}."None" ("Object recognition mode") enum16{"Ball", "Soap", "Gel", "Pipe", "None"}."None" ("Object recognition mode") enum16{"Ball", "Soap", "Gel", "Pipe", "None"}."None" ("Object recognition mode") enum16{"Ball", "Soap", "Gel", "Pipe", "None"}."None" ("Object recognition mode")] -> w360
              frame "Start Task 1" {
                n205 = for {
                  shift-right: [w379] -> w374
                  shift-left: w375 -> [w378]
                  tunnel: string[] ["RESET ENCODERS", "RESET YAW", "FORWARD", "READ ENCODERS"] -> [w377] mode=indexing
                  n206 = Enqueue Element(queue=w378, element=w377) -> (queue out=w379:refnum<queue>)  [unwired: 2 in, 2 out]
                }
              }
              frame "Start Task 2" {
                n207 = for {
                  shift-right: [w387] -> w382
                  shift-left: w383 -> [w386]
                  tunnel: string[] ["RESET ENCODERS", "RESET YAW", "READ ULTRASONIC", "ARDUINO - ULTRASONIC"] -> [w385] mode=indexing
                  n208 = Enqueue Element(queue=w386, element=w385) -> (queue out=w387:refnum<queue>)  [unwired: 2 in, 2 out]
                }
              }
              frame "Start Task 3" {
                n209 = for {
                  shift-right: [w395] -> w390
                  shift-left: w391 -> [w394]
                  tunnel: string[] ["RESET ENCODERS", "READ ENCODERS", "R-ACW"] -> [w393] mode=indexing
                  n210 = Enqueue Element(queue=w394, element=w393) -> (queue out=w395:refnum<queue>)  [unwired: 2 in, 2 out]
                }
              }
              frame "Start Task 4" {
                n211 = for {
                  shift-right: [w403] -> w398
                  shift-left: w399 -> [w402]
                  tunnel: string[] ["RESET YAW", "RESET ENCODERS", "RESET ARM", "RESET FLAGS", "", ""] -> [w401] mode=indexing
                  n212 = Enqueue Element(queue=w402, element=w401) -> (queue out=w403:refnum<queue>)  [unwired: 2 in, 2 out]
                }
              }
              frame "Start Task 5" {
                n213 = for {
                  shift-right: [w411] -> w406
                  shift-left: w407 -> [w410]
                  tunnel: string[] ["RESET YAW", "RESET ENCODERS", "READ STEPPER VALUES", "Z STEPPER CAM HEIGHT", "", ""] -> [w409] mode=indexing
                  n214 = Enqueue Element(queue=w410, element=w409) -> (queue out=w411:refnum<queue>)  [unwired: 2 in, 2 out]
                }
              }
              frame "Start Task 6" {
                n215 = for {
                  shift-right: [w419] -> w414
                  shift-left: w415 -> [w418]
                  tunnel: string[] ["OPEN LOG CAM ", "", "", "", "", ""] -> [w417] mode=indexing
                  n216 = Enqueue Element(queue=w418, element=w417) -> (queue out=w419:refnum<queue>)  [unwired: 2 in, 2 out]
                }
              }
              frame "Start Task 8 - BALL" {
                n217 = for {
                  shift-right: [w427] -> w422
                  shift-left: w423 -> [w426]
                  tunnel: string[] ["RESET YAW", "RESET ENCODERS", "RESET ARM", "RESET FLAGS"] -> [w425] mode=indexing
                  n218 = Enqueue Element(queue=w426, element=w425) -> (queue out=w427:refnum<queue>)  [unwired: 2 in, 2 out]
                }
              }
              frame "Start Task 8 - Gel" {
                n219 = for {
                  shift-right: [w435] -> w430
                  shift-left: w431 -> [w434]
                  tunnel: string[] ["RESET YAW", "RESET ENCODERS", "RESET ARM", "RESET FLAGS"] -> [w433] mode=indexing
                  n220 = Enqueue Element(queue=w434, element=w433) -> (queue out=w435:refnum<queue>)  [unwired: 2 in, 2 out]
                }
              }
              frame "Start Task 8 - Pipe" {
                n221 = for {
                  shift-right: [w443] -> w438
                  shift-left: w439 -> [w442]
                  tunnel: string[] ["RESET YAW", "RESET ENCODERS", "RESET ARM", "RESET FLAGS"] -> [w441] mode=indexing
                  n222 = Enqueue Element(queue=w442, element=w441) -> (queue out=w443:refnum<queue>)  [unwired: 2 in, 2 out]
                }
              }
              frame "Start Task 8 - Soap" {
                n223 = for {
                  shift-right: [w451] -> w445
                  shift-left: w446 -> [w450]
                  tunnel: string[] ["RESET YAW", "RESET ENCODERS", "RESET ARM", "RESET FLAGS"] -> [w449] mode=indexing
                  n224 = Enqueue Element(queue=w450, element=w449) -> (queue out=w451:refnum<queue>)  [unwired: 2 in, 2 out]
                }
              }
              frame "Start Task 9" {
                n225 = for {
                  shift-right: [w459] -> w455
                  shift-left: w454 -> [w458]
                  tunnel: string[] ["RESET ENCODERS", "READ ENCODERS", "Z STEPPER BOX HEIGHT"] -> [w457] mode=indexing
                  n226 = Enqueue Element(queue=w458, element=w457) -> (queue out=w459:refnum<queue>)  [unwired: 2 in, 2 out]
                }
              }
              frame "Start Task A" {
                n227 = for {
                  shift-right: [w467] -> w463
                  shift-left: w462 -> [w466]
                  tunnel: string[] ["RESET ENCODERS", "READ ENCODERS", "RESET YAW", "Z STEPPER BOX HEIGHT"] -> [w465] mode=indexing
                  n228 = Enqueue Element(queue=w466, element=w465) -> (queue out=w467:refnum<queue>)  [unwired: 2 in, 2 out]
                }
              }
              frame "None", Default {
              }
              frame "Exit" {
                n229 = for {
                  shift-right: [w478] -> w473
                  shift-left: w474 -> [w477]
                  tunnel: string[] ["STOP", "RESET ENCODERS", "RESET YAW", "EXIT"] -> [w476] mode=indexing
                  n230 = Enqueue Element(queue=w477, element=w476) -> (queue out=w478:refnum<queue>)  [unwired: 2 in, 2 out]
                }
              }
            }
          }
          frame 5 {
            # ">> Item Selection Bias >>"
            # ">>> yStepper command>>>"
            n231 = for {
              shift-right: [w489] -> w483
              shift-left: w485 -> [w488]
              tunnel: string[] ["INIT", "RESET ENCODERS", "RESET FLAGS", "CAM CLOSE", "DISPOSE BUFFERS", "EXIT", ""] -> [w487] mode=indexing
              n232 = Enqueue Element(queue=w488, element=w487) -> (queue out=w489:refnum<queue>)  [unwired: 2 in, 2 out]
            }
          }
          frame 6 {
            # ">>> Motor control cluster >>>"
            # ">> Line detection >>"
            # ">> Checks if 1 metre moved >>"
            # ">>> yStepper command>>>"
            # "Use 250"
            n233 = Greater?(x=w499, y=265.0) -> (0:w493:bool)
            n234 = Dequeue Element(queue=w506, timeout in ms (-1)=w505, error in (no error)=w504) -> (element=w503:T8)  [unwired: 3 out]
            n235 = And(x=w492, y=w493) -> (x .and. y?=w490:bool)
            n236 = case shown="\"Start Task 1\", Default" w503 {
              tunnel: w491 -> [w507 _]
              tunnel: [w517 State_Type_Definitions,_for_0.26g_versions_and_later_2."True Stop" ("Enum")] -> w502
              tunnel: w501 -> [w515 w532]
              tunnel: [w514 w531] -> w500
              tunnel: [State_Type_Definitions,_for_0.26g_versions_and_later_2."Idle" ("Enum") State_Type_Definitions,_for_0.26g_versions_and_later_2."Shutdown" ("Enum")] -> w497
              tunnel: w490 -> [w508 _]
              frame "Start Task 1", Default {
                n237 = Or(x=w508, y=w507) -> (x .or. y?=w509:bool)
                n238 = case shown="True" w509 {
                  tunnel: w515 -> [w520 w526]
                  tunnel: [w519 w524] -> w514
                  frame False {
                    n239 = for {
                      shift-right: [w522] -> w519
                      shift-left: w520 -> [w523]
                      tunnel: string[] ["READ ENCODERS", "READ NAVX", "FORWARD", "READ LINE SENSOR"] ("element") -> [w521] mode=indexing
                      n240 = Enqueue Element(queue=w523, element=w521) -> (queue out=w522:refnum<queue>)  [unwired: 2 in, 2 out]
                    }
                  }
                  frame True {
                    n241 = for {
                      shift-right: [w528] -> w524
                      shift-left: w526 -> [w529]
                      tunnel: string[] ["RESET YAW", "RESET ENCODERS", "STOP", ""] -> [w527] mode=indexing
                      n242 = Enqueue Element(queue=w529, element=w527) -> (queue out=w528:refnum<queue>)  [unwired: 2 in, 2 out]
                    }
                  }
                }
                n243 = Select(t=State_Type_Definitions,_for_0.26g_versions_and_later_2."True Stop" ("Enum"), s=w507, f=State_Type_Definitions,_for_0.26g_versions_and_later_2."Task 1B" ("Enum")) -> (s? t:f=w512:T16)
                n244 = Select(t=w512, s=w508, f=State_Type_Definitions,_for_0.26g_versions_and_later_2."Task 1A" ("Enum")) -> (s? t:f=w517:T16)
              }
              frame "Exit" {
                n245 = for {
                  shift-right: [w536] -> w531
                  shift-left: w532 -> [w537]
                  tunnel: string[] ["STOP", "RESET ENCODERS", "RESET YAW", ""] -> [w535] mode=indexing
                  n246 = Enqueue Element(queue=w537, element=w535) -> (queue out=w536:refnum<queue>)  [unwired: 2 in, 2 out]
                }
              }
            }
          }
          frame 7 {
            # ">>> Motor control cluster >>>"
            # ">> Line detection >>"
            # ">> Adds small distance overhead after 1M >>"
            # ">>> yStepper command>>>"
            n247 = Greater?(x=w544, y=50.0) -> (0:w538:bool)
            n248 = Dequeue Element(queue=w553, timeout in ms (-1)=w552, error in (no error)=w551) -> (element=w550:T8)  [unwired: 3 out]
            n249 = Or(x=w538, y=w545) -> (x .or. y?=w549:bool)
            n250 = case shown="\"Start Task 1\", Default" w550 {
              tunnel: w549 -> [w556 _]
              tunnel: [w560 State_Type_Definitions,_for_0.26g_versions_and_later_2."True Stop" ("Enum")] -> w548
              tunnel: w547 -> [w557 w575]
              tunnel: [w555 w574] -> w546
              tunnel: [State_Type_Definitions,_for_0.26g_versions_and_later_2."Idle" ("Enum") State_Type_Definitions,_for_0.26g_versions_and_later_2."Shutdown" ("Enum")] -> w542
              frame "Start Task 1", Default {
                n251 = case shown="True" w556 {
                  tunnel: w557 -> [w563 w569]
                  tunnel: [w562 w567] -> w555
                  frame False {
                    n252 = for {
                      shift-right: [w565] -> w562
                      shift-left: w563 -> [w566]
                      tunnel: string[] ["READ ENCODERS", "READ NAVX", "FORWARD", "READ LINE SENSOR"] ("element") -> [w564] mode=indexing
                      n253 = Enqueue Element(queue=w566, element=w564) -> (queue out=w565:refnum<queue>)  [unwired: 2 in, 2 out]
                    }
                  }
                  frame True {
                    n254 = for {
                      shift-right: [w571] -> w567
                      shift-left: w569 -> [w572]
                      tunnel: string[] ["RESET YAW", "RESET ENCODERS", "STOP", ""] -> [w570] mode=indexing
                      n255 = Enqueue Element(queue=w572, element=w570) -> (queue out=w571:refnum<queue>)  [unwired: 2 in, 2 out]
                    }
                  }
                }
                n256 = Select(t=State_Type_Definitions,_for_0.26g_versions_and_later_2."True Stop" ("Enum"), s=w556, f=State_Type_Definitions,_for_0.26g_versions_and_later_2."Task 1B" ("Enum")) -> (s? t:f=w560:T16)
              }
              frame "Exit" {
                n257 = for {
                  shift-right: [w579] -> w574
                  shift-left: w575 -> [w580]
                  tunnel: string[] ["STOP", "RESET ENCODERS", "RESET YAW", ""] -> [w578] mode=indexing
                  n258 = Enqueue Element(queue=w580, element=w578) -> (queue out=w579:refnum<queue>)  [unwired: 2 in, 2 out]
                }
              }
            }
          }
          frame 8 {
            # ">> Stepper height reeached >>"
            # ">>> yStepper command>>>"
            # ">> Manual override >>"
            n259 = Dequeue Element(queue=w586, timeout in ms (-1)=w585, error in (no error)=w584) -> (element=w595:T8)  [unwired: 3 out]
            n260 = Equal?(x=w588, y=u8 60) -> (x = y?=w593:bool)
            n261 = case shown="\"Start Task 1\", Default" w595 {
              tunnel: [w606 State_Type_Definitions,_for_0.26g_versions_and_later_2."True Stop" ("Enum")] -> w590
              tunnel: [w604 w621] -> w583
              tunnel: w592 -> [w603 _]
              tunnel: w591 -> [w597 _]
              tunnel: [State_Type_Definitions,_for_0.26g_versions_and_later_2."Idle" ("Enum") State_Type_Definitions,_for_0.26g_versions_and_later_2."Shutdown" ("Enum")] -> w589
              tunnel: w593 -> [w596 _]
              frame "Start Task 1", Default {
                # ">> WIill proceed to part ii if not manual override >>"
                # ">>If ENABLE or Trigger is set to true>>"
                n262 = Or(x=w596, y=w597) -> (x .or. y?=w598:bool)
                n263 = case shown="True" w596 {
                  tunnel: [w609 w615] -> w604
                  tunnel: w603 -> [w608 w614]
                  frame False {
                    n264 = for {
                      shift-right: [w611] -> w609
                      shift-left: w608 -> [w612]
                      tunnel: string[] ["Z STEPPER CAM HEIGHT", "READ STEPPER VALUES"] ("element") -> [w610] mode=indexing
                      n265 = Enqueue Element(queue=w612, element=w610) -> (queue out=w611:refnum<queue>)  [unwired: 2 in, 2 out]
                    }
                  }
                  frame True {
                    n266 = for {
                      shift-right: [w617] -> w615
                      shift-left: w614 -> [w618]
                      tunnel: string[] ["ARDUINO - ULTRASONIC", "READ ULTRASONIC", "", "", "", ""] -> [w616] mode=indexing
                      n267 = Enqueue Element(queue=w618, element=w616) -> (queue out=w617:refnum<queue>)  [unwired: 2 in, 2 out]
                    }
                  }
                }
                n268 = Select(t=State_Type_Definitions,_for_0.26g_versions_and_later_2."True Stop" ("Enum"), s=w597, f=State_Type_Definitions,_for_0.26g_versions_and_later_2."Task 2:Sensor Mode" ("Enum")) -> (s? t:f=w600:T16)
                n269 = Select(t=w600, s=w598, f=State_Type_Definitions,_for_0.26g_versions_and_later_2."Task 2:Raise Arm" ("Enum")) -> (s? t:f=w606:T16)
              }
              frame "Exit" {
                n270 = for {
                  shift-right: [w624] -> w621
                  shift-left: _ -> [w625]
                  tunnel: string[] ["STOP", "RESET ENCODERS", "RESET YAW", ""] -> [w623] mode=indexing
                  n271 = Enqueue Element(queue=w625, element=w623) -> (queue out=w624:refnum<queue>)  [unwired: 2 in, 2 out]
                }
              }
            }
          }
          frame 9 {
            w642 = u8 20 ("y")
            # ">>> yStepper command>>>"
            # ">>Object detected>>"
            n272 = Dequeue Element(queue=w634, timeout in ms (-1)=w633, error in (no error)=w632) -> (element=w643:T8)  [unwired: 3 out]
            n273 = Less?(x=w630, y=w642) -> (x < y?=w641:bool)
            n274 = Less?(x=w629, y=w642) -> (x < y?=w640:bool)
            n275 = Or(x=w641, y=w640) -> (x .or. y?=w639:bool)
            "Obstacle detected" <- w639
            n276 = case shown="\"Start Task 1\", Default" w643 {
              tunnel: w639 -> [w646 _]
              tunnel: [w653 State_Type_Definitions,_for_0.26g_versions_and_later_2."True Stop" ("Enum")] -> w638
              tunnel: w631 -> [w645 _]
              tunnel: w635 -> [w652 w669]
              tunnel: [w651 w670] -> w637
              tunnel: [State_Type_Definitions,_for_0.26g_versions_and_later_2."Idle" ("Enum") State_Type_Definitions,_for_0.26g_versions_and_later_2."Shutdown" ("Enum")] -> w636
              frame "Start Task 1", Default {
                n277 = case shown="False" w646 {
                  tunnel: w652 -> [w656 w663]
                  tunnel: [w657 w662] -> w651
                  frame False {
                    n278 = for {
                      tunnel: string[] ["READ ULTRASONIC", "STOP"] ("element") -> [w658] mode=indexing
                      shift-right: [w660] -> w657
                      shift-left: w656 -> [w659]
                      n279 = Enqueue Element(queue=w659, element=w658) -> (queue out=w660:refnum<queue>)  [unwired: 2 in, 2 out]
                    }
                  }
                  frame True {
                    n280 = for {
                      shift-right: [w665] -> w662
                      shift-left: w663 -> [w666]
                      tunnel: string[] ["RESET ENCODERS", "READ NAVX", "READ ENCODERS"] -> [w664] mode=indexing
                      n281 = Enqueue Element(queue=w666, element=w664) -> (queue out=w665:refnum<queue>)  [unwired: 2 in, 2 out]
                    }
                  }
                }
                n282 = Or(x=w646, y=w645) -> (x .or. y?=w644:bool)
                n283 = Select(t=State_Type_Definitions,_for_0.26g_versions_and_later_2."True Stop" ("Enum"), s=w645, f=State_Type_Definitions,_for_0.26g_versions_and_later_2."Task 2:Reverse Mode" ("Enum")) -> (s? t:f=w647:T16)
                n284 = Select(t=w647, s=w644, f=State_Type_Definitions,_for_0.26g_versions_and_later_2."Task 2:Sensor Mode" ("Enum")) -> (s? t:f=w653:T16)
              }
              frame "Exit" {
                n285 = for {
                  shift-right: [w673] -> w670
                  shift-left: w669 -> [w674]
                  tunnel: string[] ["STOP", "RESET ENCODERS", "RESET YAW", "ARDUINO MODE 0"] -> [w672] mode=indexing
                  n286 = Enqueue Element(queue=w674, element=w672) -> (queue out=w673:refnum<queue>)  [unwired: 2 in, 2 out]
                }
              }
            }
          }
          frame 10 {
            # ">>> yStepper command>>>"
            n287 = Dequeue Element(queue=w685, timeout in ms (-1)=w686, error in (no error)=w687) -> (element=w689:T8)  [unwired: 3 out]
            n288 = Less?(x=w679, y=-50.0) -> (x < y?=w677:bool)
            n289 = case shown="\"Start Task 1\", Default" w689 {
              tunnel: [w699 State_Type_Definitions,_for_0.26g_versions_and_later_2."True Stop" ("Enum")] -> w681
              tunnel: w688 -> [w692 _]
              tunnel: w684 -> [w698 w715]
              tunnel: [w697 w716] -> w680
              tunnel: [State_Type_Definitions,_for_0.26g_versions_and_later_2."Idle" ("Enum") State_Type_Definitions,_for_0.26g_versions_and_later_2."Shutdown" ("Enum")] -> w682
              tunnel: w677 -> [w690 _]
              frame "Start Task 1", Default {
                n290 = case shown="True" w690 {
                  tunnel: w698 -> [w702 w709]
                  tunnel: [w703 w708] -> w697
                  frame False {
                    n291 = for {
                      tunnel: string[] ["READ ENCODERS", "REVERSE", "READ NAVX"] ("element") -> [w704] mode=indexing
                      shift-right: [w706] -> w703
                      shift-left: w702 -> [w705]
                      n292 = Enqueue Element(queue=w705, element=w704) -> (queue out=w706:refnum<queue>)  [unwired: 2 in, 2 out]
                    }
                  }
                  frame True {
                    n293 = for {
                      shift-right: [w711] -> w708
                      shift-left: w709 -> [w712]
                      tunnel: string[] ["STOP", "ARDUINO - ULTRASONIC", "READ ULTRASONIC", "RESET ENCODERS"] -> [w710] mode=indexing
                      n294 = Enqueue Element(queue=w712, element=w710) -> (queue out=w711:refnum<queue>)  [unwired: 2 in, 2 out]
                    }
                  }
                }
                n295 = Or(x=w690, y=w692) -> (x .or. y?=w691:bool)
                n296 = Select(t=State_Type_Definitions,_for_0.26g_versions_and_later_2."True Stop" ("Enum"), s=w692, f=State_Type_Definitions,_for_0.26g_versions_and_later_2."Task 2:Sensor Mode" ("Enum")) -> (s? t:f=w693:T16)
                n297 = Select(t=w693, s=w691, f=State_Type_Definitions,_for_0.26g_versions_and_later_2."Task 2:Reverse Mode" ("Enum")) -> (s? t:f=w699:T16)
              }
              frame "Exit" {
                n298 = for {
                  shift-right: [w719] -> w716
                  shift-left: w715 -> [w720]
                  tunnel: string[] ["STOP", "RESET ENCODERS", "RESET YAW", "ARDUINO MODE 0"] -> [w718] mode=indexing
                  n299 = Enqueue Element(queue=w720, element=w718) -> (queue out=w719:refnum<queue>)  [unwired: 2 in, 2 out]
                }
              }
            }
          }
          frame 11 {
            # ">>> Motor control cluster >>>"
            # ">>> yStepper command>>>"
            n300 = Dequeue Element(queue=w736, timeout in ms (-1)=w735, error in (no error)=w734) -> (element=w725:T8)  [unwired: 3 out]
            n301 = Less?(x=w733, y=-160.0) -> (x < y?=w730:bool)
            n302 = Or(x=w730, y=w731) -> (x .or. y?=w726:bool)
            n303 = case shown="\"Start Task 1\", Default" w725 {
              tunnel: w726 -> [w739 _]
              tunnel: [w743 State_Type_Definitions,_for_0.26g_versions_and_later_2."True Stop" ("Enum")] -> w727
              tunnel: w729 -> [w740 w759]
              tunnel: [w738 w758] -> w728
              tunnel: [State_Type_Definitions,_for_0.26g_versions_and_later_2."Idle" ("Enum") State_Type_Definitions,_for_0.26g_versions_and_later_2."Shutdown" ("Enum")] -> w724
              frame "Start Task 1", Default {
                n304 = case shown="False" w739 {
                  tunnel: w740 -> [w746 w752]
                  tunnel: [w745 w750] -> w738
                  frame False {
                    n305 = for {
                      shift-right: [w748] -> w745
                      shift-left: w746 -> [w749]
                      tunnel: string[] ["READ ENCODERS", "R-CW"] ("element") -> [w747] mode=indexing
                      n306 = Enqueue Element(queue=w749, element=w747) -> (queue out=w748:refnum<queue>)  [unwired: 2 in, 2 out]
                    }
                  }
                  frame True {
                    n307 = for {
                      shift-right: [w754] -> w750
                      shift-left: w752 -> [w755]
                      tunnel: string[] ["RESET YAW", "RESET ENCODERS", "STOP", "ARDUINO MODE 0"] -> [w753] mode=indexing
                      n308 = Enqueue Element(queue=w755, element=w753) -> (queue out=w754:refnum<queue>)  [unwired: 2 in, 2 out]
                    }
                  }
                }
                n309 = Select(t=State_Type_Definitions,_for_0.26g_versions_and_later_2."True Stop" ("Enum"), s=w739, f=State_Type_Definitions,_for_0.26g_versions_and_later_2."Task 3" ("Enum")) -> (s? t:f=w743:T16)
              }
              frame "Exit" {
                n310 = for {
                  shift-right: [w762] -> w758
                  shift-left: w759 -> [w763]
                  tunnel: string[] ["STOP", "RESET ENCODERS", "RESET YAW", ""] -> [w761] mode=indexing
                  n311 = Enqueue Element(queue=w763, element=w761) -> (queue out=w762:refnum<queue>)  [unwired: 2 in, 2 out]
                }
              }
            }
          }
          frame 12 {
            # ">> Stepper height reeached >>"
            # ">>> yStepper command>>>"
            # ">> Manual override >>"
            n312 = Dequeue Element(queue=w777, timeout in ms (-1)=w776, error in (no error)=w775) -> (element=w774:T8)  [unwired: 3 out]
            n313 = Equal?(x=w768, y=u8 60) -> (x = y?=w766:bool)
            n314 = case shown="\"Start Task 1\", Default" w774 {
              tunnel: [w789 State_Type_Definitions,_for_0.26g_versions_and_later_2."True Stop" ("Enum")] -> w773
              tunnel: [w787 w805] -> w772
              tunnel: w778 -> [w786 w802]
              tunnel: w771 -> [w780 _]
              tunnel: [State_Type_Definitions,_for_0.26g_versions_and_later_2."Idle" ("Enum") State_Type_Definitions,_for_0.26g_versions_and_later_2."Shutdown" ("Enum")] -> w770
              tunnel: w766 -> [w779 _]
              frame "Start Task 1", Default {
                # ">> WIill proceed to part ii if not manual override >>"
                # ">>If ENABLE or Trigger is set to true>>"
                n315 = Or(x=w779, y=w780) -> (x .or. y?=w781:bool)
                n316 = case shown="False" w779 {
                  tunnel: [w792 w798] -> w787
                  tunnel: w786 -> [w791 w797]
                  frame False {
                    n317 = for {
                      shift-right: [w794] -> w792
                      shift-left: w791 -> [w795]
                      tunnel: string[] ["Z STEPPER CAM HEIGHT", "READ STEPPER VALUES"] ("element") -> [w793] mode=indexing
                      n318 = Enqueue Element(queue=w795, element=w793) -> (queue out=w794:refnum<queue>)  [unwired: 2 in, 2 out]
                    }
                  }
                  frame True {
                    n319 = for {
                      shift-right: [w800] -> w798
                      shift-left: w797 -> [w801]
                      tunnel: string[] ["ARDUINO - ULTRASONIC", "READ ULTRASONIC", "FORWARD", "", "", ""] -> [w799] mode=indexing
                      n320 = Enqueue Element(queue=w801, element=w799) -> (queue out=w800:refnum<queue>)  [unwired: 2 in, 2 out]
                    }
                  }
                }
                n321 = Select(t=State_Type_Definitions,_for_0.26g_versions_and_later_2."True Stop" ("Enum"), s=w780, f=State_Type_Definitions,_for_0.26g_versions_and_later_2."Task 4_B" ("Enum")) -> (s? t:f=w783:T16)
                n322 = Select(t=w783, s=w781, f=State_Type_Definitions,_for_0.26g_versions_and_later_2."Task 4_A" ("Enum")) -> (s? t:f=w789:T16)
              }
              frame "Exit" {
                n323 = for {
                  shift-right: [w808] -> w805
                  shift-left: w802 -> [w809]
                  tunnel: string[] ["STOP", "RESET ENCODERS", "RESET YAW", ""] -> [w807] mode=indexing
                  n324 = Enqueue Element(queue=w809, element=w807) -> (queue out=w808:refnum<queue>)  [unwired: 2 in, 2 out]
                }
              }
            }
          }
          frame 13 {
            w815 = u8 20
            # ">> Path blocked >>"
            # ">>> yStepper command>>>"
            # ">> Manual override >>"
            n325 = Dequeue Element(queue=w824, timeout in ms (-1)=w823, error in (no error)=w822) -> (element=w821:T8)  [unwired: 3 out]
            n326 = Less?(x=w817, y=w815) -> (x < y?=w812:bool)
            n327 = Less?(x=w816, y=w815) -> (x < y?=w813:bool)
            n328 = And(x=w813, y=w812) -> (x .and. y?=w814:bool)
            n329 = case shown="\"Start Task 1\", Default" w821 {
              tunnel: [w838 State_Type_Definitions,_for_0.26g_versions_and_later_2."True Stop" ("Enum")] -> w826
              tunnel: [w836 w853] -> w827
              tunnel: w820 -> [w835 _]
              tunnel: w825 -> [w829 _]
              tunnel: [State_Type_Definitions,_for_0.26g_versions_and_later_2."Idle" ("Enum") State_Type_Definitions,_for_0.26g_versions_and_later_2."Shutdown" ("Enum")] -> w819
              tunnel: w814 -> [w828 _]
              frame "Start Task 1", Default {
                # ">> Manual override forces program to true stop >>"
                # ">>If ENABLE or Trigger is set to true>>"
                n330 = Or(x=w828, y=w829) -> (x .or. y?=w834:bool)
                n331 = case shown="False" w828 {
                  tunnel: [w841 w846] -> w836
                  tunnel: w835 -> [w840 w845]
                  frame False {
                    n332 = for {
                      shift-right: [w843] -> w841
                      shift-left: w840 -> [w844]
                      tunnel: string[] ["FORWARD", "READ ULTRASONIC", "READ NAVX"] ("element") -> [w842] mode=indexing
                      n333 = Enqueue Element(queue=w844, element=w842) -> (queue out=w843:refnum<queue>)  [unwired: 2 in, 2 out]
                    }
                  }
                  frame True {
                    n334 = for {
                      shift-right: [w849] -> w846
                      shift-left: w845 -> [w850]
                      tunnel: string[] ["STOP", "RESET YAW", "RESET ENCODERS", "RESET FLAGS"] -> [w848] mode=indexing
                      n335 = Enqueue Element(queue=w850, element=w848) -> (queue out=w849:refnum<queue>)  [unwired: 2 in, 2 out]
                    }
                  }
                }
                n336 = Select(t=State_Type_Definitions,_for_0.26g_versions_and_later_2."True Stop" ("Enum"), s=w829, f=State_Type_Definitions,_for_0.26g_versions_and_later_2."Task 4_C" ("Enum")) -> (s? t:f=w831:T16)
                n337 = Select(t=w831, s=w834, f=State_Type_Definitions,_for_0.26g_versions_and_later_2."Task 4_B" ("Enum")) -> (s? t:f=w838:T16)
              }
              frame "Exit" {
                n338 = for {
                  shift-right: [w856] -> w853
                  shift-left: _ -> [w857]
                  tunnel: string[] ["STOP", "RESET ENCODERS", "RESET YAW", ""] -> [w855] mode=indexing
                  n339 = Enqueue Element(queue=w857, element=w855) -> (queue out=w856:refnum<queue>)  [unwired: 2 in, 2 out]
                }
              }
            }
          }
          frame 14 {
            w869 = u8 20
            # ">> xDistance travelled>>"
            # ">> Path NOT blocked >>"
            # ">>> yStepper command>>>"
            # ">> Manual override >>"
            n340 = Dequeue Element(queue=w879, timeout in ms (-1)=w872, error in (no error)=w871) -> (element=w873:T8)  [unwired: 3 out]
            n341 = Greater?(x=w861, y=w869) -> (0:w867:bool)
            n342 = Greater?(x=w866, y=80.0) -> (0:w864:bool)
            n343 = Greater?(x=w860, y=w869) -> (0:w868:bool)
            n344 = And(x=w868, y=w867) -> (x .and. y?=w863:bool)
            n345 = And(x=w864, y=w863) -> (x .and. y?=w862:bool)
            n346 = case shown="\"Start Task 1\", Default" w873 {
              tunnel: [w890 State_Type_Definitions,_for_0.26g_versions_and_later_2."True Stop" ("Enum")] -> w876
              tunnel: [w888 w906] -> w875
              tunnel: w878 -> [w887 w903]
              tunnel: w877 -> [w881 _]
              tunnel: [State_Type_Definitions,_for_0.26g_versions_and_later_2."Idle" ("t") State_Type_Definitions,_for_0.26g_versions_and_later_2."Shutdown" ("Enum")] -> w874
              tunnel: w862 -> [w880 _]
              frame "Start Task 1", Default {
                # ">> Manual override forces program to true stop >>"
                # ">>If ENABLE or Trigger is set to true>>"
                n347 = Or(x=w880, y=w881) -> (x .or. y?=w886:bool)
                n348 = case shown="False" w880 {
                  tunnel: [w893 w898] -> w888
                  tunnel: w887 -> [w891 w897]
                  frame False {
                    n349 = for {
                      shift-right: [w895] -> w893
                      shift-left: w891 -> [w896]
                      tunnel: string[] ["RIGHT", "READ NAVX", "READ ENCODERS", "READ ULTRASONIC"] ("element") -> [w894] mode=indexing
                      n350 = Enqueue Element(queue=w896, element=w894) -> (queue out=w895:refnum<queue>)  [unwired: 2 in, 2 out]
                    }
                  }
                  frame True {
                    n351 = for {
                      shift-right: [w901] -> w898
                      shift-left: w897 -> [w902]
                      tunnel: string[] ["STOP", "RESET YAW", "RESET ENCODERS", "ARDUINO - ULTRASONIC"] -> [w900] mode=indexing
                      n352 = Enqueue Element(queue=w902, element=w900) -> (queue out=w901:refnum<queue>)  [unwired: 2 in, 2 out]
                    }
                  }
                }
                n353 = Select(t=State_Type_Definitions,_for_0.26g_versions_and_later_2."True Stop" ("Enum"), s=w881, f=State_Type_Definitions,_for_0.26g_versions_and_later_2."Task 4_D" ("Enum")) -> (s? t:f=w882:T16)
                n354 = Select(t=w882, s=w886, f=State_Type_Definitions,_for_0.26g_versions_and_later_2."Task 4_C" ("Enum")) -> (s? t:f=w890:T16)
              }
              frame "Exit" {
                n355 = for {
                  shift-right: [w909] -> w906
                  shift-left: w903 -> [w910]
                  tunnel: string[] ["STOP", "RESET ENCODERS", "RESET YAW", ""] -> [w908] mode=indexing
                  n356 = Enqueue Element(queue=w910, element=w908) -> (queue out=w909:refnum<queue>)  [unwired: 2 in, 2 out]
                }
              }
            }
          }
          frame 15 {
            w933 = u8 20
            # ">>> Motor control cluster >>>"
            # ">> Line detected >>"
            # ">> yDistance travelled>>"
            # ">> Path blocked >>"
            # ">>> yStepper command>>>"
            # ">> Manual override >>"
            n357 = Less?(x=w918, y=w933) -> (x < y?=w931:bool)
            n358 = Greater?(x=w922, y=200.0) -> (0:w929:bool)
            n359 = Less?(x=w917, y=w933) -> (x < y?=w932:bool)
            n360 = And(x=w932, y=w931) -> (x .and. y?=w928:bool)
            n361 = Dequeue Element(queue=w925, timeout in ms (-1)=w924, error in (no error)=w923) -> (element=w934:T8)  [unwired: 3 out]
            n362 = Or(x=w929, y=w928) -> (x .or. y?=w912:bool)
            n363 = And(x=w913, y=w912) -> (x .and. y?=w911:bool)
            n364 = case shown="\"Start Task 1\", Default" w934 {
              tunnel: [w945 State_Type_Definitions,_for_0.26g_versions_and_later_2."True Stop" ("Enum")] -> w921
              tunnel: [w943 w961] -> w919
              tunnel: w926 -> [w942 w958]
              tunnel: w927 -> [w936 _]
              tunnel: [State_Type_Definitions,_for_0.26g_versions_and_later_2."Idle" ("t") State_Type_Definitions,_for_0.26g_versions_and_later_2."Shutdown" ("Enum")] -> w920
              tunnel: w911 -> [w935 _]
              frame "Start Task 1", Default {
                # ">> Manual override forces program to true stop >>"
                # ">>If ENABLE or Trigger is set to true>>"
                n365 = Or(x=w935, y=w936) -> (x .or. y?=w941:bool)
                n366 = case shown="False" w935 {
                  tunnel: [w948 w953] -> w943
                  tunnel: w942 -> [w946 w952]
                  frame False {
                    n367 = for {
                      shift-right: [w950] -> w948
                      shift-left: w946 -> [w951]
                      tunnel: string[] ["FORWARD", "READ NAVX", "READ ENCODERS", "READ ULTRASONIC", "READ LINE SENSOR"] ("element") -> [w949] mode=indexing
                      n368 = Enqueue Element(queue=w951, element=w949) -> (queue out=w950:refnum<queue>)  [unwired: 2 in, 2 out]
                    }
                  }
                  frame True {
                    n369 = for {
                      shift-right: [w956] -> w953
                      shift-left: w952 -> [w957]
                      tunnel: string[] ["STOP", "RESET YAW", "RESET ENCODERS", "RESET FLAGS"] -> [w955] mode=indexing
                      n370 = Enqueue Element(queue=w957, element=w955) -> (queue out=w956:refnum<queue>)  [unwired: 2 in, 2 out]
                    }
                  }
                }
                n371 = Select(t=State_Type_Definitions,_for_0.26g_versions_and_later_2."True Stop" ("Enum"), s=w936, f=State_Type_Definitions,_for_0.26g_versions_and_later_2."True Stop" ("Enum")) -> (s? t:f=w937:T16)
                n372 = Select(t=w937, s=w941, f=State_Type_Definitions,_for_0.26g_versions_and_later_2."Task 4_D" ("Enum")) -> (s? t:f=w945:T16)
              }
              frame "Exit" {
                n373 = for {
                  shift-right: [w964] -> w961
                  shift-left: w958 -> [w965]
                  tunnel: string[] ["STOP", "RESET ENCODERS", "RESET YAW", ""] -> [w963] mode=indexing
                  n374 = Enqueue Element(queue=w965, element=w963) -> (queue out=w964:refnum<queue>)  [unwired: 2 in, 2 out]
                }
              }
            }
          }
          frame 16 {
            # ">>> Motor control cluster >>>"
            # ">>> yStepper command>>>"
            # ">> Manual override >>"
            n375 = Dequeue Element(queue=w976, timeout in ms (-1)=w975, error in (no error)=w977) -> (element=w974:T8)  [unwired: 3 out]
            n376 = Equal?(x=w973, y=u8 60) -> (x = y?=w971:bool)
            n377 = case shown="\"Start Task 1\", Default" w974 {
              tunnel: [w987 State_Type_Definitions,_for_0.26g_versions_and_later_2."True Stop" ("Enum")] -> w978
              tunnel: [w990 w1007] -> w979
              tunnel: [State_Type_Definitions,_for_0.26g_versions_and_later_2."Idle" ("Enum") State_Type_Definitions,_for_0.26g_versions_and_later_2."Shutdown" ("Enum")] -> w980
              tunnel: w971 -> [w986 _]
              tunnel: w970 -> [w985 _]
              tunnel: w969 -> [w981 w1004]
              frame "Start Task 1", Default {
                # "Stays in Task 5_A until stepper reaches desired \nheight"
                # "T: Go back to idle, F: Continue with task\""
                # ">> Manual override >>"
                n378 = case shown="True" w986 {
                  tunnel: [w994 w1000] -> w990
                  tunnel: w981 -> [w992 w998]
                  frame False {
                    n379 = for {
                      tunnel: string[] ["Z STEPPER CAM HEIGHT", "READ STEPPER VALUES"] ("element") -> [w995] mode=indexing
                      shift-right: [w997] -> w994
                      shift-left: w992 -> [w996]
                      n380 = Enqueue Element(queue=w996, element=w995) -> (queue out=w997:refnum<queue>)  [unwired: 2 in, 2 out]
                    }
                  }
                  frame True {
                    n381 = for {
                      shift-right: [w1002] -> w1000
                      shift-left: w998 -> [w1003]
                      tunnel: string[] ["ARDUINO - ULTRASONIC", "READ ULTRASONIC", ""] -> [w1001] mode=indexing
                      n382 = Enqueue Element(queue=w1003, element=w1001) -> (queue out=w1002:refnum<queue>)  [unwired: 2 in, 2 out]
                    }
                  }
                }
                n383 = Or(x=w986, y=w985) -> (x .or. y?=w988:bool)
                n384 = Select(t=State_Type_Definitions,_for_0.26g_versions_and_later_2."True Stop" ("Enum"), s=w985, f=State_Type_Definitions."Task 5B: MOVE TO BOX" ("Enum")) -> (s? t:f=w982:u16)
                n385 = Select(t=w982, s=w988, f=State_Type_Definitions."Task 5A: ARM CAM HEIGHT" ("Enum")) -> (s? t:f=w987:u16)
              }
              frame "Exit" {
                n386 = for {
                  shift-right: [w1010] -> w1007
                  shift-left: w1004 -> [w1011]
                  tunnel: string[] ["STOP", "RESET ENCODERS", "RESET YAW", "ARDUINO MODE 0"] -> [w1009] mode=indexing
                  n387 = Enqueue Element(queue=w1011, element=w1009) -> (queue out=w1010:refnum<queue>)  [unwired: 2 in, 2 out]
                }
              }
            }
          }
          frame 17 {
            w1019 = u8 20 ("y")
            # ">>> yStepper command>>>"
            n388 = Less?(x=w1016, y=w1019) -> (x < y?=w1017:bool)
            n389 = Dequeue Element(queue=w1023, timeout in ms (-1)=w1022, error in (no error)=w1024) -> (element=w1021:T8)  [unwired: 3 out]
            n390 = Less?(x=w1015, y=w1019) -> (x < y?=w1018:bool)
            n391 = And(x=w1018, y=w1017) -> (x .and. y?=w1014:bool)
            n392 = case shown="\"Start Task 1\", Default" w1021 {
              tunnel: [w1036 State_Type_Definitions,_for_0.26g_versions_and_later_2."True Stop" ("Enum")] -> w1026
              tunnel: [w1039 w1056] -> w1025
              tunnel: [State_Type_Definitions,_for_0.26g_versions_and_later_2."Idle" ("Enum") State_Type_Definitions,_for_0.26g_versions_and_later_2."Shutdown" ("Enum")] -> w1027
              tunnel: w1029 -> [w1035 _]
              tunnel: w1028 -> [w1031 w1053]
              tunnel: w1014 -> [w1030 _]
              frame "Start Task 1", Default {
                # "Stays in Task 5_B to capture image over 5 seconds"
                # "T: Go back to idle, F: Continue with task\""
                # ">> Manual override >>"
                n393 = case shown="True" w1030 {
                  tunnel: [w1043 w1049] -> w1039
                  tunnel: w1031 -> [w1041 w1047]
                  frame False {
                    n394 = for {
                      tunnel: string[] ["FORWARD", "READ ULTRASONIC", "READ NAVX"] ("element") -> [w1044] mode=indexing
                      shift-right: [w1046] -> w1043
                      shift-left: w1041 -> [w1045]
                      n395 = Enqueue Element(queue=w1045, element=w1044) -> (queue out=w1046:refnum<queue>)  [unwired: 2 in, 2 out]
                    }
                  }
                  frame True {
                    n396 = for {
                      shift-right: [w1051] -> w1049
                      shift-left: w1047 -> [w1052]
                      tunnel: string[] ["STOP", "RESET ENCODERS", "OPEN LOG CAM", "SET TIMER 5"] -> [w1050] mode=indexing
                      n397 = Enqueue Element(queue=w1052, element=w1050) -> (queue out=w1051:refnum<queue>)  [unwired: 2 in, 2 out]
                    }
                  }
                }
                n398 = Or(x=w1030, y=w1035) -> (x .or. y?=w1037:bool)
                n399 = Select(t=State_Type_Definitions,_for_0.26g_versions_and_later_2."True Stop" ("Enum"), s=w1035, f=State_Type_Definitions."Task 5C: CAM BURST" ("Enum")) -> (s? t:f=w1032:u16)
                n400 = Select(t=w1032, s=w1037, f=State_Type_Definitions."Task 5B: MOVE TO BOX" ("Enum")) -> (s? t:f=w1036:u16)
              }
              frame "Exit" {
                n401 = for {
                  shift-right: [w1059] -> w1056
                  shift-left: w1053 -> [w1060]
                  tunnel: string[] ["STOP", "RESET ENCODERS", "RESET YAW", "ARDUINO MODE 0"] -> [w1058] mode=indexing
                  n402 = Enqueue Element(queue=w1060, element=w1058) -> (queue out=w1059:refnum<queue>)  [unwired: 2 in, 2 out]
                }
              }
            }
          }
          frame 18 {
            # ">>> Motor control cluster >>>"
            # ">>> yStepper command>>>"
            # ">> Manual override >>"
            n403 = Dequeue Element(queue=w1071, timeout in ms (-1)=w1070, error in (no error)=w1069) -> (element=w1068:T8)  [unwired: 3 out]
            n404 = case shown="\"Start Task 1\", Default" w1068 {
              tunnel: [w1080 State_Type_Definitions,_for_0.26g_versions_and_later_2."True Stop" ("Enum")] -> w1073
              tunnel: [w1083 w1100] -> w1066
              tunnel: [State_Type_Definitions,_for_0.26g_versions_and_later_2."Idle" ("Enum") State_Type_Definitions,_for_0.26g_versions_and_later_2."Shutdown" ("Enum")] -> w1065
              tunnel: w1067 -> [w1074 _]
              tunnel: w1072 -> [w1079 w1097]
              tunnel: w1063 -> [w1078 _]
              frame "Start Task 1", Default {
                # ">> Is time up? >>"
                # "Determines if object is in range to pick up"
                # ">> Manual override >>"
                n405 = case shown="False" w1078 {
                  tunnel: [w1087 w1093] -> w1083
                  tunnel: w1079 -> [w1085 w1091]
                  frame False {
                    n406 = for {
                      tunnel: string[] ["CAM ACQ", "START TIMER"] ("element") -> [w1088] mode=indexing
                      shift-right: [w1090] -> w1087
                      shift-left: w1085 -> [w1089]
                      n407 = Enqueue Element(queue=w1089, element=w1088) -> (queue out=w1090:refnum<queue>)  [unwired: 2 in, 2 out]
                    }
                  }
                  frame True {
                    n408 = for {
                      shift-right: [w1095] -> w1093
                      shift-left: w1091 -> [w1096]
                      tunnel: string[] ["CAM CLOSE", "PROCESS IMAGE", "SET TIMER 5"] -> [w1094] mode=indexing
                      n409 = Enqueue Element(queue=w1096, element=w1094) -> (queue out=w1095:refnum<queue>)  [unwired: 2 in, 2 out]
                    }
                  }
                }
                n410 = Or(x=w1078, y=w1074) -> (x .or. y?=w1081:bool)
                n411 = Select(t=State_Type_Definitions,_for_0.26g_versions_and_later_2."True Stop" ("Enum"), s=w1074, f=State_Type_Definitions."Task 5D: PROCESS IMAGE" ("Enum")) -> (s? t:f=w1076:u16)
                n412 = Select(t=w1076, s=w1081, f=State_Type_Definitions."Task 5C: CAM BURST" ("Enum")) -> (s? t:f=w1080:u16)
              }
              frame "Exit" {
                n413 = for {
                  shift-right: [w1103] -> w1100
                  shift-left: w1097 -> [w1104]
                  tunnel: string[] ["STOP", "RESET ENCODERS", "RESET YAW", "ARDUINO MODE 0"] -> [w1102] mode=indexing
                  n414 = Enqueue Element(queue=w1104, element=w1102) -> (queue out=w1103:refnum<queue>)  [unwired: 2 in, 2 out]
                }
              }
            }
          }
          frame 19 {
            # ">>> yStepper command>>>"
            n415 = Dequeue Element(queue=w1112, timeout in ms (-1)=w1111, error in (no error)=w1110) -> (element=w1109:T8)  [unwired: 3 out]
            n416 = case shown="\"Exit\"" w1109 {
              tunnel: [w1124 State_Type_Definitions,_for_0.26g_versions_and_later_2."True Stop" ("Enum")] -> w1116
              tunnel: [w1127 w1144] -> w1115
              tunnel: [State_Type_Definitions,_for_0.26g_versions_and_later_2."Idle" ("Enum") State_Type_Definitions,_for_0.26g_versions_and_later_2."Shutdown" ("Enum")] -> w1117
              tunnel: w1113 -> [w1123 _]
              tunnel: w1114 -> [w1119 w1141]
              tunnel: w1107 -> [w1118 _]
              frame "Start Task 1", Default {
                # ">> T: Breaks out of state loop; F: Stays in loop>>"
                # ">> Manual override >>"
                # ">> Checks if time is up>>"
                # "Stays in Task 5D until the object is detected"
                # "T: Go back to idle, F: Continue with task\""
                # ">> Manual override >>"
                n417 = case shown="True" w1118 {
                  tunnel: [w1131 w1137] -> w1127
                  tunnel: w1119 -> [w1129 w1135]
                  frame False {
                    n418 = for {
                      tunnel: string[] ["START TIMER", "PROCESS IMAGE", ""] ("element") -> [w1132] mode=indexing
                      shift-right: [w1134] -> w1131
                      shift-left: w1129 -> [w1133]
                      n419 = Enqueue Element(queue=w1133, element=w1132) -> (queue out=w1134:refnum<queue>)  [unwired: 2 in, 2 out]
                    }
                  }
                  frame True {
                    n420 = for {
                      shift-right: [w1139] -> w1137
                      shift-left: w1135 -> [w1140]
                      tunnel: string[] ["CAM CLOSE", "", ""] -> [w1138] mode=indexing
                      n421 = Enqueue Element(queue=w1140, element=w1138) -> (queue out=w1139:refnum<queue>)  [unwired: 2 in, 2 out]
                    }
                  }
                }
                n422 = Or(x=w1118, y=w1123) -> (x .or. y?=w1125:bool)
                n423 = Select(t=State_Type_Definitions,_for_0.26g_versions_and_later_2."True Stop" ("Enum"), s=w1123, f=State_Type_Definitions,_for_0.26g_versions_and_later_2."Task 5E: POSITION ARM" ("Enum")) -> (s? t:f=w1120:T16)
                n424 = Select(t=w1120, s=w1125, f=State_Type_Definitions."Task 5D: PROCESS IMAGE" ("Enum")) -> (s? t:f=w1124:u16)
              }
              frame "Exit" {
                n425 = for {
                  shift-right: [w1147] -> w1144
                  shift-left: w1141 -> [w1148]
                  tunnel: string[] ["STOP", "RESET ENCODERS", "RESET YAW", "ARDUINO MODE 0"] -> [w1146] mode=indexing
                  n426 = Enqueue Element(queue=w1148, element=w1146) -> (queue out=w1147:refnum<queue>)  [unwired: 2 in, 2 out]
                }
              }
            }
          }
          frame 20 {
            # ">>> yStepper command>>>"
            n427 = Dequeue Element(queue=w1162, timeout in ms (-1)=w1163, error in (no error)=w1164) -> (element=w1166:T8)  [unwired: 3 out]
            n428 = formula code="if (pos < 100)\ny = 41;\n\nelse if (pos >= 100 && pos <= 140)\ny = 30;\n\nelse if (pos >= 141 && pos <= 170)\ny = 25;\n\nelse if (pos >= 171 &&pos <= 180) \ny = 20;\n\nelse if (pos >= 181&& pos <= 200)\ny = 15;\n\nelse if (pos >= 201 && pos <= 230)\ny = 10;\n\nelse if (pos >= 231 && pos <= 320)\ny = 8;\n\nelse if (pos > 320)\ny = 0;"("pos"=w1154) -> ("y"=w1157:dbl)
            n429 = To Unsigned Byte Integer(number=w1157) -> (unsigned 8bit integer=w1152:u8)
            n430 = Equal?(x=w1153, y=w1152) -> (x = y?=w1151:bool)
            n431 = case shown="\"Start Task 1\", Default" w1166 {
              tunnel: [w1173 State_Type_Definitions,_for_0.26g_versions_and_later_2."True Stop" ("Enum")] -> w1160
              tunnel: [w1176 w1193] -> w1158
              tunnel: [State_Type_Definitions,_for_0.26g_versions_and_later_2."Idle" ("Enum") State_Type_Definitions,_for_0.26g_versions_and_later_2."Shutdown" ("Enum")] -> w1159
              tunnel: w1165 -> [w1172 _]
              tunnel: w1161 -> [w1168 w1190]
              tunnel: w1151 -> [w1167 _]
              frame "Start Task 1", Default {
                # ">> T: Breaks out of state loop; F: Stays in loop>>"
                # ">> Manual override >>"
                # ">> Checks if time is up>>"
                # "Stays in Task 5D until the object is detected"
                # "T: Go back to idle, F: Continue with task\""
                # ">> Manual override >>"
                n432 = case shown="False" w1167 {
                  tunnel: [w1180 w1186] -> w1176
                  tunnel: w1168 -> [w1178 w1184]
                  frame False {
                    n433 = for {
                      tunnel: string[] ["READ STEPPER VALUES", "Y STEPPER CONTROL", ""] ("element") -> [w1181] mode=indexing
                      shift-right: [w1183] -> w1180
                      shift-left: w1178 -> [w1182]
                      n434 = Enqueue Element(queue=w1182, element=w1181) -> (queue out=w1183:refnum<queue>)  [unwired: 2 in, 2 out]
                    }
                  }
                  frame True {
                    n435 = for {
                      shift-right: [w1188] -> w1186
                      shift-left: w1184 -> [w1189]
                      tunnel: string[] ["CAM CLOSE", "DISPOSE BUFFERS", ""] -> [w1187] mode=indexing
                      n436 = Enqueue Element(queue=w1189, element=w1187) -> (queue out=w1188:refnum<queue>)  [unwired: 2 in, 2 out]
                    }
                  }
                }
                n437 = Or(x=w1167, y=w1172) -> (x .or. y?=w1174:bool)
                n438 = Select(t=State_Type_Definitions,_for_0.26g_versions_and_later_2."True Stop" ("Enum"), s=w1172, f=State_Type_Definitions,_for_0.26g_versions_and_later_2."Task 5F: ARM GRAB HEIGHT" ("Enum")) -> (s? t:f=w1169:T16)
                n439 = Select(t=w1169, s=w1174, f=State_Type_Definitions,_for_0.26g_versions_and_later_2."Task 5E: POSITION ARM" ("Enum")) -> (s? t:f=w1173:T16)
              }
              frame "Exit" {
                n440 = for {
                  shift-right: [w1196] -> w1193
                  shift-left: w1190 -> [w1197]
                  tunnel: string[] ["STOP", "RESET ENCODERS", "RESET YAW", "ARDUINO MODE 0"] -> [w1195] mode=indexing
                  n441 = Enqueue Element(queue=w1197, element=w1195) -> (queue out=w1196:refnum<queue>)  [unwired: 2 in, 2 out]
                }
              }
            }
            n442 = Bundle By Name(cluster=w1156, "yStepper desired"=w1152) -> (w1155:T18)
          }
          frame 21 {
            # ">>> Motor control cluster >>>"
            # ">>> yStepper command>>>"
            # ">> Manual override >>"
            n443 = Dequeue Element(queue=w1208, timeout in ms (-1)=w1207, error in (no error)=w1209) -> (element=w1206:T8)  [unwired: 3 out]
            n444 = Equal?(x=w1205, y=u8 1) -> (x = y?=w1203:bool)
            n445 = case shown="\"Start Task 1\", Default" w1206 {
              tunnel: [w1219 State_Type_Definitions,_for_0.26g_versions_and_later_2."True Stop" ("Enum")] -> w1210
              tunnel: [w1222 w1239] -> w1211
              tunnel: [State_Type_Definitions,_for_0.26g_versions_and_later_2."Idle" ("Enum") State_Type_Definitions,_for_0.26g_versions_and_later_2."Shutdown" ("Enum")] -> w1212
              tunnel: w1203 -> [w1218 _]
              tunnel: w1202 -> [w1217 _]
              tunnel: w1201 -> [w1213 w1236]
              frame "Start Task 1", Default {
                # "Stays in Task 5F until stepper reaches desired \nheight"
                # "T: Go back to idle, F: Continue with task\""
                # ">> Manual override >>"
                n446 = case shown="True" w1218 {
                  tunnel: [w1226 w1232] -> w1222
                  tunnel: w1213 -> [w1224 w1230]
                  frame False {
                    n447 = for {
                      tunnel: string[] ["Z STEPPER GRAB HEIGHT", "READ STEPPER VALUES"] ("element") -> [w1227] mode=indexing
                      shift-right: [w1229] -> w1226
                      shift-left: w1224 -> [w1228]
                      n448 = Enqueue Element(queue=w1228, element=w1227) -> (queue out=w1229:refnum<queue>)  [unwired: 2 in, 2 out]
                    }
                  }
                  frame True {
                    n449 = for {
                      shift-right: [w1234] -> w1232
                      shift-left: w1230 -> [w1235]
                      tunnel: string[] ["SET TIMER 5", "CLOSE CLAW", ""] -> [w1233] mode=indexing
                      n450 = Enqueue Element(queue=w1235, element=w1233) -> (queue out=w1234:refnum<queue>)  [unwired: 2 in, 2 out]
                    }
                  }
                }
                n451 = Or(x=w1218, y=w1217) -> (x .or. y?=w1220:bool)
                n452 = Select(t=State_Type_Definitions,_for_0.26g_versions_and_later_2."True Stop" ("Enum"), s=w1217, f=State_Type_Definitions,_for_0.26g_versions_and_later_2."Task 5G: CLOSE CLAW" ("Enum")) -> (s? t:f=w1214:T16)
                n453 = Select(t=w1214, s=w1220, f=State_Type_Definitions,_for_0.26g_versions_and_later_2."Task 5F: ARM GRAB HEIGHT" ("Enum")) -> (s? t:f=w1219:T16)
              }
              frame "Exit" {
                n454 = for {
                  shift-right: [w1242] -> w1239
                  shift-left: w1236 -> [w1243]
                  tunnel: string[] ["STOP", "RESET ENCODERS", "RESET YAW", "ARDUINO MODE 0"] -> [w1241] mode=indexing
                  n455 = Enqueue Element(queue=w1243, element=w1241) -> (queue out=w1242:refnum<queue>)  [unwired: 2 in, 2 out]
                }
              }
            }
          }
          frame 22 {
            # ">>> yStepper command>>>"
            # ">> Manual override >>"
            n456 = Dequeue Element(queue=w1254, timeout in ms (-1)=w1253, error in (no error)=w1252) -> (element=w1251:T8)  [unwired: 3 out]
            n457 = case shown="\"Start Task 1\", Default" w1251 {
              tunnel: [w1263 State_Type_Definitions,_for_0.26g_versions_and_later_2."True Stop" ("Enum")] -> w1256
              tunnel: [w1266 w1283] -> w1249
              tunnel: [State_Type_Definitions,_for_0.26g_versions_and_later_2."Idle" ("Enum") State_Type_Definitions,_for_0.26g_versions_and_later_2."Shutdown" ("Enum")] -> w1248
              tunnel: w1250 -> [w1257 _]
              tunnel: w1255 -> [w1262 w1280]
              tunnel: w1246 -> [w1261 _]
              frame "Start Task 1", Default {
                # ">> Is time up? >>"
                # "Determines if object is in range to pick up"
                # ">> Manual override >>"
                n458 = case shown="True" w1261 {
                  tunnel: [w1270 w1276] -> w1266
                  tunnel: w1262 -> [w1268 w1274]
                  frame False {
                    n459 = for {
                      tunnel: string[] ["CLOSE CLAW", "START TIMER"] ("element") -> [w1271] mode=indexing
                      shift-right: [w1273] -> w1270
                      shift-left: w1268 -> [w1272]
                      n460 = Enqueue Element(queue=w1272, element=w1271) -> (queue out=w1273:refnum<queue>)  [unwired: 2 in, 2 out]
                    }
                  }
                  frame True {
                    n461 = for {
                      shift-right: [w1278] -> w1276
                      shift-left: w1274 -> [w1279]
                      tunnel: string[] ["READ STEPPER VALUES", "", ""] -> [w1277] mode=indexing
                      n462 = Enqueue Element(queue=w1279, element=w1277) -> (queue out=w1278:refnum<queue>)  [unwired: 2 in, 2 out]
                    }
                  }
                }
                n463 = Or(x=w1261, y=w1257) -> (x .or. y?=w1264:bool)
                n464 = Select(t=State_Type_Definitions,_for_0.26g_versions_and_later_2."True Stop" ("Enum"), s=w1257, f=State_Type_Definitions,_for_0.26g_versions_and_later_2."Task 5H: RAISE ARM" ("Enum")) -> (s? t:f=w1259:T16)
                n465 = Select(t=w1259, s=w1264, f=State_Type_Definitions,_for_0.26g_versions_and_later_2."Task 5G: CLOSE CLAW" ("Enum")) -> (s? t:f=w1263:T16)
              }
              frame "Exit" {
                n466 = for {
                  shift-right: [w1286] -> w1283
                  shift-left: w1280 -> [w1287]
                  tunnel: string[] ["STOP", "RESET ENCODERS", "RESET YAW", "ARDUINO MODE 0"] -> [w1285] mode=indexing
                  n467 = Enqueue Element(queue=w1287, element=w1285) -> (queue out=w1286:refnum<queue>)  [unwired: 2 in, 2 out]
                }
              }
            }
          }
          frame 23 {
            # ">>> yStepper command>>>"
            # ">> Manual override >>"
            n468 = Dequeue Element(queue=w1298, timeout in ms (-1)=w1297, error in (no error)=w1299) -> (element=w1296:T8)  [unwired: 3 out]
            n469 = Equal?(x=w1295, y=u8 60) -> (x = y?=w1293:bool)
            n470 = case shown="\"Start Task 1\", Default" w1296 {
              tunnel: [w1309 State_Type_Definitions,_for_0.26g_versions_and_later_2."True Stop" ("Enum")] -> w1300
              tunnel: [w1312 w1329] -> w1301
              tunnel: [State_Type_Definitions,_for_0.26g_versions_and_later_2."Idle" ("Enum") State_Type_Definitions,_for_0.26g_versions_and_later_2."Shutdown" ("Enum")] -> w1302
              tunnel: w1293 -> [w1308 _]
              tunnel: w1292 -> [w1307 _]
              tunnel: w1291 -> [w1303 w1326]
              frame "Start Task 1", Default {
                # "Stays in Task 5_A until stepper reaches desired \nheight"
                # "T: Go back to idle, F: Continue with task\""
                # ">> Manual override >>"
                n471 = case shown="False" w1308 {
                  tunnel: [w1316 w1322] -> w1312
                  tunnel: w1303 -> [w1314 w1320]
                  frame False {
                    n472 = for {
                      tunnel: string[] ["Z STEPPER CAM HEIGHT", "READ STEPPER VALUES"] ("element") -> [w1317] mode=indexing
                      shift-right: [w1319] -> w1316
                      shift-left: w1314 -> [w1318]
                      n473 = Enqueue Element(queue=w1318, element=w1317) -> (queue out=w1319:refnum<queue>)  [unwired: 2 in, 2 out]
                    }
                  }
                  frame True {
                    n474 = for {
                      shift-right: [w1324] -> w1322
                      shift-left: w1320 -> [w1325]
                      tunnel: string[] ["ARDUINO - ULTRASONIC", "READ ULTRASONIC", ""] -> [w1323] mode=indexing
                      n475 = Enqueue Element(queue=w1325, element=w1323) -> (queue out=w1324:refnum<queue>)  [unwired: 2 in, 2 out]
                    }
                  }
                }
                n476 = Or(x=w1308, y=w1307) -> (x .or. y?=w1310:bool)
                n477 = Select(t=State_Type_Definitions,_for_0.26g_versions_and_later_2."True Stop" ("Enum"), s=w1307, f=State_Type_Definitions,_for_0.26g_versions_and_later_2."True Stop" ("Enum")) -> (s? t:f=w1304:T16)
                n478 = Select(t=w1304, s=w1310, f=State_Type_Definitions,_for_0.26g_versions_and_later_2."Task 5H: RAISE ARM" ("Enum")) -> (s? t:f=w1309:T16)
              }
              frame "Exit" {
                n479 = for {
                  shift-right: [w1332] -> w1329
                  shift-left: w1326 -> [w1333]
                  tunnel: string[] ["STOP", "RESET ENCODERS", "RESET YAW", "ARDUINO MODE 0"] -> [w1331] mode=indexing
                  n480 = Enqueue Element(queue=w1333, element=w1331) -> (queue out=w1332:refnum<queue>)  [unwired: 2 in, 2 out]
                }
              }
            }
          }
          frame 24 {
            # ">>> yStepper command>>>"
            n481 = Dequeue Element(queue=w1343, timeout in ms (-1)=w1342, error in (no error)=w1341) -> (element=w1348:T8)  [unwired: 3 out]
            n482 = Equal?(x=w1339, y=u8 60) -> (x = y?=w1338:bool)
            n483 = case shown="\"Start Task 1\", Default" w1348 {
              tunnel: [w1355 State_Type_Definitions,_for_0.26g_versions_and_later_2."True Stop" ("Enum")] -> w1346
              tunnel: [w1354 w1372] -> w1345
              tunnel: [State_Type_Definitions,_for_0.26g_versions_and_later_2."Idle" ("Enum") State_Type_Definitions,_for_0.26g_versions_and_later_2."Shutdown" ("Enum")] -> w1347
              tunnel: w1344 -> [w1350 _]
              tunnel: w1340 -> [w1352 _]
              tunnel: w1338 -> [w1349 _]
              frame "Start Task 1", Default {
                n484 = case shown="False" w1349 {
                  tunnel: [w1360 w1366] -> w1354
                  tunnel: w1352 -> [w1358 w1364]
                  frame False {
                    n485 = for {
                      tunnel: string[] ["Z STEPPER CAM HEIGHT", "READ STEPPER VALUES"] ("element") -> [w1361] mode=indexing
                      shift-right: [w1363] -> w1360
                      shift-left: w1358 -> [w1362]
                      n486 = Enqueue Element(queue=w1362, element=w1361) -> (queue out=w1363:refnum<queue>)  [unwired: 2 in, 2 out]
                    }
                  }
                  frame True {
                    n487 = for {
                      shift-right: [w1368] -> w1366
                      shift-left: w1364 -> [w1369]
                      tunnel: string[] ["CAM ACQ", "OPEN LOG CAM"] -> [w1367] mode=indexing
                      n488 = Enqueue Element(queue=w1369, element=w1367) -> (queue out=w1368:refnum<queue>)  [unwired: 2 in, 2 out]
                    }
                  }
                }
                n489 = Or(x=w1349, y=w1350) -> (x .or. y?=w1351:bool)
                n490 = Select(t=State_Type_Definitions,_for_0.26g_versions_and_later_2."Task 6_B" ("Enum"), s=w1351, f=State_Type_Definitions,_for_0.26g_versions_and_later_2."Task 6_A" ("Enum")) -> (s? t:f=w1355:T16)
              }
              frame "Exit" {
                n491 = for {
                  shift-right: [w1375] -> w1372
                  shift-left: _ -> [w1376]
                  tunnel: string[] ["STOP", "RESET ENCODERS", "RESET YAW", "ARDUINO MODE 0"] -> [w1374] mode=indexing
                  n492 = Enqueue Element(queue=w1376, element=w1374) -> (queue out=w1375:refnum<queue>)  [unwired: 2 in, 2 out]
                }
              }
            }
          }
          frame 25 {
            # ">>> yStepper command>>>"
            n493 = Dequeue Element(queue=w1388, timeout in ms (-1)=w1386, error in (no error)=w1387) -> (element=w1385:T8)  [unwired: 3 out]
            n494 = case shown="\"Start Task 1\", Default" w1385 {
              tunnel: [w1395 State_Type_Definitions,_for_0.26g_versions_and_later_2."True Stop" ("Enum")] -> w1381
              tunnel: [w1394 w1413] -> w1389
              tunnel: [State_Type_Definitions,_for_0.26g_versions_and_later_2."Idle" ("Enum") State_Type_Definitions,_for_0.26g_versions_and_later_2."Shutdown" ("Enum")] -> w1382
              tunnel: w1384 -> [w1390 _]
              tunnel: w1383 -> [w1392 _]
              tunnel: w1380 -> [w1391 w1410]
              frame "Start Task 1", Default {
                # ">> Manual override >>"
                n495 = case shown="False" w1392 {
                  tunnel: [w1400 w1406] -> w1394
                  tunnel: w1391 -> [w1399 w1404]
                  frame False {
                    n496 = for {
                      shift-right: [w1403] -> w1400
                      shift-left: w1399 -> [w1402]
                      tunnel: string[] ["CAM ACQ", "PROCESS IMAGE", "OPEN CLAW"] -> [w1401] mode=indexing
                      n497 = Enqueue Element(queue=w1402, element=w1401) -> (queue out=w1403:refnum<queue>)  [unwired: 2 in, 2 out]
                    }
                  }
                  frame True {
                    n498 = for {
                      shift-right: [w1408] -> w1406
                      shift-left: w1404 -> [w1409]
                      tunnel: string[] ["CAM ACQ", "PROCESS IMAGE", "CLOSE CLAW"] -> [w1407] mode=indexing
                      n499 = Enqueue Element(queue=w1409, element=w1407) -> (queue out=w1408:refnum<queue>)  [unwired: 2 in, 2 out]
                    }
                  }
                }
                n500 = Select(t=State_Type_Definitions,_for_0.26g_versions_and_later_2."True Stop" ("Enum"), s=w1390, f=State_Type_Definitions,_for_0.26g_versions_and_later_2."Task 6_B" ("Enum")) -> (s? t:f=w1395:T16)
              }
              frame "Exit" {
                # ">> State after true stop >>"
                # ">> Goes to true stop >>"
                n501 = for {
                  shift-right: [w1416] -> w1413
                  shift-left: w1410 -> [w1417]
                  tunnel: string[] ["STOP", "RESET ENCODERS", "RESET YAW", ""] -> [w1415] mode=indexing
                  n502 = Enqueue Element(queue=w1417, element=w1415) -> (queue out=w1416:refnum<queue>)  [unwired: 2 in, 2 out]
                }
              }
            }
          }
          frame 26 {
          }
          frame 27 {
            # ">>> Motor control cluster >>>"
            # ">>> yStepper command>>>"
            # ">> Manual override >>"
            n503 = Dequeue Element(queue=w1434, timeout in ms (-1)=w1433, error in (no error)=w1435) -> (element=w1432:T8)  [unwired: 3 out]
            n504 = Equal?(x=w1431, y=u8 60) -> (x = y?=w1429:bool)
            n505 = case shown="\"Start Task 1\", Default" w1432 {
              tunnel: [w1445 State_Type_Definitions,_for_0.26g_versions_and_later_2."True Stop" ("Enum")] -> w1436
              tunnel: [w1448 w1465] -> w1437
              tunnel: [State_Type_Definitions,_for_0.26g_versions_and_later_2."Idle" ("Enum") State_Type_Definitions,_for_0.26g_versions_and_later_2."Shutdown" ("Enum")] -> w1438
              tunnel: w1429 -> [w1444 _]
              tunnel: w1428 -> [w1443 _]
              tunnel: w1427 -> [w1439 w1462]
              frame "Start Task 1", Default {
                # "Stays in Task 5_A until stepper reaches desired \nheight"
                # "T: Go back to idle, F: Continue with task\""
                # ">> Manual override >>"
                n506 = case shown="False" w1444 {
                  tunnel: [w1452 w1458] -> w1448
                  tunnel: w1439 -> [w1450 w1456]
                  frame False {
                    n507 = for {
                      tunnel: string[] ["Z STEPPER CAM HEIGHT", "READ STEPPER VALUES"] ("element") -> [w1453] mode=indexing
                      shift-right: [w1455] -> w1452
                      shift-left: w1450 -> [w1454]
                      n508 = Enqueue Element(queue=w1454, element=w1453) -> (queue out=w1455:refnum<queue>)  [unwired: 2 in, 2 out]
                    }
                  }
                  frame True {
                    n509 = for {
                      shift-right: [w1460] -> w1458
                      shift-left: w1456 -> [w1461]
                      tunnel: string[] ["ARDUINO - ULTRASONIC", "READ ULTRASONIC", ""] -> [w1459] mode=indexing
                      n510 = Enqueue Element(queue=w1461, element=w1459) -> (queue out=w1460:refnum<queue>)  [unwired: 2 in, 2 out]
                    }
                  }
                }
                n511 = Or(x=w1444, y=w1443) -> (x .or. y?=w1446:bool)
                n512 = Select(t=State_Type_Definitions,_for_0.26g_versions_and_later_2."True Stop" ("Enum"), s=w1443, f=State_Type_Definitions,_for_0.26g_versions_and_later_2."Task 8B: MOVE TO BOX" ("Enum")) -> (s? t:f=w1440:T16)
                n513 = Select(t=w1440, s=w1446, f=State_Type_Definitions,_for_0.26g_versions_and_later_2."Task 8A: RAISE ARM" ("Enum")) -> (s? t:f=w1445:T16)
              }
              frame "Exit" {
                n514 = for {
                  shift-right: [w1468] -> w1465
                  shift-left: w1462 -> [w1469]
                  tunnel: string[] ["STOP", "RESET ENCODERS", "RESET YAW", "ARDUINO MODE 0"] -> [w1467] mode=indexing
                  n515 = Enqueue Element(queue=w1469, element=w1467) -> (queue out=w1468:refnum<queue>)  [unwired: 2 in, 2 out]
                }
              }
            }
          }
          frame 28 {
            w1477 = u8 15 ("y")
            # ">>> yStepper command>>>"
            n516 = Less?(x=w1474, y=w1477) -> (x < y?=w1475:bool)
            n517 = Dequeue Element(queue=w1481, timeout in ms (-1)=w1480, error in (no error)=w1482) -> (element=w1479:T8)  [unwired: 3 out]
            n518 = Less?(x=w1473, y=w1477) -> (x < y?=w1476:bool)
            n519 = And(x=w1476, y=w1475) -> (x .and. y?=w1472:bool)
            n520 = case shown="\"Start Task 1\", Default" w1479 {
              tunnel: [w1494 State_Type_Definitions,_for_0.26g_versions_and_later_2."True Stop" ("Enum")] -> w1484
              tunnel: [w1497 w1514] -> w1483
              tunnel: [State_Type_Definitions,_for_0.26g_versions_and_later_2."Idle" ("Enum") State_Type_Definitions,_for_0.26g_versions_and_later_2."Shutdown" ("Enum")] -> w1485
              tunnel: w1487 -> [w1493 _]
              tunnel: w1486 -> [w1489 w1511]
              tunnel: w1472 -> [w1488 _]
              frame "Start Task 1", Default {
                # "Stays in Task 5_B to capture image over 5 seconds"
                # "T: Go back to idle, F: Continue with task\""
                # ">> Manual override >>"
                n521 = case shown="True" w1488 {
                  tunnel: [w1501 w1507] -> w1497
                  tunnel: w1489 -> [w1499 w1505]
                  frame False {
                    n522 = for {
                      tunnel: string[] ["FORWARD", "READ ULTRASONIC", "READ NAVX"] ("element") -> [w1502] mode=indexing
                      shift-right: [w1504] -> w1501
                      shift-left: w1499 -> [w1503]
                      n523 = Enqueue Element(queue=w1503, element=w1502) -> (queue out=w1504:refnum<queue>)  [unwired: 2 in, 2 out]
                    }
                  }
                  frame True {
                    n524 = for {
                      shift-right: [w1509] -> w1507
                      shift-left: w1505 -> [w1510]
                      tunnel: string[] ["STOP", "RESET ENCODERS", "OPEN LOG CAM", "SET TIMER 2", "OPEN IMAQ REF"] -> [w1508] mode=indexing
                      n525 = Enqueue Element(queue=w1510, element=w1508) -> (queue out=w1509:refnum<queue>)  [unwired: 2 in, 2 out]
                    }
                  }
                }
                n526 = Or(x=w1488, y=w1493) -> (x .or. y?=w1495:bool)
                n527 = Select(t=State_Type_Definitions,_for_0.26g_versions_and_later_2."True Stop" ("Enum"), s=w1493, f=State_Type_Definitions,_for_0.26g_versions_and_later_2."Task 8C: CAM BURST" ("Enum")) -> (s? t:f=w1490:T16)
                n528 = Select(t=w1490, s=w1495, f=State_Type_Definitions,_for_0.26g_versions_and_later_2."Task 8B: MOVE TO BOX" ("Enum")) -> (s? t:f=w1494:T16)
              }
              frame "Exit" {
                n529 = for {
                  shift-right: [w1517] -> w1514
                  shift-left: w1511 -> [w1518]
                  tunnel: string[] ["STOP", "RESET ENCODERS", "RESET YAW", "ARDUINO MODE 0"] -> [w1516] mode=indexing
                  n530 = Enqueue Element(queue=w1518, element=w1516) -> (queue out=w1517:refnum<queue>)  [unwired: 2 in, 2 out]
                }
              }
            }
          }
          frame 29 {
            # ">>> Motor control cluster >>>"
            # ">>> yStepper command>>>"
            # ">> Manual override >>"
            n531 = Dequeue Element(queue=w1529, timeout in ms (-1)=w1528, error in (no error)=w1527) -> (element=w1526:T8)  [unwired: 3 out]
            n532 = case shown="\"Start Task 1\", Default" w1526 {
              tunnel: [w1538 State_Type_Definitions,_for_0.26g_versions_and_later_2."True Stop" ("Enum")] -> w1531
              tunnel: [w1541 w1558] -> w1524
              tunnel: [State_Type_Definitions,_for_0.26g_versions_and_later_2."Idle" ("Enum") State_Type_Definitions,_for_0.26g_versions_and_later_2."Shutdown" ("Enum")] -> w1523
              tunnel: w1525 -> [w1532 _]
              tunnel: w1530 -> [w1537 w1555]
              tunnel: w1521 -> [w1536 _]
              frame "Start Task 1", Default {
                # ">> Is time up? >>"
                # "Determines if object is in range to pick up"
                # ">> Manual override >>"
                n533 = case shown="True" w1536 {
                  tunnel: [w1545 w1551] -> w1541
                  tunnel: w1537 -> [w1543 w1549]
                  frame False {
                    n534 = for {
                      tunnel: string[] ["CAM ACQ", "START TIMER"] ("element") -> [w1546] mode=indexing
                      shift-right: [w1548] -> w1545
                      shift-left: w1543 -> [w1547]
                      n535 = Enqueue Element(queue=w1547, element=w1546) -> (queue out=w1548:refnum<queue>)  [unwired: 2 in, 2 out]
                    }
                  }
                  frame True {
                    n536 = for {
                      shift-right: [w1553] -> w1551
                      shift-left: w1549 -> [w1554]
                      tunnel: string[] ["CAM CLOSE", "PROCESS IMAGE", "SET TIMER 5"] -> [w1552] mode=indexing
                      n537 = Enqueue Element(queue=w1554, element=w1552) -> (queue out=w1553:refnum<queue>)  [unwired: 2 in, 2 out]
                    }
                  }
                }
                n538 = Or(x=w1536, y=w1532) -> (x .or. y?=w1539:bool)
                n539 = Select(t=State_Type_Definitions,_for_0.26g_versions_and_later_2."True Stop" ("Enum"), s=w1532, f=State_Type_Definitions,_for_0.26g_versions_and_later_2."Task 8D: PROCESS IMAGE" ("Enum")) -> (s? t:f=w1534:T16)
                n540 = Select(t=w1534, s=w1539, f=State_Type_Definitions,_for_0.26g_versions_and_later_2."Task 8C: CAM BURST" ("Enum")) -> (s? t:f=w1538:T16)
              }
              frame "Exit" {
                n541 = for {
                  shift-right: [w1561] -> w1558
                  shift-left: w1555 -> [w1562]
                  tunnel: string[] ["STOP", "RESET ENCODERS", "RESET YAW", "ARDUINO MODE 0"] -> [w1560] mode=indexing
                  n542 = Enqueue Element(queue=w1562, element=w1560) -> (queue out=w1561:refnum<queue>)  [unwired: 2 in, 2 out]
                }
              }
            }
          }
          frame 30 {
            # ">>> yStepper command>>>"
            n543 = Dequeue Element(queue=w1570, timeout in ms (-1)=w1569, error in (no error)=w1568) -> (element=w1567:T8)  [unwired: 3 out]
            n544 = case shown="\"Start Task 1\", Default" w1567 {
              tunnel: [w1582 State_Type_Definitions,_for_0.26g_versions_and_later_2."True Stop" ("Enum")] -> w1574
              tunnel: [w1585 w1602] -> w1573
              tunnel: [State_Type_Definitions,_for_0.26g_versions_and_later_2."Idle" ("Enum") State_Type_Definitions,_for_0.26g_versions_and_later_2."Shutdown" ("Enum")] -> w1575
              tunnel: w1571 -> [w1581 _]
              tunnel: w1572 -> [w1577 w1599]
              tunnel: w1565 -> [w1576 _]
              frame "Start Task 1", Default {
                # ">> T: Breaks out of state loop; F: Stays in loop>>"
                # ">> Manual override >>"
                # ">> Checks if time is up>>"
                # "Stays in Task 5D until the object is detected"
                # "T: Go back to idle, F: Continue with task\""
                # ">> Manual override >>"
                n545 = case shown="True" w1576 {
                  tunnel: [w1589 w1595] -> w1585
                  tunnel: w1577 -> [w1587 w1593]
                  frame False {
                    n546 = for {
                      tunnel: string[] ["START TIMER", "PROCESS IMAGE", ""] ("element") -> [w1590] mode=indexing
                      shift-right: [w1592] -> w1589
                      shift-left: w1587 -> [w1591]
                      n547 = Enqueue Element(queue=w1591, element=w1590) -> (queue out=w1592:refnum<queue>)  [unwired: 2 in, 2 out]
                    }
                  }
                  frame True {
                    n548 = for {
                      shift-right: [w1597] -> w1595
                      shift-left: w1593 -> [w1598]
                      tunnel: string[] ["RESET ENCODERS", "", ""] -> [w1596] mode=indexing
                      n549 = Enqueue Element(queue=w1598, element=w1596) -> (queue out=w1597:refnum<queue>)  [unwired: 2 in, 2 out]
                    }
                  }
                }
                n550 = Or(x=w1576, y=w1581) -> (x .or. y?=w1583:bool)
                n551 = Select(t=State_Type_Definitions,_for_0.26g_versions_and_later_2."True Stop" ("Enum"), s=w1581, f=State_Type_Definitions,_for_0.26g_versions_and_later_2."Task 8E: ROBOT ADJUST" ("Enum")) -> (s? t:f=w1578:T16)
                n552 = Select(t=w1578, s=w1583, f=State_Type_Definitions,_for_0.26g_versions_and_later_2."Task 8D: PROCESS IMAGE" ("Enum")) -> (s? t:f=w1582:T16)
              }
              frame "Exit" {
                n553 = for {
                  shift-right: [w1605] -> w1602
                  shift-left: w1599 -> [w1606]
                  tunnel: string[] ["STOP", "RESET ENCODERS", "RESET YAW", "ARDUINO MODE 0"] -> [w1604] mode=indexing
                  n554 = Enqueue Element(queue=w1606, element=w1604) -> (queue out=w1605:refnum<queue>)  [unwired: 2 in, 2 out]
                }
              }
            }
          }
          frame 31 {
            # ">>> Motor control cluster >>>"
            # ">>> yStepper command>>>"
            n555 = Dequeue Element(queue=w1623, timeout in ms (-1)=w1622, error in (no error)=w1621) -> (element=w1620:T8)  [unwired: 3 out]
            n556 = Subtract(x=w1618, y=300.0) -> (x-y=w1616:dbl)
            "x-y" <- w1616
            n557 = formula code="if (error <= -61&&error > -300){\ndistance = -15;\nxSpeed = -30;\n}\n\nelse if (error <= -51 && error >= -60){\ndistance = -10;\nxSpeed = -30;\n}\n\nelse if (error >= -50 && error <= 50){\ndistance = 0;\nxSpeed = 0;\n}\n\nelse if (error >= 51 && error <= 80){\ndistance = 10;\nxSpeed = 30;\n}\n\nelse if (error >= 81 && error <= 100){\ndistance = 15;\nxSpeed = 30;\n}\n\nelse if (error >= 101 && error <= 120){\ndistance = 20;\nxSpeed = 30;\n}\n\nelse if (error >= 121 && error < 300){\ndistance = 25;\nxSpeed = 30;\n}\n\nelse{\ndistance = 0;\nxSpeed = 0;\n}"("error"=w1616) -> ("distance"=w1611:dbl, "xSpeed"=w1613:dbl)
            n558 = formula code="if (target > 0){\nif (current  >= target)\noutput = 1;\n\nelse if (current != target)\noutput = 0;\n}\n\nelse if (target == 0){\nif (current == target)\noutput = 1;\n\nelse if (current != target)\noutput = 0;\n}\n\nelse if (target < 0){\nif (current <= target)\noutput = 1;\n\nelse if (current != target)\noutput = 0;\n}\n\nelse if (current != target)\noutput = 0;"("target"=w1611, "current"=w1612) -> ("output"=w1610:dbl)
            n559 = Bundle By Name(cluster=w1615, "xSpeed"=w1613) -> (w1614:T17)
            n560 = Equal?(x=w1610, y=1.0) -> (x = y?=w1608:bool)
            n561 = case shown="\"Start Task 1\", Default" w1620 {
              tunnel: [w1635 State_Type_Definitions,_for_0.26g_versions_and_later_2."True Stop" ("Enum")] -> w1627
              tunnel: [w1638 w1655] -> w1626
              tunnel: [State_Type_Definitions,_for_0.26g_versions_and_later_2."Idle" ("Enum") State_Type_Definitions,_for_0.26g_versions_and_later_2."Shutdown" ("Enum")] -> w1628
              tunnel: w1624 -> [w1634 _]
              tunnel: w1625 -> [w1630 w1652]
              tunnel: w1608 -> [w1629 _]
              frame "Start Task 1", Default {
                # ">> T: Breaks out of state loop; F: Stays in loop>>"
                # ">> Manual override >>"
                # ">> Checks if time is up>>"
                # "Stays in Task 5D until the object is detected"
                # "T: Go back to idle, F: Continue with task\""
                # ">> Manual override >>"
                n562 = case shown="True" w1629 {
                  tunnel: [w1642 w1648] -> w1638
                  tunnel: w1630 -> [w1640 w1646]
                  frame False {
                    n563 = for {
                      tunnel: string[] ["X AXIS - SLOW", "READ ENCODERS", "READ NAVX"] ("element") -> [w1643] mode=indexing
                      shift-right: [w1645] -> w1642
                      shift-left: w1640 -> [w1644]
                      n564 = Enqueue Element(queue=w1644, element=w1643) -> (queue out=w1645:refnum<queue>)  [unwired: 2 in, 2 out]
                    }
                  }
                  frame True {
                    n565 = for {
                      shift-right: [w1650] -> w1648
                      shift-left: w1646 -> [w1651]
                      tunnel: string[] ["SET TIMER 2", "STOP", "READ STEPPER VALUES", ""] -> [w1649] mode=indexing
                      n566 = Enqueue Element(queue=w1651, element=w1649) -> (queue out=w1650:refnum<queue>)  [unwired: 2 in, 2 out]
                    }
                  }
                }
                n567 = Or(x=w1629, y=w1634) -> (x .or. y?=w1636:bool)
                n568 = Select(t=State_Type_Definitions,_for_0.26g_versions_and_later_2."True Stop" ("Enum"), s=w1634, f=State_Type_Definitions,_for_0.26g_versions_and_later_2."Task 8H: ARM ADJUST" ("Enum")) -> (s? t:f=w1631:T16)
                n569 = Select(t=w1631, s=w1636, f=State_Type_Definitions,_for_0.26g_versions_and_later_2."Task 8E: ROBOT ADJUST" ("Enum")) -> (s? t:f=w1635:T16)
              }
              frame "Exit" {
                n570 = for {
                  shift-right: [w1658] -> w1655
                  shift-left: w1652 -> [w1659]
                  tunnel: string[] ["STOP", "RESET ENCODERS", "RESET YAW", "ARDUINO MODE 0"] -> [w1657] mode=indexing
                  n571 = Enqueue Element(queue=w1659, element=w1657) -> (queue out=w1658:refnum<queue>)  [unwired: 2 in, 2 out]
                }
              }
            }
          }
          frame 32 {
            # ">>> Motor control cluster >>>"
            # ">>> yStepper command>>>"
            # ">> Manual override >>"
            n572 = Dequeue Element(queue=w1670, timeout in ms (-1)=w1669, error in (no error)=w1668) -> (element=w1667:T8)  [unwired: 3 out]
            n573 = case shown="\"Start Task 1\", Default" w1667 {
              tunnel: [w1679 State_Type_Definitions,_for_0.26g_versions_and_later_2."True Stop" ("Enum")] -> w1672
              tunnel: [w1682 w1699] -> w1665
              tunnel: [State_Type_Definitions,_for_0.26g_versions_and_later_2."Idle" ("Enum") State_Type_Definitions,_for_0.26g_versions_and_later_2."Shutdown" ("Enum")] -> w1664
              tunnel: w1666 -> [w1673 _]
              tunnel: w1671 -> [w1678 w1696]
              tunnel: w1662 -> [w1677 _]
              frame "Start Task 1", Default {
                # ">> Is time up? >>"
                # "Determines if object is in range to pick up"
                # ">> Manual override >>"
                n574 = case shown="False" w1677 {
                  tunnel: [w1686 w1692] -> w1682
                  tunnel: w1678 -> [w1684 w1690]
                  frame False {
                    n575 = for {
                      tunnel: string[] ["CAM ACQ", "START TIMER"] ("element") -> [w1687] mode=indexing
                      shift-right: [w1689] -> w1686
                      shift-left: w1684 -> [w1688]
                      n576 = Enqueue Element(queue=w1688, element=w1687) -> (queue out=w1689:refnum<queue>)  [unwired: 2 in, 2 out]
                    }
                  }
                  frame True {
                    n577 = for {
                      shift-right: [w1694] -> w1692
                      shift-left: w1690 -> [w1695]
                      tunnel: string[] ["CAM CLOSE", "PROCESS IMAGE", "SET TIMER 3"] -> [w1693] mode=indexing
                      n578 = Enqueue Element(queue=w1695, element=w1693) -> (queue out=w1694:refnum<queue>)  [unwired: 2 in, 2 out]
                    }
                  }
                }
                n579 = Or(x=w1677, y=w1673) -> (x .or. y?=w1680:bool)
                n580 = Select(t=State_Type_Definitions,_for_0.26g_versions_and_later_2."True Stop" ("Enum"), s=w1673, f=State_Type_Definitions,_for_0.26g_versions_and_later_2."Task 8G: PROCESS IMAGE 2" ("Enum")) -> (s? t:f=w1675:T16)
                n581 = Select(t=w1675, s=w1680, f=State_Type_Definitions,_for_0.26g_versions_and_later_2."Task 8F: CAM BURST 2" ("Enum")) -> (s? t:f=w1679:T16)
              }
              frame "Exit" {
                n582 = for {
                  shift-right: [w1702] -> w1699
                  shift-left: w1696 -> [w1703]
                  tunnel: string[] ["STOP", "RESET ENCODERS", "RESET YAW", "ARDUINO MODE 0"] -> [w1701] mode=indexing
                  n583 = Enqueue Element(queue=w1703, element=w1701) -> (queue out=w1702:refnum<queue>)  [unwired: 2 in, 2 out]
                }
              }
            }
          }
          frame 33 {
            # ">>> yStepper command>>>"
            n584 = Dequeue Element(queue=w1711, timeout in ms (-1)=w1710, error in (no error)=w1709) -> (element=w1708:T8)  [unwired: 3 out]
            n585 = case shown="\"Start Task 1\", Default" w1708 {
              tunnel: [w1723 State_Type_Definitions,_for_0.26g_versions_and_later_2."True Stop" ("Enum")] -> w1715
              tunnel: [w1726 w1743] -> w1714
              tunnel: [State_Type_Definitions,_for_0.26g_versions_and_later_2."Idle" ("Enum") State_Type_Definitions,_for_0.26g_versions_and_later_2."Shutdown" ("Enum")] -> w1716
              tunnel: w1712 -> [w1722 _]
              tunnel: w1713 -> [w1718 w1740]
              tunnel: w1706 -> [w1717 _]
              frame "Start Task 1", Default {
                # ">> T: Breaks out of state loop; F: Stays in loop>>"
                # ">> Manual override >>"
                # ">> Checks if time is up>>"
                # "Stays in Task 5D until the object is detected"
                # "T: Go back to idle, F: Continue with task\""
                # ">> Manual override >>"
                n586 = case shown="False" w1717 {
                  tunnel: [w1730 w1736] -> w1726
                  tunnel: w1718 -> [w1728 w1734]
                  frame False {
                    n587 = for {
                      tunnel: string[] ["START TIMER", "PROCESS IMAGE", ""] ("element") -> [w1731] mode=indexing
                      shift-right: [w1733] -> w1730
                      shift-left: w1728 -> [w1732]
                      n588 = Enqueue Element(queue=w1732, element=w1731) -> (queue out=w1733:refnum<queue>)  [unwired: 2 in, 2 out]
                    }
                  }
                  frame True {
                    n589 = for {
                      shift-right: [w1738] -> w1736
                      shift-left: w1734 -> [w1739]
                      tunnel: string[] ["READ STEPPER VALUES", "Y STEPPER CONTROL", ""] -> [w1737] mode=indexing
                      n590 = Enqueue Element(queue=w1739, element=w1737) -> (queue out=w1738:refnum<queue>)  [unwired: 2 in, 2 out]
                    }
                  }
                }
                n591 = Or(x=w1717, y=w1722) -> (x .or. y?=w1724:bool)
                n592 = Select(t=State_Type_Definitions,_for_0.26g_versions_and_later_2."True Stop" ("Enum"), s=w1722, f=State_Type_Definitions,_for_0.26g_versions_and_later_2."Task 8H: ARM ADJUST" ("Enum")) -> (s? t:f=w1719:T16)
                n593 = Select(t=w1719, s=w1724, f=State_Type_Definitions,_for_0.26g_versions_and_later_2."Task 8G: PROCESS IMAGE 2" ("Enum")) -> (s? t:f=w1723:T16)
              }
              frame "Exit" {
                n594 = for {
                  shift-right: [w1746] -> w1743
                  shift-left: w1740 -> [w1747]
                  tunnel: string[] ["STOP", "RESET ENCODERS", "RESET YAW", "ARDUINO MODE 0"] -> [w1745] mode=indexing
                  n595 = Enqueue Element(queue=w1747, element=w1745) -> (queue out=w1746:refnum<queue>)  [unwired: 2 in, 2 out]
                }
              }
            }
          }
          frame 34 {
            # ">>> yStepper command>>>"
            n596 = Dequeue Element(queue=w1761, timeout in ms (-1)=w1762, error in (no error)=w1763) -> (element=w1765:T8)  [unwired: 3 out]
            n597 = formula code="if (pos < 70)\ny = 43;\n\nelse if (pos >= 71 &&pos <= 80)\ny = 40;\n\nelse if (pos >= 81 && pos <= 90)\ny = 38;\n\nelse if (pos >= 91 &&pos <= 120)\ny = 35;\n\nelse if (pos >= 121 && pos <= 140)\ny = 30;\n\nelse if (pos >= 141 && pos <= 170)\ny = 26;\n\nelse if (pos >= 171 &&pos <= 220) \ny = 20;\n\nelse if (pos >= 221&& pos <= 240)\ny = 15;\n\nelse if (pos >= 241 && pos <= 250)\ny = 10;\n\nelse if (pos >= 251)\ny = 0;"("pos"=w1753) -> ("y"=w1756:dbl)
            n598 = To Unsigned Byte Integer(number=w1756) -> (unsigned 8bit integer=w1751:u8)
            "Correcte stepper" <- w1751
            n599 = Equal?(x=w1752, y=w1751) -> (x = y?=w1750:bool)
            n600 = case shown="\"Start Task 1\", Default" w1765 {
              tunnel: [w1772 State_Type_Definitions,_for_0.26g_versions_and_later_2."True Stop" ("Enum")] -> w1759
              tunnel: [w1775 w1792] -> w1757
              tunnel: [State_Type_Definitions,_for_0.26g_versions_and_later_2."Idle" ("Enum") State_Type_Definitions,_for_0.26g_versions_and_later_2."Shutdown" ("Enum")] -> w1758
              tunnel: w1764 -> [w1771 _]
              tunnel: w1760 -> [w1767 w1789]
              tunnel: w1750 -> [w1766 _]
              frame "Start Task 1", Default {
                # ">> T: Breaks out of state loop; F: Stays in loop>>"
                # ">> Manual override >>"
                # ">> Checks if time is up>>"
                # "Stays in Task 5D until the object is detected"
                # "T: Go back to idle, F: Continue with task\""
                # ">> Manual override >>"
                n601 = case shown="False" w1766 {
                  tunnel: [w1779 w1785] -> w1775
                  tunnel: w1767 -> [w1777 w1783]
                  frame False {
                    n602 = for {
                      tunnel: string[] ["READ STEPPER VALUES", "Y STEPPER CONTROL", ""] ("element") -> [w1780] mode=indexing
                      shift-right: [w1782] -> w1779
                      shift-left: w1777 -> [w1781]
                      n603 = Enqueue Element(queue=w1781, element=w1780) -> (queue out=w1782:refnum<queue>)  [unwired: 2 in, 2 out]
                    }
                  }
                  frame True {
                    n604 = for {
                      shift-right: [w1787] -> w1785
                      shift-left: w1783 -> [w1788]
                      tunnel: string[] ["DISPOSE BUFFERS", "READ STEPPER VALUES", ""] -> [w1786] mode=indexing
                      n605 = Enqueue Element(queue=w1788, element=w1786) -> (queue out=w1787:refnum<queue>)  [unwired: 2 in, 2 out]
                    }
                  }
                }
                n606 = Or(x=w1766, y=w1771) -> (x .or. y?=w1773:bool)
                n607 = Select(t=State_Type_Definitions,_for_0.26g_versions_and_later_2."True Stop" ("Enum"), s=w1771, f=State_Type_Definitions,_for_0.26g_versions_and_later_2."Task 8I: ARM GRAB HEIGHT" ("Enum")) -> (s? t:f=w1768:T16)
                n608 = Select(t=w1768, s=w1773, f=State_Type_Definitions,_for_0.26g_versions_and_later_2."Task 8H: ARM ADJUST" ("Enum")) -> (s? t:f=w1772:T16)
              }
              frame "Exit" {
                n609 = for {
                  shift-right: [w1795] -> w1792
                  shift-left: w1789 -> [w1796]
                  tunnel: string[] ["STOP", "RESET ENCODERS", "RESET YAW", "ARDUINO MODE 0"] -> [w1794] mode=indexing
                  n610 = Enqueue Element(queue=w1796, element=w1794) -> (queue out=w1795:refnum<queue>)  [unwired: 2 in, 2 out]
                }
              }
            }
            n611 = Bundle By Name(cluster=w1755, "yStepper desired"=w1751) -> (w1754:T18)
          }
          frame 35 {
            # ">>> Motor control cluster >>>"
            # ">>> yStepper command>>>"
            # ">> Manual override >>"
            n612 = Dequeue Element(queue=w1807, timeout in ms (-1)=w1806, error in (no error)=w1808) -> (element=w1805:T8)  [unwired: 3 out]
            n613 = Equal?(x=w1804, y=u8 1) -> (x = y?=w1802:bool)
            n614 = case shown="\"Start Task 1\", Default" w1805 {
              tunnel: [w1818 State_Type_Definitions,_for_0.26g_versions_and_later_2."True Stop" ("Enum")] -> w1809
              tunnel: [w1821 w1838] -> w1810
              tunnel: [State_Type_Definitions,_for_0.26g_versions_and_later_2."Idle" ("Enum") State_Type_Definitions,_for_0.26g_versions_and_later_2."Shutdown" ("Enum")] -> w1811
              tunnel: w1802 -> [w1817 _]
              tunnel: w1801 -> [w1816 _]
              tunnel: w1800 -> [w1812 w1835]
              frame "Start Task 1", Default {
                # "Stays in Task 5F until stepper reaches desired \nheight"
                # "T: Go back to idle, F: Continue with task\""
                # ">> Manual override >>"
                n615 = case shown="True" w1817 {
                  tunnel: [w1825 w1831] -> w1821
                  tunnel: w1812 -> [w1823 w1829]
                  frame False {
                    n616 = for {
                      tunnel: string[] ["Z STEPPER GRAB HEIGHT", "READ STEPPER VALUES"] ("element") -> [w1826] mode=indexing
                      shift-right: [w1828] -> w1825
                      shift-left: w1823 -> [w1827]
                      n617 = Enqueue Element(queue=w1827, element=w1826) -> (queue out=w1828:refnum<queue>)  [unwired: 2 in, 2 out]
                    }
                  }
                  frame True {
                    n618 = for {
                      shift-right: [w1833] -> w1831
                      shift-left: w1829 -> [w1834]
                      tunnel: string[] ["SET TIMER 2", "CLOSE CLAW", ""] -> [w1832] mode=indexing
                      n619 = Enqueue Element(queue=w1834, element=w1832) -> (queue out=w1833:refnum<queue>)  [unwired: 2 in, 2 out]
                    }
                  }
                }
                n620 = Or(x=w1817, y=w1816) -> (x .or. y?=w1819:bool)
                n621 = Select(t=State_Type_Definitions,_for_0.26g_versions_and_later_2."True Stop" ("Enum"), s=w1816, f=State_Type_Definitions,_for_0.26g_versions_and_later_2."Task 8J: CLOSE CLAW" ("Enum")) -> (s? t:f=w1813:T16)
                n622 = Select(t=w1813, s=w1819, f=State_Type_Definitions,_for_0.26g_versions_and_later_2."Task 8I: ARM GRAB HEIGHT" ("Enum")) -> (s? t:f=w1818:T16)
              }
              frame "Exit" {
                n623 = for {
                  shift-right: [w1841] -> w1838
                  shift-left: w1835 -> [w1842]
                  tunnel: string[] ["STOP", "RESET ENCODERS", "RESET YAW", "ARDUINO MODE 0"] -> [w1840] mode=indexing
                  n624 = Enqueue Element(queue=w1842, element=w1840) -> (queue out=w1841:refnum<queue>)  [unwired: 2 in, 2 out]
                }
              }
            }
          }
          frame 36 {
            # ">>> yStepper command>>>"
            # ">> Manual override >>"
            n625 = Dequeue Element(queue=w1853, timeout in ms (-1)=w1852, error in (no error)=w1851) -> (element=w1850:T8)  [unwired: 3 out]
            n626 = case shown="\"Start Task 1\", Default" w1850 {
              tunnel: [w1862 State_Type_Definitions,_for_0.26g_versions_and_later_2."True Stop" ("Enum")] -> w1855
              tunnel: [w1865 w1882] -> w1848
              tunnel: [State_Type_Definitions,_for_0.26g_versions_and_later_2."Idle" ("Enum") State_Type_Definitions,_for_0.26g_versions_and_later_2."Shutdown" ("Enum")] -> w1847
              tunnel: w1849 -> [w1856 _]
              tunnel: w1854 -> [w1861 w1879]
              tunnel: w1845 -> [w1860 _]
              frame "Start Task 1", Default {
                # ">> Is time up? >>"
                # "Determines if object is in range to pick up"
                # ">> Manual override >>"
                n627 = case shown="True" w1860 {
                  tunnel: [w1869 w1875] -> w1865
                  tunnel: w1861 -> [w1867 w1873]
                  frame False {
                    n628 = for {
                      tunnel: string[] ["CLOSE CLAW", "START TIMER"] ("element") -> [w1870] mode=indexing
                      shift-right: [w1872] -> w1869
                      shift-left: w1867 -> [w1871]
                      n629 = Enqueue Element(queue=w1871, element=w1870) -> (queue out=w1872:refnum<queue>)  [unwired: 2 in, 2 out]
                    }
                  }
                  frame True {
                    n630 = for {
                      shift-right: [w1877] -> w1875
                      shift-left: w1873 -> [w1878]
                      tunnel: string[] ["READ STEPPER VALUES", "", ""] -> [w1876] mode=indexing
                      n631 = Enqueue Element(queue=w1878, element=w1876) -> (queue out=w1877:refnum<queue>)  [unwired: 2 in, 2 out]
                    }
                  }
                }
                n632 = Or(x=w1860, y=w1856) -> (x .or. y?=w1863:bool)
                n633 = Select(t=State_Type_Definitions,_for_0.26g_versions_and_later_2."True Stop" ("Enum"), s=w1856, f=State_Type_Definitions,_for_0.26g_versions_and_later_2."Task 8K: RAISE MY SWORD" ("Enum")) -> (s? t:f=w1858:T16)
                n634 = Select(t=w1858, s=w1863, f=State_Type_Definitions,_for_0.26g_versions_and_later_2."Task 8J: CLOSE CLAW" ("Enum")) -> (s? t:f=w1862:T16)
              }
              frame "Exit" {
                n635 = for {
                  shift-right: [w1885] -> w1882
                  shift-left: w1879 -> [w1886]
                  tunnel: string[] ["STOP", "RESET ENCODERS", "RESET YAW", "ARDUINO MODE 0"] -> [w1884] mode=indexing
                  n636 = Enqueue Element(queue=w1886, element=w1884) -> (queue out=w1885:refnum<queue>)  [unwired: 2 in, 2 out]
                }
              }
            }
          }
          frame 37 {
            # ">>> yStepper command>>>"
            # ">> Manual override >>"
            n637 = Dequeue Element(queue=w1897, timeout in ms (-1)=w1896, error in (no error)=w1898) -> (element=w1895:T8)  [unwired: 3 out]
            n638 = Equal?(x=w1894, y=u8 60) -> (x = y?=w1892:bool)
            n639 = case shown="\"Start Task 1\", Default" w1895 {
              tunnel: [w1908 State_Type_Definitions,_for_0.26g_versions_and_later_2."True Stop" ("Enum")] -> w1899
              tunnel: [w1911 w1928] -> w1900
              tunnel: [State_Type_Definitions,_for_0.26g_versions_and_later_2."Idle" ("Enum") State_Type_Definitions,_for_0.26g_versions_and_later_2."Shutdown" ("Enum")] -> w1901
              tunnel: w1892 -> [w1907 _]
              tunnel: w1891 -> [w1906 _]
              tunnel: w1890 -> [w1902 w1925]
              frame "Start Task 1", Default {
                # "Stays in Task 5_A until stepper reaches desired \nheight"
                # "T: Go back to idle, F: Continue with task\""
                # ">> Manual override >>"
                n640 = case shown="True" w1907 {
                  tunnel: [w1915 w1921] -> w1911
                  tunnel: w1902 -> [w1913 w1919]
                  frame False {
                    n641 = for {
                      tunnel: string[] ["Z STEPPER CAM HEIGHT", "READ STEPPER VALUES"] ("element") -> [w1916] mode=indexing
                      shift-right: [w1918] -> w1915
                      shift-left: w1913 -> [w1917]
                      n642 = Enqueue Element(queue=w1917, element=w1916) -> (queue out=w1918:refnum<queue>)  [unwired: 2 in, 2 out]
                    }
                  }
                  frame True {
                    n643 = for {
                      shift-right: [w1923] -> w1921
                      shift-left: w1919 -> [w1924]
                      tunnel: string[] ["CAM CLOSE", "DISPOSE CAM BUFFERS", "DISPOSE PROC BUFFERS", "RESET ENCODERS"] -> [w1922] mode=indexing
                      n644 = Enqueue Element(queue=w1924, element=w1922) -> (queue out=w1923:refnum<queue>)  [unwired: 2 in, 2 out]
                    }
                  }
                }
                n645 = Or(x=w1907, y=w1906) -> (x .or. y?=w1909:bool)
                n646 = Select(t=State_Type_Definitions,_for_0.26g_versions_and_later_2."True Stop" ("Enum"), s=w1906, f=State_Type_Definitions,_for_0.26g_versions_and_later_2."True Stop" ("Enum")) -> (s? t:f=w1903:T16)
                n647 = Select(t=w1903, s=w1909, f=State_Type_Definitions,_for_0.26g_versions_and_later_2."Task 8K: RAISE MY SWORD" ("Enum")) -> (s? t:f=w1908:T16)
              }
              frame "Exit" {
                n648 = for {
                  shift-right: [w1931] -> w1928
                  shift-left: w1925 -> [w1932]
                  tunnel: string[] ["STOP", "RESET ENCODERS", "RESET YAW", "ARDUINO MODE 0"] -> [w1930] mode=indexing
                  n649 = Enqueue Element(queue=w1932, element=w1930) -> (queue out=w1931:refnum<queue>)  [unwired: 2 in, 2 out]
                }
              }
            }
          }
          frame 38 {
            # ">>> Motor control cluster >>>"
            # ">> Stepper height reeached >>"
            # ">>> yStepper command>>>"
            # ">> Manual override >>"
            n650 = Dequeue Element(queue=w1944, timeout in ms (-1)=w1939, error in (no error)=w1943) -> (element=w1947:T8)  [unwired: 3 out]
            n651 = Equal?(x=w1941, y=u8 40) -> (x = y?=w1945:bool)
            n652 = case shown="\"Start Task 1\", Default" w1947 {
              tunnel: [w1958 State_Type_Definitions,_for_0.26g_versions_and_later_2."True Stop" ("Enum")] -> w1937
              tunnel: [w1956 w1973] -> w1936
              tunnel: w1940 -> [w1955 _]
              tunnel: w1942 -> [w1949 _]
              tunnel: [State_Type_Definitions,_for_0.26g_versions_and_later_2."Idle" ("Enum") State_Type_Definitions,_for_0.26g_versions_and_later_2."Shutdown" ("Enum")] -> w1938
              tunnel: w1945 -> [w1948 _]
              frame "Start Task 1", Default {
                # ">> WIill proceed to part ii if not manual override >>"
                # ">>If ENABLE or Trigger is set to true>>"
                n653 = Or(x=w1948, y=w1949) -> (x .or. y?=w1950:bool)
                n654 = case shown="True" w1948 {
                  tunnel: [w1961 w1967] -> w1956
                  tunnel: w1955 -> [w1960 w1966]
                  frame False {
                    n655 = for {
                      shift-right: [w1963] -> w1961
                      shift-left: w1960 -> [w1964]
                      tunnel: string[] ["Z STEPPER BOX HEIGHT", "READ STEPPER VALUES"] ("element") -> [w1962] mode=indexing
                      n656 = Enqueue Element(queue=w1964, element=w1962) -> (queue out=w1963:refnum<queue>)  [unwired: 2 in, 2 out]
                    }
                  }
                  frame True {
                    n657 = for {
                      shift-right: [w1969] -> w1967
                      shift-left: w1966 -> [w1970]
                      tunnel: string[] ["ARDUINO - ULTRASONIC", "READ NAVX", "RESET FLAGS", "", "", ""] -> [w1968] mode=indexing
                      n658 = Enqueue Element(queue=w1970, element=w1968) -> (queue out=w1969:refnum<queue>)  [unwired: 2 in, 2 out]
                    }
                  }
                }
                n659 = Select(t=State_Type_Definitions,_for_0.26g_versions_and_later_2."True Stop" ("Enum"), s=w1949, f=State_Type_Definitions,_for_0.26g_versions_and_later_2."Task 9B: Rotate to Angle" ("Enum")) -> (s? t:f=w1952:T16)
                n660 = Select(t=w1952, s=w1950, f=State_Type_Definitions,_for_0.26g_versions_and_later_2."Task 9A: Raise Arm" ("Enum")) -> (s? t:f=w1958:T16)
              }
              frame "Exit" {
                n661 = for {
                  shift-right: [w1976] -> w1973
                  shift-left: _ -> [w1977]
                  tunnel: string[] ["STOP", "RESET ENCODERS", "RESET YAW", ""] -> [w1975] mode=indexing
                  n662 = Enqueue Element(queue=w1977, element=w1975) -> (queue out=w1976:refnum<queue>)  [unwired: 2 in, 2 out]
                }
              }
            }
          }
          frame 39 {
            # ">>> Motor control cluster >>>"
            # ">>> yStepper command>>>"
            n663 = Dequeue Element(queue=w1991, timeout in ms (-1)=w1990, error in (no error)=w1989) -> (element=w1993:T8)  [unwired: 3 out]
            n664 = In Range and Coerce(upper limit=65.0, x=w1983, lower limit=55.0) -> (In Range?=w1980:bool)  [unwired: 1 out]
            n665 = case shown="\"Start Task 1\", Default" w1993 {
              tunnel: w1984 -> [w1996 _]
              tunnel: [w2004 State_Type_Definitions,_for_0.26g_versions_and_later_2."True Stop" ("Enum")] -> w1986
              tunnel: w1992 -> [w2002 w2020]
              tunnel: [w2001 w2019] -> w1985
              tunnel: [State_Type_Definitions,_for_0.26g_versions_and_later_2."Idle" ("Enum") State_Type_Definitions,_for_0.26g_versions_and_later_2."Shutdown" ("Enum")] -> w1987
              tunnel: w1980 -> [w1994 _]
              frame "Start Task 1", Default {
                n666 = Or(x=w1994, y=w1996) -> (x .or. y?=w1995:bool)
                n667 = case shown="True" w1994 {
                  tunnel: w2002 -> [w2007 w2013]
                  tunnel: [w2006 w2011] -> w2001
                  frame False {
                    n668 = for {
                      shift-right: [w2009] -> w2006
                      shift-left: w2007 -> [w2010]
                      tunnel: string[] ["READ NAVX", "R-CW", "READ ULTRASONIC"] ("element") -> [w2008] mode=indexing
                      n669 = Enqueue Element(queue=w2010, element=w2008) -> (queue out=w2009:refnum<queue>)  [unwired: 2 in, 2 out]
                    }
                  }
                  frame True {
                    n670 = for {
                      shift-right: [w2015] -> w2011
                      shift-left: w2013 -> [w2016]
                      tunnel: string[] ["STOP", "RESET ENCODERS", "RESET YAW", "ARDUINO - ULTRASONIC", ""] -> [w2014] mode=indexing
                      n671 = Enqueue Element(queue=w2016, element=w2014) -> (queue out=w2015:refnum<queue>)  [unwired: 2 in, 2 out]
                    }
                  }
                }
                n672 = Select(t=State_Type_Definitions,_for_0.26g_versions_and_later_2."True Stop" ("Enum"), s=w1996, f=State_Type_Definitions,_for_0.26g_versions_and_later_2."Task 9C: Detect Box") -> (s? t:f=w1998:T16)
                n673 = Select(t=w1998, s=w1995, f=State_Type_Definitions,_for_0.26g_versions_and_later_2."Task 9B: Rotate to Angle" ("Enum")) -> (s? t:f=w2004:T16)
              }
              frame "Exit" {
                n674 = for {
                  shift-right: [w2023] -> w2019
                  shift-left: w2020 -> [w2024]
                  tunnel: string[] ["STOP", "RESET ENCODERS", "RESET YAW", ""] -> [w2022] mode=indexing
                  n675 = Enqueue Element(queue=w2024, element=w2022) -> (queue out=w2023:refnum<queue>)  [unwired: 2 in, 2 out]
                }
              }
            }
          }
          frame 40 {
            # ">>> Motor control cluster >>>"
            # ">>Line Detected>>"
            # ">>Action Queue>>"
            # ">>> yStepper command>>>"
            n676 = Dequeue Element(queue=w2036, timeout in ms (-1)=w2035, error in (no error)=w2034) -> (element=w2037:T8)  [unwired: 3 out]
            n677 = case shown="\"Start Task 1\", Default" w2037 {
              tunnel: w2032 -> [w2038 _]
              tunnel: [w2048 State_Type_Definitions,_for_0.26g_versions_and_later_2."True Stop" ("Enum")] -> w2029
              tunnel: w2033 -> [w2046 w2064]
              tunnel: [w2045 w2063] -> w2028
              tunnel: [State_Type_Definitions,_for_0.26g_versions_and_later_2."Idle" ("Enum") State_Type_Definitions,_for_0.26g_versions_and_later_2."Shutdown" ("Enum")] -> w2031
              tunnel: w2026 -> [w2039 _]
              frame "Start Task 1", Default {
                n678 = Or(x=w2038, y=w2039) -> (x .or. y?=w2040:bool)
                n679 = case shown="True" w2039 {
                  tunnel: w2046 -> [w2051 w2057]
                  tunnel: [w2050 w2055] -> w2045
                  frame False {
                    n680 = for {
                      shift-right: [w2053] -> w2050
                      shift-left: w2051 -> [w2054]
                      tunnel: string[] ["READ IR", "READ LINE SENSOR", "FORWARD - IR ASSIST"] ("element") -> [w2052] mode=indexing
                      n681 = Enqueue Element(queue=w2054, element=w2052) -> (queue out=w2053:refnum<queue>)  [unwired: 2 in, 2 out]
                    }
                  }
                  frame True {
                    n682 = for {
                      shift-right: [w2059] -> w2055
                      shift-left: w2057 -> [w2060]
                      tunnel: string[] ["STOP", "RESET ENCODERS", "RESET YAW", ""] -> [w2058] mode=indexing
                      n683 = Enqueue Element(queue=w2060, element=w2058) -> (queue out=w2059:refnum<queue>)  [unwired: 2 in, 2 out]
                    }
                  }
                }
                n684 = Select(t=State_Type_Definitions,_for_0.26g_versions_and_later_2."True Stop" ("Enum"), s=w2038, f=State_Type_Definitions,_for_0.26g_versions_and_later_2."Task 9D: MOVE FORWARD") -> (s? t:f=w2042:T16)
                n685 = Select(t=w2042, s=w2040, f=State_Type_Definitions,_for_0.26g_versions_and_later_2."Task 9C: Detect Box" ("Enum")) -> (s? t:f=w2048:T16)
              }
              frame "Exit" {
                n686 = for {
                  shift-right: [w2067] -> w2063
                  shift-left: w2064 -> [w2068]
                  tunnel: string[] ["STOP", "RESET ENCODERS", "RESET YAW", ""] -> [w2066] mode=indexing
                  n687 = Enqueue Element(queue=w2068, element=w2066) -> (queue out=w2067:refnum<queue>)  [unwired: 2 in, 2 out]
                }
              }
            }
          }
          frame 41 {
            w2072 = u8 35 ("y")
            # ">> Wall detected >>"
            # ">> Manual override >>"
            # ">>Table Detected>>"
            # ">>> Motor control cluster >>>"
            # ">>Table or wall detectected>>"
            # ">>Action Queue>>"
            # ">>> yStepper command>>>"
            n688 = Less?(x=w2076, y=w2072) -> (x < y?=w2074:bool)
            n689 = Less?(x=w2075, y=w2072) -> (x < y?=w2073:bool)
            n690 = Less Or Equal?(x=w2078, y=15.0) -> (x <= y?=w2069:bool)
            n691 = And(x=w2074, y=w2073) -> (x .and. y?=w2071:bool)
            "Front Wall detected" <- w2071
            n692 = Dequeue Element(queue=w2089, timeout in ms (-1)=w2088, error in (no error)=w2087) -> (element=w2090:T8)  [unwired: 3 out]
            n693 = Or(x=w2069, y=w2071) -> (x .or. y?=w2070:bool)
            n694 = case shown="\"Start Task 1\", Default" w2090 {
              tunnel: w2085 -> [w2091 _]
              tunnel: [w2101 State_Type_Definitions,_for_0.26g_versions_and_later_2."True Stop" ("Enum")] -> w2082
              tunnel: w2086 -> [w2099 w2117]
              tunnel: [w2098 w2116] -> w2081
              tunnel: [State_Type_Definitions,_for_0.26g_versions_and_later_2."Idle" ("Enum") State_Type_Definitions,_for_0.26g_versions_and_later_2."Shutdown" ("Enum")] -> w2084
              tunnel: w2070 -> [w2092 _]
              frame "Start Task 1", Default {
                n695 = Or(x=w2091, y=w2092) -> (x .or. y?=w2093:bool)
                n696 = case shown="False" w2092 {
                  tunnel: w2099 -> [w2104 w2110]
                  tunnel: [w2103 w2108] -> w2098
                  frame False {
                    n697 = for {
                      shift-right: [w2106] -> w2103
                      shift-left: w2104 -> [w2107]
                      tunnel: string[] ["READ IR", "FORWARD - IR ASSIST", "READ ULTRASONIC"] ("element") -> [w2105] mode=indexing
                      n698 = Enqueue Element(queue=w2107, element=w2105) -> (queue out=w2106:refnum<queue>)  [unwired: 2 in, 2 out]
                    }
                  }
                  frame True {
                    n699 = for {
                      shift-right: [w2112] -> w2108
                      shift-left: w2110 -> [w2113]
                      tunnel: string[] ["STOP", "RESET ENCODERS", "RESET YAW", ""] -> [w2111] mode=indexing
                      n700 = Enqueue Element(queue=w2113, element=w2111) -> (queue out=w2112:refnum<queue>)  [unwired: 2 in, 2 out]
                    }
                  }
                }
                n701 = Select(t=State_Type_Definitions,_for_0.26g_versions_and_later_2."True Stop" ("Enum"), s=w2091, f=State_Type_Definitions,_for_0.26g_versions_and_later_2."True Stop") -> (s? t:f=w2095:T16)
                n702 = Select(t=w2095, s=w2093, f=State_Type_Definitions,_for_0.26g_versions_and_later_2."Task 9D: MOVE FORWARD" ("Enum")) -> (s? t:f=w2101:T16)
              }
              frame "Exit" {
                n703 = for {
                  shift-right: [w2120] -> w2116
                  shift-left: w2117 -> [w2121]
                  tunnel: string[] ["STOP", "RESET ENCODERS", "RESET YAW", ""] -> [w2119] mode=indexing
                  n704 = Enqueue Element(queue=w2121, element=w2119) -> (queue out=w2120:refnum<queue>)  [unwired: 2 in, 2 out]
                }
              }
            }
          }
          frame 42 {
            # ">> Item Selection Bias >>"
            # ">> Line detected? >>"
            # ">> Manual override >>"
            # ">>> Motor control cluster >>>"
            # ">>Action Queue>>"
            # ">>> yStepper command>>>"
            n705 = Dequeue Element(queue=w2133, timeout in ms (-1)=w2132, error in (no error)=w2131) -> (element=w2134:T8)  [unwired: 3 out]
            n706 = case shown="\"Start Task 1\", Default" w2134 {
              tunnel: w2129 -> [w2135 _]
              tunnel: [w2145 State_Type_Definitions,_for_0.26g_versions_and_later_2."True Stop" ("Enum")] -> w2126
              tunnel: w2130 -> [w2143 w2161]
              tunnel: [w2142 w2160] -> w2125
              tunnel: [State_Type_Definitions,_for_0.26g_versions_and_later_2."Idle" ("Enum") State_Type_Definitions,_for_0.26g_versions_and_later_2."Shutdown" ("Enum")] -> w2128
              tunnel: w2122 -> [w2136 _]
              frame "Start Task 1", Default {
                n707 = Or(x=w2135, y=w2136) -> (x .or. y?=w2137:bool)
                n708 = case shown="False" w2136 {
                  tunnel: w2143 -> [w2148 w2154]
                  tunnel: [w2147 w2152] -> w2142
                  frame False {
                    n709 = for {
                      shift-right: [w2150] -> w2147
                      shift-left: w2148 -> [w2151]
                      tunnel: string[] ["LEFT", "READ NAVX", "READ LINE SENSOR", ""] ("element") -> [w2149] mode=indexing
                      n710 = Enqueue Element(queue=w2151, element=w2149) -> (queue out=w2150:refnum<queue>)  [unwired: 2 in, 2 out]
                    }
                  }
                  frame True {
                    n711 = for {
                      shift-right: [w2156] -> w2152
                      shift-left: w2154 -> [w2157]
                      tunnel: string[] ["STOP", "RESET ENCODERS", "RESET YAW", "RESET FLAGS", "OPEN LIFE CAM", "SET TIMER 2"] -> [w2155] mode=indexing
                      n712 = Enqueue Element(queue=w2157, element=w2155) -> (queue out=w2156:refnum<queue>)  [unwired: 2 in, 2 out]
                    }
                  }
                }
                n713 = Select(t=State_Type_Definitions,_for_0.26g_versions_and_later_2."True Stop" ("Enum"), s=w2135, f=State_Type_Definitions."Task 9F: SCAN IMAGE") -> (s? t:f=w2139:u16)
                n714 = Select(t=w2139, s=w2137, f=State_Type_Definitions,_for_0.26g_versions_and_later_2."Task 9E: MOVE LEFT" ("Enum")) -> (s? t:f=w2145:u16)
              }
              frame "Exit" {
                n715 = for {
                  shift-right: [w2164] -> w2160
                  shift-left: w2161 -> [w2165]
                  tunnel: string[] ["STOP", "RESET ENCODERS", "RESET YAW", ""] -> [w2163] mode=indexing
                  n716 = Enqueue Element(queue=w2165, element=w2163) -> (queue out=w2164:refnum<queue>)  [unwired: 2 in, 2 out]
                }
              }
            }
          }
          frame 43 {
            # ">>> Motor control cluster >>>"
            # ">>Time up? >>"
            # ">>> yStepper command>>>"
            # ">> Manual override >>"
            n717 = Dequeue Element(queue=w2177, timeout in ms (-1)=w2173, error in (no error)=w2176) -> (element=w2178:T8)  [unwired: 3 out]
            n718 = case shown="\"Start Task 1\", Default" w2178 {
              tunnel: [w2189 State_Type_Definitions,_for_0.26g_versions_and_later_2."True Stop" ("Enum")] -> w2171
              tunnel: [w2187 w2205] -> w2170
              tunnel: w2174 -> [w2186 w2202]
              tunnel: w2175 -> [w2180 _]
              tunnel: [State_Type_Definitions,_for_0.26g_versions_and_later_2."Idle" ("Enum") State_Type_Definitions,_for_0.26g_versions_and_later_2."Shutdown" ("Enum")] -> w2172
              tunnel: w2166 -> [w2179 _]
              frame "Start Task 1", Default {
                # ">> WIill proceed to part ii if not manual override >>"
                # ">>If ENABLE or Trigger is set to true>>"
                n719 = Or(x=w2179, y=w2180) -> (x .or. y?=w2181:bool)
                n720 = case shown="True" w2179 {
                  tunnel: [w2192 w2198] -> w2187
                  tunnel: w2186 -> [w2191 w2197]
                  frame False {
                    n721 = for {
                      shift-right: [w2194] -> w2192
                      shift-left: w2191 -> [w2195]
                      tunnel: string[] ["CAM ACQ", "START TIMER"] ("element") -> [w2193] mode=indexing
                      n722 = Enqueue Element(queue=w2195, element=w2193) -> (queue out=w2194:refnum<queue>)  [unwired: 2 in, 2 out]
                    }
                  }
                  frame True {
                    n723 = for {
                      shift-right: [w2200] -> w2198
                      shift-left: w2197 -> [w2201]
                      tunnel: string[] ["CLOSE CAM", "SET TIMER 5", "", "", "", ""] -> [w2199] mode=indexing
                      n724 = Enqueue Element(queue=w2201, element=w2199) -> (queue out=w2200:refnum<queue>)  [unwired: 2 in, 2 out]
                    }
                  }
                }
                n725 = Select(t=State_Type_Definitions,_for_0.26g_versions_and_later_2."True Stop" ("Enum"), s=w2180, f=State_Type_Definitions."Task 9G: PROCESS COLOUR" ("Enum")) -> (s? t:f=w2183:u16)
                n726 = Select(t=w2183, s=w2181, f=State_Type_Definitions."Task 9F: SCAN IMAGE" ("Enum")) -> (s? t:f=w2189:u16)
              }
              frame "Exit" {
                n727 = for {
                  shift-right: [w2208] -> w2205
                  shift-left: w2202 -> [w2209]
                  tunnel: string[] ["STOP", "RESET ENCODERS", "RESET YAW", ""] -> [w2207] mode=indexing
                  n728 = Enqueue Element(queue=w2209, element=w2207) -> (queue out=w2208:refnum<queue>)  [unwired: 2 in, 2 out]
                }
              }
            }
          }
          frame 44 {
            # ">>> Motor control cluster >>>"
            # ">>> yStepper command>>>"
            # ">>Object detected>>"
            n729 = Less Or Equal?(x=w2213, y=30.0) -> (x <= y?=w2211:bool)
            "Table obstruct" <- w2211
            n730 = Dequeue Element(queue=w2219, timeout in ms (-1)=w2218, error in (no error)=w2217) -> (element=w2224:T8)  [unwired: 3 out]
            n731 = case shown="\"Start Task 1\", Default" w2224 {
              tunnel: w2211 -> [w2227 _]
              tunnel: [w2234 State_Type_Definitions,_for_0.26g_versions_and_later_2."True Stop" ("Enum")] -> w2223
              tunnel: w2216 -> [w2226 _]
              tunnel: w2220 -> [w2233 w2250]
              tunnel: [w2232 w2251] -> w2222
              tunnel: [State_Type_Definitions,_for_0.26g_versions_and_later_2."Idle" ("Enum") State_Type_Definitions,_for_0.26g_versions_and_later_2."Shutdown" ("Enum")] -> w2221
              frame "Start Task 1", Default {
                n732 = case shown="True" w2227 {
                  tunnel: w2233 -> [w2237 w2244]
                  tunnel: [w2238 w2243] -> w2232
                  frame False {
                    n733 = for {
                      tunnel: string[] ["START TIMER", "COLOUR PROCESSING", ""] ("element") -> [w2239] mode=indexing
                      shift-right: [w2241] -> w2238
                      shift-left: w2237 -> [w2240]
                      n734 = Enqueue Element(queue=w2240, element=w2239) -> (queue out=w2241:refnum<queue>)  [unwired: 2 in, 2 out]
                    }
                  }
                  frame True {
                    n735 = for {
                      shift-right: [w2246] -> w2243
                      shift-left: w2244 -> [w2247]
                      tunnel: string[] ["DISPOSE BUFFERS", "CLOSE CAM", "RESET ENCODERS", "RESET YAW", "RESET FLAGS"] -> [w2245] mode=indexing
                      n736 = Enqueue Element(queue=w2247, element=w2245) -> (queue out=w2246:refnum<queue>)  [unwired: 2 in, 2 out]
                    }
                  }
                }
                n737 = Or(x=w2227, y=w2226) -> (x .or. y?=w2225:bool)
                n738 = Select(t=State_Type_Definitions,_for_0.26g_versions_and_later_2."True Stop" ("Enum"), s=w2226, f=State_Type_Definitions."Task 9H: MOVE RIGHT" ("Enum")) -> (s? t:f=w2228:u16)
                n739 = Select(t=w2228, s=w2225, f=State_Type_Definitions."Task 9G: PROCESS COLOUR" ("Enum")) -> (s? t:f=w2234:u16)
              }
              frame "Exit" {
                n740 = for {
                  shift-right: [w2254] -> w2251
                  shift-left: w2250 -> [w2255]
                  tunnel: string[] ["STOP", "RESET ENCODERS", "RESET YAW", "ARDUINO MODE 0"] -> [w2253] mode=indexing
                  n741 = Enqueue Element(queue=w2255, element=w2253) -> (queue out=w2254:refnum<queue>)  [unwired: 2 in, 2 out]
                }
              }
            }
          }
          frame 45 {
            # ">> Item Selection Bias >>"
            # ">>> Motor control cluster >>>"
            # ">>> yStepper command>>>"
            n742 = Dequeue Element(queue=w2265, timeout in ms (-1)=w2266, error in (no error)=w2267) -> (element=w2269:T8)  [unwired: 3 out]
            n743 = Greater?(x=w2257, y=50.0) -> (0:w2258:bool)
            n744 = And(x=w2259, y=w2258) -> (x .and. y?=w2260:bool)
            n745 = case shown="\"Start Task 1\", Default" w2269 {
              tunnel: w2260 -> [w2275 _]
              tunnel: [w2282 State_Type_Definitions,_for_0.26g_versions_and_later_2."True Stop" ("Enum")] -> w2262
              tunnel: w2268 -> [w2274 _]
              tunnel: w2264 -> [w2281 w2298]
              tunnel: [w2280 w2299] -> w2263
              tunnel: [State_Type_Definitions,_for_0.26g_versions_and_later_2."Idle" ("Enum") State_Type_Definitions,_for_0.26g_versions_and_later_2."Shutdown" ("Enum")] -> w2261
              frame "Start Task 1", Default {
                n746 = case shown="False" w2275 {
                  tunnel: w2281 -> [w2285 w2292]
                  tunnel: [w2286 w2291] -> w2280
                  frame False {
                    n747 = for {
                      tunnel: string[] ["READ LINE SENSOR", "READ NAVX", "RIGHT", "READ ENCODERS"] ("element") -> [w2287] mode=indexing
                      shift-right: [w2289] -> w2286
                      shift-left: w2285 -> [w2288]
                      n748 = Enqueue Element(queue=w2288, element=w2287) -> (queue out=w2289:refnum<queue>)  [unwired: 2 in, 2 out]
                    }
                  }
                  frame True {
                    n749 = for {
                      shift-right: [w2294] -> w2291
                      shift-left: w2292 -> [w2295]
                      tunnel: string[] ["STOP", "RESET ENCODERS", "RESET YAW", "OPEN LIFE CAM", "SET TIMER 2", "RESET FLAGS"] -> [w2293] mode=indexing
                      n750 = Enqueue Element(queue=w2295, element=w2293) -> (queue out=w2294:refnum<queue>)  [unwired: 2 in, 2 out]
                    }
                  }
                }
                n751 = Or(x=w2275, y=w2274) -> (x .or. y?=w2273:bool)
                n752 = Select(t=State_Type_Definitions,_for_0.26g_versions_and_later_2."True Stop" ("Enum"), s=w2274, f=State_Type_Definitions."Task 9I: SCAN IMAGE" ("Enum")) -> (s? t:f=w2276:u16)
                n753 = Select(t=w2276, s=w2273, f=State_Type_Definitions."Task 9H: MOVE RIGHT" ("Enum")) -> (s? t:f=w2282:u16)
              }
              frame "Exit" {
                n754 = for {
                  shift-right: [w2302] -> w2299
                  shift-left: w2298 -> [w2303]
                  tunnel: string[] ["STOP", "RESET ENCODERS", "RESET YAW", "ARDUINO MODE 0"] -> [w2301] mode=indexing
                  n755 = Enqueue Element(queue=w2303, element=w2301) -> (queue out=w2302:refnum<queue>)  [unwired: 2 in, 2 out]
                }
              }
            }
          }
          frame 46 {
            # ">> Item Selection Bias >>"
            n756 = Dequeue Element(queue=w2305, timeout in ms (-1)=w2306, error in (no error)=w2307) -> (element=w2313:T8)  [unwired: 3 out]
            n757 = case shown="\"Start Task 1\", Default" w2313 {
              tunnel: w2304 -> [w2319 _]
              tunnel: [w2326 State_Type_Definitions,_for_0.26g_versions_and_later_2."True Stop" ("Enum")] -> w2310
              tunnel: w2308 -> [w2318 _]
              tunnel: w2312 -> [w2325 w2342]
              tunnel: [w2324 w2343] -> w2311
              tunnel: [State_Type_Definitions,_for_0.26g_versions_and_later_2."Idle" ("Enum") State_Type_Definitions,_for_0.26g_versions_and_later_2."Shutdown" ("Enum")] -> w2309
              frame "Start Task 1", Default {
                n758 = case shown="True" w2319 {
                  tunnel: w2325 -> [w2329 w2336]
                  tunnel: [w2330 w2335] -> w2324
                  frame False {
                    n759 = for {
                      tunnel: string[] ["START TIMER", "CAM ACQ", ""] ("element") -> [w2331] mode=indexing
                      shift-right: [w2333] -> w2330
                      shift-left: w2329 -> [w2332]
                      n760 = Enqueue Element(queue=w2332, element=w2331) -> (queue out=w2333:refnum<queue>)  [unwired: 2 in, 2 out]
                    }
                  }
                  frame True {
                    n761 = for {
                      shift-right: [w2338] -> w2335
                      shift-left: w2336 -> [w2339]
                      tunnel: string[] ["CLOSE CAM", "SET TIMER 5", "", "", "", ""] -> [w2337] mode=indexing
                      n762 = Enqueue Element(queue=w2339, element=w2337) -> (queue out=w2338:refnum<queue>)  [unwired: 2 in, 2 out]
                    }
                  }
                }
                n763 = Or(x=w2319, y=w2318) -> (x .or. y?=w2317:bool)
                n764 = Select(t=State_Type_Definitions,_for_0.26g_versions_and_later_2."True Stop" ("Enum"), s=w2318, f=State_Type_Definitions."Task 9J: PROCESS COLOUR" ("Enum")) -> (s? t:f=w2320:u16)
                n765 = Select(t=w2320, s=w2317, f=State_Type_Definitions."Task 9I: SCAN IMAGE" ("Enum")) -> (s? t:f=w2326:u16)
              }
              frame "Exit" {
                n766 = for {
                  shift-right: [w2346] -> w2343
                  shift-left: w2342 -> [w2347]
                  tunnel: string[] ["STOP", "RESET ENCODERS", "RESET YAW", "ARDUINO MODE 0"] -> [w2345] mode=indexing
                  n767 = Enqueue Element(queue=w2347, element=w2345) -> (queue out=w2346:refnum<queue>)  [unwired: 2 in, 2 out]
                }
              }
            }
          }
          frame 47 {
            # ">> Item Selection Bias >>"
            n768 = Dequeue Element(queue=w2353, timeout in ms (-1)=w2354, error in (no error)=w2355) -> (element=w2357:T8)  [unwired: 3 out]
            n769 = case shown="\"Start Task 1\", Default" w2357 {
              tunnel: w2348 -> [w2363 _]
              tunnel: [w2370 State_Type_Definitions,_for_0.26g_versions_and_later_2."True Stop" ("Enum")] -> w2351
              tunnel: w2356 -> [w2362 _]
              tunnel: w2352 -> [w2369 w2386]
              tunnel: [w2368 w2387] -> w2350
              tunnel: [State_Type_Definitions,_for_0.26g_versions_and_later_2."Idle" ("Enum") State_Type_Definitions,_for_0.26g_versions_and_later_2."Shutdown" ("Enum")] -> w2349
              frame "Start Task 1", Default {
                n770 = case shown="True" w2363 {
                  tunnel: w2369 -> [w2373 w2380]
                  tunnel: [w2374 w2379] -> w2368
                  frame False {
                    n771 = for {
                      tunnel: string[] ["START TIMER", "COLOUR PROCESSING", ""] ("element") -> [w2375] mode=indexing
                      shift-right: [w2377] -> w2374
                      shift-left: w2373 -> [w2376]
                      n772 = Enqueue Element(queue=w2376, element=w2375) -> (queue out=w2377:refnum<queue>)  [unwired: 2 in, 2 out]
                    }
                  }
                  frame True {
                    n773 = for {
                      shift-right: [w2382] -> w2379
                      shift-left: w2380 -> [w2383]
                      tunnel: string[] ["CLOSE CAM", "DISPOSE BUFFERS", "RESET ENCODERS", "RESET YAW", "RESET FLAGS", ""] -> [w2381] mode=indexing
                      n774 = Enqueue Element(queue=w2383, element=w2381) -> (queue out=w2382:refnum<queue>)  [unwired: 2 in, 2 out]
                    }
                  }
                }
                n775 = Or(x=w2363, y=w2362) -> (x .or. y?=w2361:bool)
                n776 = Select(t=State_Type_Definitions,_for_0.26g_versions_and_later_2."True Stop" ("Enum"), s=w2362, f=State_Type_Definitions."Task 9K: ROTATE 90 CW" ("Enum")) -> (s? t:f=w2364:u16)
                n777 = Select(t=w2364, s=w2361, f=State_Type_Definitions."Task 9J: PROCESS COLOUR" ("Enum")) -> (s? t:f=w2370:u16)
              }
              frame "Exit" {
                n778 = for {
                  shift-right: [w2390] -> w2387
                  shift-left: w2386 -> [w2391]
                  tunnel: string[] ["STOP", "RESET ENCODERS", "RESET YAW", "ARDUINO MODE 0"] -> [w2389] mode=indexing
                  n779 = Enqueue Element(queue=w2391, element=w2389) -> (queue out=w2390:refnum<queue>)  [unwired: 2 in, 2 out]
                }
              }
            }
          }
          frame 48 {
            # ">>> Motor control cluster >>>"
            # ">>> yStepper command>>>"
            # ">> Item Selection Bias >>"
            n780 = Less?(x=w2395, y=-38.0) -> (x < y?=w2393:bool)
            n781 = Dequeue Element(queue=w2401, timeout in ms (-1)=w2400, error in (no error)=w2399) -> (element=w2403:T8)  [unwired: 3 out]
            n782 = case shown="\"Start Task 1\", Default" w2403 {
              tunnel: w2393 -> [w2409 _]
              tunnel: [w2416 State_Type_Definitions,_for_0.26g_versions_and_later_2."True Stop" ("Enum")] -> w2397
              tunnel: w2398 -> [w2408 _]
              tunnel: w2402 -> [w2415 w2432]
              tunnel: [w2414 w2433] -> w2392
              tunnel: [State_Type_Definitions,_for_0.26g_versions_and_later_2."Idle" ("Enum") State_Type_Definitions,_for_0.26g_versions_and_later_2."Shutdown" ("Enum")] -> w2396
              frame "Start Task 1", Default {
                n783 = case shown="True" w2409 {
                  tunnel: w2415 -> [w2419 w2426]
                  tunnel: [w2420 w2425] -> w2414
                  frame False {
                    n784 = for {
                      tunnel: string[] ["READ ENCODERS", "R-CW"] ("element") -> [w2421] mode=indexing
                      shift-right: [w2423] -> w2420
                      shift-left: w2419 -> [w2422]
                      n785 = Enqueue Element(queue=w2422, element=w2421) -> (queue out=w2423:refnum<queue>)  [unwired: 2 in, 2 out]
                    }
                  }
                  frame True {
                    n786 = for {
                      shift-right: [w2428] -> w2425
                      shift-left: w2426 -> [w2429]
                      tunnel: string[] ["STOP", "RESET ENCODERS", "RESET FLAGS", "RESET YAW", "READ IR", "ARDUINO - ULTRASONIC"] -> [w2427] mode=indexing
                      n787 = Enqueue Element(queue=w2429, element=w2427) -> (queue out=w2428:refnum<queue>)  [unwired: 2 in, 2 out]
                    }
                  }
                }
                n788 = Or(x=w2409, y=w2408) -> (x .or. y?=w2407:bool)
                n789 = Select(t=State_Type_Definitions,_for_0.26g_versions_and_later_2."True Stop" ("Enum"), s=w2408, f=State_Type_Definitions."Task 9L: MOVE FORWARD" ("Enum")) -> (s? t:f=w2410:u16)
                n790 = Select(t=w2410, s=w2407, f=State_Type_Definitions."Task 9K: ROTATE 90 CW" ("Enum")) -> (s? t:f=w2416:u16)
              }
              frame "Exit" {
                n791 = for {
                  shift-right: [w2436] -> w2433
                  shift-left: w2432 -> [w2437]
                  tunnel: string[] ["STOP", "RESET ENCODERS", "RESET YAW", "ARDUINO MODE 0"] -> [w2435] mode=indexing
                  n792 = Enqueue Element(queue=w2437, element=w2435) -> (queue out=w2436:refnum<queue>)  [unwired: 2 in, 2 out]
                }
              }
            }
          }
          frame 49 {
            w2450 = u8 50 ("y")
            # ">>> Motor control cluster >>>"
            # ">>> yStepper command>>>"
            # ">> Item Selection Bias >>"
            n793 = Less?(x=w2452, y=w2450) -> (x < y?=w2445:bool)
            n794 = Dequeue Element(queue=w2456, timeout in ms (-1)=w2455, error in (no error)=w2454) -> (element=w2460:T8)  [unwired: 3 out]
            n795 = Less?(x=w2451, y=w2450) -> (x < y?=w2446:bool)
            n796 = And(x=w2446, y=w2445) -> (x .and. y?=w2438:bool)
            n797 = Less Or Equal?(x=w2449, y=15.0) -> (x <= y?=w2444:bool)
            n798 = Greater?(x=w2443, y=100.0) -> (0:w2442:bool)
            n799 = Or(x=w2444, y=w2438) -> (x .or. y?=w2440:bool)
            n800 = And(x=w2442, y=w2440) -> (x .and. y?=w2441:bool)
            "Stop?" <- w2441
            n801 = case shown="\"Start Task 1\", Default" w2460 {
              tunnel: w2441 -> [w2466 _]
              tunnel: [w2473 State_Type_Definitions,_for_0.26g_versions_and_later_2."True Stop" ("Enum")] -> w2458
              tunnel: w2453 -> [w2465 _]
              tunnel: w2457 -> [w2472 w2489]
              tunnel: [w2471 w2490] -> w2447
              tunnel: [State_Type_Definitions,_for_0.26g_versions_and_later_2."Idle" ("Enum") State_Type_Definitions,_for_0.26g_versions_and_later_2."Shutdown" ("Enum")] -> w2459
              frame "Start Task 1", Default {
                n802 = case shown="True" w2466 {
                  tunnel: w2472 -> [w2476 w2483]
                  tunnel: [w2477 w2482] -> w2471
                  frame False {
                    n803 = for {
                      tunnel: string[] ["READ IR", "FORWARD", "READ NAVX", "READ ENCODERS"] ("element") -> [w2478] mode=indexing
                      shift-right: [w2480] -> w2477
                      shift-left: w2476 -> [w2479]
                      n804 = Enqueue Element(queue=w2479, element=w2478) -> (queue out=w2480:refnum<queue>)  [unwired: 2 in, 2 out]
                    }
                  }
                  frame True {
                    n805 = for {
                      shift-right: [w2485] -> w2482
                      shift-left: w2483 -> [w2486]
                      tunnel: string[] ["STOP", "RESET ENCODERS", "RESET FLAGS", "RESET YAW", "", ""] -> [w2484] mode=indexing
                      n806 = Enqueue Element(queue=w2486, element=w2484) -> (queue out=w2485:refnum<queue>)  [unwired: 2 in, 2 out]
                    }
                  }
                }
                n807 = Or(x=w2466, y=w2465) -> (x .or. y?=w2464:bool)
                n808 = Select(t=State_Type_Definitions,_for_0.26g_versions_and_later_2."True Stop" ("Enum"), s=w2465, f=State_Type_Definitions,_for_0.26g_versions_and_later_2."True Stop" ("Enum")) -> (s? t:f=w2467:T16)
                n809 = Select(t=w2467, s=w2464, f=State_Type_Definitions."Task 9L: MOVE FORWARD" ("Enum")) -> (s? t:f=w2473:u16)
              }
              frame "Exit" {
                n810 = for {
                  shift-right: [w2493] -> w2490
                  shift-left: w2489 -> [w2494]
                  tunnel: string[] ["STOP", "RESET ENCODERS", "RESET YAW", "ARDUINO MODE 0"] -> [w2492] mode=indexing
                  n811 = Enqueue Element(queue=w2494, element=w2492) -> (queue out=w2493:refnum<queue>)  [unwired: 2 in, 2 out]
                }
              }
            }
          }
          frame 50 {
            # ">> Item Selection Bias >>"
            n812 = Dequeue Element(queue=w2499, timeout in ms (-1)=w2498, error in (no error)=w2497) -> (element=w2504:T8)  [unwired: 3 out]
            n813 = case shown="\"Start Task 1\", Default" w2504 {
              tunnel: w2495 -> [w2510 _]
              tunnel: [w2517 State_Type_Definitions,_for_0.26g_versions_and_later_2."True Stop" ("Enum")] -> w2502
              tunnel: w2496 -> [w2509 _]
              tunnel: w2500 -> [w2516 w2533]
              tunnel: [w2515 w2534] -> w2501
              tunnel: [State_Type_Definitions,_for_0.26g_versions_and_later_2."Idle" ("Enum") State_Type_Definitions,_for_0.26g_versions_and_later_2."Shutdown" ("Enum")] -> w2503
              frame "Start Task 1", Default {
                n814 = case shown="False" w2510 {
                  tunnel: w2516 -> [w2520 w2527]
                  tunnel: [w2521 w2526] -> w2515
                  frame False {
                    n815 = for {
                      tunnel: string[] ["READ LINE SENSOR", "READ NAVX", "RIGHT", "READ ENCODERS"] ("element") -> [w2522] mode=indexing
                      shift-right: [w2524] -> w2521
                      shift-left: w2520 -> [w2523]
                      n816 = Enqueue Element(queue=w2523, element=w2522) -> (queue out=w2524:refnum<queue>)  [unwired: 2 in, 2 out]
                    }
                  }
                  frame True {
                    n817 = for {
                      shift-right: [w2529] -> w2526
                      shift-left: w2527 -> [w2530]
                      tunnel: string[] ["STOP", "RESET ENCODERS", "RESET YAW", "OPEN LIFE CAM", "SET TIMER 2", "RESET FLAGS"] -> [w2528] mode=indexing
                      n818 = Enqueue Element(queue=w2530, element=w2528) -> (queue out=w2529:refnum<queue>)  [unwired: 2 in, 2 out]
                    }
                  }
                }
                n819 = Or(x=w2510, y=w2509) -> (x .or. y?=w2508:bool)
                n820 = Select(t=State_Type_Definitions,_for_0.26g_versions_and_later_2."True Stop" ("Enum"), s=w2509, f=State_Type_Definitions."Task 9N: SCAN IMAGE" ("Enum")) -> (s? t:f=w2511:u16)
                n821 = Select(t=w2511, s=w2508, f=State_Type_Definitions,_for_0.26g_versions_and_later_2."Task 9M: MOVE RIGHT" ("Enum")) -> (s? t:f=w2517:u16)
              }
              frame "Exit" {
                n822 = for {
                  shift-right: [w2537] -> w2534
                  shift-left: w2533 -> [w2538]
                  tunnel: string[] ["STOP", "RESET ENCODERS", "RESET YAW", "ARDUINO MODE 0"] -> [w2536] mode=indexing
                  n823 = Enqueue Element(queue=w2538, element=w2536) -> (queue out=w2537:refnum<queue>)  [unwired: 2 in, 2 out]
                }
              }
            }
          }
          frame 51 {
            # ">> Manual override >>"
            n824 = Dequeue Element(queue=w2547, timeout in ms (-1)=w2546, error in (no error)=w2545) -> (element=w2548:T8)  [unwired: 3 out]
            n825 = case shown="\"Start Task 1\", Default" w2548 {
              tunnel: [w2562 State_Type_Definitions,_for_0.26g_versions_and_later_2."True Stop" ("Enum")] -> w2540
              tunnel: [w2560 w2578] -> w2539
              tunnel: w2543 -> [w2559 w2575]
              tunnel: w2544 -> [w2553 _]
              tunnel: [State_Type_Definitions,_for_0.26g_versions_and_later_2."Idle" ("Enum") State_Type_Definitions,_for_0.26g_versions_and_later_2."Shutdown" ("Enum")] -> w2541
              tunnel: w2542 -> [w2552 _]
              frame "Start Task 1", Default {
                # ">> WIill proceed to part ii if not manual override >>"
                # ">>If ENABLE or Trigger is set to true>>"
                n826 = Or(x=w2552, y=w2553) -> (x .or. y?=w2554:bool)
                n827 = case shown="False" w2552 {
                  tunnel: [w2565 w2571] -> w2560
                  tunnel: w2559 -> [w2564 w2570]
                  frame False {
                    n828 = for {
                      shift-right: [w2567] -> w2565
                      shift-left: w2564 -> [w2568]
                      tunnel: string[] ["CAM ACQ", "START TIMER"] ("element") -> [w2566] mode=indexing
                      n829 = Enqueue Element(queue=w2568, element=w2566) -> (queue out=w2567:refnum<queue>)  [unwired: 2 in, 2 out]
                    }
                  }
                  frame True {
                    n830 = for {
                      shift-right: [w2573] -> w2571
                      shift-left: w2570 -> [w2574]
                      tunnel: string[] ["CLOSE CAM", "SET TIMER 5", "", "", "", ""] -> [w2572] mode=indexing
                      n831 = Enqueue Element(queue=w2574, element=w2572) -> (queue out=w2573:refnum<queue>)  [unwired: 2 in, 2 out]
                    }
                  }
                }
                n832 = Select(t=State_Type_Definitions,_for_0.26g_versions_and_later_2."True Stop" ("Enum"), s=w2553, f=State_Type_Definitions."Task 9O: PROCESS COLOUR" ("Enum")) -> (s? t:f=w2556:u16)
                n833 = Select(t=w2556, s=w2554, f=State_Type_Definitions."Task 9N: SCAN IMAGE" ("Enum")) -> (s? t:f=w2562:u16)
              }
              frame "Exit" {
                n834 = for {
                  shift-right: [w2581] -> w2578
                  shift-left: w2575 -> [w2582]
                  tunnel: string[] ["STOP", "RESET ENCODERS", "RESET YAW", ""] -> [w2580] mode=indexing
                  n835 = Enqueue Element(queue=w2582, element=w2580) -> (queue out=w2581:refnum<queue>)  [unwired: 2 in, 2 out]
                }
              }
            }
          }
          frame 52 {
            # ">> Item Selection Bias >>"
            n836 = Dequeue Element(queue=w2590, timeout in ms (-1)=w2589, error in (no error)=w2588) -> (element=w2592:T8)  [unwired: 3 out]
            n837 = case shown="\"Start Task 1\", Default" w2592 {
              tunnel: w2583 -> [w2598 _]
              tunnel: [w2605 State_Type_Definitions,_for_0.26g_versions_and_later_2."True Stop" ("Enum")] -> w2586
              tunnel: w2587 -> [w2597 _]
              tunnel: w2591 -> [w2604 w2621]
              tunnel: [w2603 w2622] -> w2585
              tunnel: [State_Type_Definitions,_for_0.26g_versions_and_later_2."Idle" ("Enum") State_Type_Definitions,_for_0.26g_versions_and_later_2."Shutdown" ("Enum")] -> w2584
              frame "Start Task 1", Default {
                n838 = case shown="False" w2598 {
                  tunnel: w2604 -> [w2608 w2615]
                  tunnel: [w2609 w2614] -> w2603
                  frame False {
                    n839 = for {
                      tunnel: string[] ["START TIMER", "COLOUR PROCESSING", ""] ("element") -> [w2610] mode=indexing
                      shift-right: [w2612] -> w2609
                      shift-left: w2608 -> [w2611]
                      n840 = Enqueue Element(queue=w2611, element=w2610) -> (queue out=w2612:refnum<queue>)  [unwired: 2 in, 2 out]
                    }
                  }
                  frame True {
                    n841 = for {
                      shift-right: [w2617] -> w2614
                      shift-left: w2615 -> [w2618]
                      tunnel: string[] ["CLOSE CAM", "DISPOSE BUFFERS", "RESET ENCODERS", "RESET YAW", "RESET FLAGS", ""] -> [w2616] mode=indexing
                      n842 = Enqueue Element(queue=w2618, element=w2616) -> (queue out=w2617:refnum<queue>)  [unwired: 2 in, 2 out]
                    }
                  }
                }
                n843 = Or(x=w2598, y=w2597) -> (x .or. y?=w2596:bool)
                n844 = Select(t=State_Type_Definitions,_for_0.26g_versions_and_later_2."True Stop" ("Enum"), s=w2597, f=State_Type_Definitions."Task 9P: MOVE RIGHT" ("Enum")) -> (s? t:f=w2599:u16)
                n845 = Select(t=w2599, s=w2596, f=State_Type_Definitions."Task 9O: PROCESS COLOUR" ("Enum")) -> (s? t:f=w2605:u16)
              }
              frame "Exit" {
                n846 = for {
                  shift-right: [w2625] -> w2622
                  shift-left: w2621 -> [w2626]
                  tunnel: string[] ["STOP", "RESET ENCODERS", "RESET YAW", "ARDUINO MODE 0"] -> [w2624] mode=indexing
                  n847 = Enqueue Element(queue=w2626, element=w2624) -> (queue out=w2625:refnum<queue>)  [unwired: 2 in, 2 out]
                }
              }
            }
          }
          frame 53 {
            # ">> Item Selection Bias >>"
            n848 = Dequeue Element(queue=w2632, timeout in ms (-1)=w2631, error in (no error)=w2630) -> (element=w2640:T8)  [unwired: 3 out]
            n849 = Greater?(x=w2628, y=50.0) -> (0:w2638:bool)
            n850 = And(x=w2627, y=w2638) -> (x .and. y?=w2639:bool)
            n851 = case shown="\"Start Task 1\", Default" w2640 {
              tunnel: w2639 -> [w2646 _]
              tunnel: [w2653 State_Type_Definitions,_for_0.26g_versions_and_later_2."True Stop" ("Enum")] -> w2635
              tunnel: w2629 -> [w2645 _]
              tunnel: w2633 -> [w2652 w2669]
              tunnel: [w2651 w2670] -> w2634
              tunnel: [State_Type_Definitions,_for_0.26g_versions_and_later_2."Idle" ("Enum") State_Type_Definitions,_for_0.26g_versions_and_later_2."Shutdown" ("Enum")] -> w2636
              frame "Start Task 1", Default {
                n852 = case shown="False" w2646 {
                  tunnel: w2652 -> [w2656 w2663]
                  tunnel: [w2657 w2662] -> w2651
                  frame False {
                    n853 = for {
                      tunnel: string[] ["READ LINE SENSOR", "READ NAVX", "RIGHT", "READ ENCODERS"] ("element") -> [w2658] mode=indexing
                      shift-right: [w2660] -> w2657
                      shift-left: w2656 -> [w2659]
                      n854 = Enqueue Element(queue=w2659, element=w2658) -> (queue out=w2660:refnum<queue>)  [unwired: 2 in, 2 out]
                    }
                  }
                  frame True {
                    n855 = for {
                      shift-right: [w2665] -> w2662
                      shift-left: w2663 -> [w2666]
                      tunnel: string[] ["STOP", "RESET ENCODERS", "RESET YAW", "OPEN LIFE CAM", "SET TIMER 2", "RESET FLAGS"] -> [w2664] mode=indexing
                      n856 = Enqueue Element(queue=w2666, element=w2664) -> (queue out=w2665:refnum<queue>)  [unwired: 2 in, 2 out]
                    }
                  }
                }
                n857 = Or(x=w2646, y=w2645) -> (x .or. y?=w2644:bool)
                n858 = Select(t=State_Type_Definitions,_for_0.26g_versions_and_later_2."True Stop" ("Enum"), s=w2645, f=State_Type_Definitions."Task 9Q: SCAN IMAGE" ("Enum")) -> (s? t:f=w2647:u16)
                n859 = Select(t=w2647, s=w2644, f=State_Type_Definitions."Task 9P: MOVE RIGHT" ("Enum")) -> (s? t:f=w2653:u16)
              }
              frame "Exit" {
                n860 = for {
                  shift-right: [w2673] -> w2670
                  shift-left: w2669 -> [w2674]
                  tunnel: string[] ["STOP", "RESET ENCODERS", "RESET YAW", "ARDUINO MODE 0"] -> [w2672] mode=indexing
                  n861 = Enqueue Element(queue=w2674, element=w2672) -> (queue out=w2673:refnum<queue>)  [unwired: 2 in, 2 out]
                }
              }
            }
          }
          frame 54 {
            # ">> Manual override >>"
            n862 = Dequeue Element(queue=w2683, timeout in ms (-1)=w2682, error in (no error)=w2681) -> (element=w2684:T8)  [unwired: 3 out]
            n863 = case shown="\"Start Task 1\", Default" w2684 {
              tunnel: [w2698 State_Type_Definitions,_for_0.26g_versions_and_later_2."True Stop" ("Enum")] -> w2676
              tunnel: [w2696 w2714] -> w2675
              tunnel: w2679 -> [w2695 w2711]
              tunnel: w2680 -> [w2689 _]
              tunnel: [State_Type_Definitions,_for_0.26g_versions_and_later_2."Idle" ("Enum") State_Type_Definitions,_for_0.26g_versions_and_later_2."Shutdown" ("Enum")] -> w2677
              tunnel: w2678 -> [w2688 _]
              frame "Start Task 1", Default {
                # ">> WIill proceed to part ii if not manual override >>"
                # ">>If ENABLE or Trigger is set to true>>"
                n864 = Or(x=w2688, y=w2689) -> (x .or. y?=w2690:bool)
                n865 = case shown="False" w2688 {
                  tunnel: [w2701 w2707] -> w2696
                  tunnel: w2695 -> [w2700 w2706]
                  frame False {
                    n866 = for {
                      shift-right: [w2703] -> w2701
                      shift-left: w2700 -> [w2704]
                      tunnel: string[] ["CAM ACQ", "START TIMER"] ("element") -> [w2702] mode=indexing
                      n867 = Enqueue Element(queue=w2704, element=w2702) -> (queue out=w2703:refnum<queue>)  [unwired: 2 in, 2 out]
                    }
                  }
                  frame True {
                    n868 = for {
                      shift-right: [w2709] -> w2707
                      shift-left: w2706 -> [w2710]
                      tunnel: string[] ["CLOSE CAM", "SET TIMER 5", "", "", "", ""] -> [w2708] mode=indexing
                      n869 = Enqueue Element(queue=w2710, element=w2708) -> (queue out=w2709:refnum<queue>)  [unwired: 2 in, 2 out]
                    }
                  }
                }
                n870 = Select(t=State_Type_Definitions,_for_0.26g_versions_and_later_2."True Stop" ("Enum"), s=w2689, f=State_Type_Definitions,_for_0.26g_versions_and_later_2."Task 9R: PROCESS COLOUR" ("Enum")) -> (s? t:f=w2692:T16)
                n871 = Select(t=w2692, s=w2690, f=State_Type_Definitions."Task 9Q: SCAN IMAGE" ("Enum")) -> (s? t:f=w2698:u16)
              }
              frame "Exit" {
                n872 = for {
                  shift-right: [w2717] -> w2714
                  shift-left: w2711 -> [w2718]
                  tunnel: string[] ["STOP", "RESET ENCODERS", "RESET YAW", ""] -> [w2716] mode=indexing
                  n873 = Enqueue Element(queue=w2718, element=w2716) -> (queue out=w2717:refnum<queue>)  [unwired: 2 in, 2 out]
                }
              }
            }
          }
          frame 55 {
            # ">> Item Selection Bias >>"
            # ">>> Motor control cluster >>>"
            # ">>> yStepper command>>>"
            n874 = Dequeue Element(queue=w2724, timeout in ms (-1)=w2725, error in (no error)=w2726) -> (element=w2728:T8)  [unwired: 3 out]
            n875 = case shown="\"Start Task 1\", Default" w2728 {
              tunnel: w2722 -> [w2734 _]
              tunnel: [w2741 State_Type_Definitions,_for_0.26g_versions_and_later_2."True Stop" ("Enum")] -> w2720
              tunnel: w2727 -> [w2733 _]
              tunnel: w2723 -> [w2740 w2757]
              tunnel: [w2739 w2758] -> w2719
              tunnel: [State_Type_Definitions,_for_0.26g_versions_and_later_2."Idle" ("Enum") State_Type_Definitions,_for_0.26g_versions_and_later_2."Shutdown" ("Enum")] -> w2721
              frame "Start Task 1", Default {
                n876 = case shown="False" w2734 {
                  tunnel: w2740 -> [w2744 w2751]
                  tunnel: [w2745 w2750] -> w2739
                  frame False {
                    n877 = for {
                      tunnel: string[] ["START TIMER", "COLOUR PROCESSING", ""] ("element") -> [w2746] mode=indexing
                      shift-right: [w2748] -> w2745
                      shift-left: w2744 -> [w2747]
                      n878 = Enqueue Element(queue=w2747, element=w2746) -> (queue out=w2748:refnum<queue>)  [unwired: 2 in, 2 out]
                    }
                  }
                  frame True {
                    n879 = for {
                      shift-right: [w2753] -> w2750
                      shift-left: w2751 -> [w2754]
                      tunnel: string[] ["CLOSE CAM", "DISPOSE BUFFERS", "RESET ENCODERS", "RESET YAW", "RESET FLAGS", ""] -> [w2752] mode=indexing
                      n880 = Enqueue Element(queue=w2754, element=w2752) -> (queue out=w2753:refnum<queue>)  [unwired: 2 in, 2 out]
                    }
                  }
                }
                n881 = Or(x=w2734, y=w2733) -> (x .or. y?=w2732:bool)
                n882 = Select(t=State_Type_Definitions,_for_0.26g_versions_and_later_2."True Stop" ("Enum"), s=w2733, f=State_Type_Definitions,_for_0.26g_versions_and_later_2."True Stop" ("Enum")) -> (s? t:f=w2735:T16)
                n883 = Select(t=w2735, s=w2732, f=State_Type_Definitions,_for_0.26g_versions_and_later_2."Task 9R: PROCESS COLOUR" ("Enum")) -> (s? t:f=w2741:T16)
              }
              frame "Exit" {
                n884 = for {
                  shift-right: [w2761] -> w2758
                  shift-left: w2757 -> [w2762]
                  tunnel: string[] ["STOP", "RESET ENCODERS", "RESET YAW", "ARDUINO MODE 0"] -> [w2760] mode=indexing
                  n885 = Enqueue Element(queue=w2762, element=w2760) -> (queue out=w2761:refnum<queue>)  [unwired: 2 in, 2 out]
                }
              }
            }
          }
        }
        "Object Detection" <- w300
        "Ultrasonic sensors" <- w323
        "Encoder values" <- w312
        "Stepper position values" <- w296
        "NAVX Values" <- w294
        "Time up" <- w292
        "IR Sensors" <- w286
        "Line sensors" <- w281
      }
    }
    "Object recognition mode" <- w212
    n886 = local write "Green LED"(w222) -> ()
  }
  n887 = while {
    stop <- w3525 stop-if-true
    n888 = call "MOTOR CONTROL WITH PID AE.vi"("AE Mode"=MOTOR_CONTROL_WITH_PID_AE_DATA_MODE_TYPE_DEF."Read from AE") -> ("Speed & distance"=→"Speed & distance":T13)  [unwired: 3 in]
    n889 = call "FGV Bool.vi"("Init/Read/Write State"=States_for_Action_Engine."Read") -> ("Output node"=w3525:bool)  [unwired: 2 in, 1 out]
    n890 = Wait (ms)(milliseconds to wait=u32 5) -> ()  [unwired: 1 out]
  }
  n891 = call <vilib>:"DIO Close.vi"("error in (no error)"=w22, "DIO Info In"=w25) -> ()  [unwired: 9 in, 1 out]
  n892 = call <vilib>:"DIO Close.vi"("error in (no error)"=w32, "DIO Info In"=w34) -> ()  [unwired: 9 in, 1 out]
  n893 = call <vilib>:"NavX Close.vi"("error in (no error)"=w9, "NavX Info In"=w8) -> ()  [unwired: 9 in, 1 out]
  n894 = call <vilib>:"DIO Close.vi"("error in (no error)"=w27, "DIO Info In"=w29) -> ()  [unwired: 9 in, 1 out]
  n895 = call <vilib>:"DIO Close.vi"("error in (no error)"=w16, "DIO Info In"=w17) -> ()  [unwired: 9 in, 1 out]
  n896 = call <vilib>:"DIO Close.vi"("error in (no error)"=w11, "DIO Info In"=w12) -> ()  [unwired: 9 in, 1 out]
  n897 = Merge Errors "Merge Errors"(w62, w61) -> (w44:errorcluster)
  n898 = Merge Errors(w48, w44) -> (w43:errorcluster)
  n899 = Destroy User Event(user event=w66, error in=w43) -> ()  [unwired: 1 out]
  n900 = Release Queue(queue=w39, error in (no error)=w43) -> (error out=→"Queue Errors":errorcluster)  [unwired: 1 in, 2 out]
  n901 = Release Queue(queue=w56, error in (no error)=w43) -> ()  [unwired: 1 in, 3 out]
  n902 = Destroy User Event(user event=w65, error in=w43) -> ()  [unwired: 1 out]
  n903 = Unregister For Events(event registration refnum=w57, error in=w43) -> ()  [unwired: 1 out]
